vi "Version1z.vi"() -> ()   [LabVIEW 2019]
doc: "This is the interface, the one VI which loads all the others. Run this one first.\n\n(the line below ensures settings are saved)\n[Red Tweezers Save Settings]"
uses:
  plugins/subvis/line_trapping.ctl
  plugins/subvis/spot.ctl
  <vilib>/userDefined/High Color/IMAQdx.ctl
  plugins/subvis/selection_element.ctl
  <vilib>/Analysis/Matrix/Datatypes/RealMatrix.ctl
  plugins/subvis/mouse_info.ctl
  <vilib>/Analysis/baseanly.llb/Real A x B.vi
  plugins/subvis/red_tweezers_globals_INTERNAL_VOLATILE.vi
  plugins/subvis/red_tweezers_globals.vi
  <vilib>/Analysis/Matrix/Numeric/Multiply/Multiply - RM,R.vi
  <vilib>/Analysis/NI_AALBase.lvlib
  <vilib>/vision/driver/NI_Vision_Acquisition_Software.lvlib
  <vilib>/vision/NI_Vision_Development_Module.lvlib
  <vilib>/Analysis/Matrix/NI_Matrix.lvlib
panel:
  out "Objects":T1(array[cluster]) {"Aspect Ratio" format="%.2f"; "Orientation" format="%.2f"; "Area" format="%.2f"; "Object Center"."Y" format="%.2f"; "Object Center"."X" format="%.2f"}
  out "Specific Point 2":cluster{i32, i32}
  out "Specific Point":cluster{i32, i32}
  out "bottomrx 3":dbl
  out "toply 3":dbl
  out "bottomry 3":dbl
  out "toplx 3":dbl
  out "Circles 2":T2(array[cluster]) {"Position"."Y" format="%.2f"; "Position"."X" format="%.2f"}
  out "Spot Storage":T3[](array[typedef]) {"Amplitude Correction" step=0.1; "Line Trapping"."Phase Gradient" step=0.05; "Line Trapping"."Vector"."x" step=1e-06 format="%#_6p"; "Line Trapping"."Vector"."y" step=1e-06 format="%#_6p"; "Line Trapping"."Vector"."z" step=1e-06 format="%#_6p"; "NA Position"."r" step=1e-06; "NA Position"."y" step=1e-06; "NA Position"."x" step=1e-06; "Position"."z" step=1e-06; "Position"."y" step=1e-06; "Position"."x" step=1e-06; "Phase" step=0.7753; "Intensity" step=0.1}
  out "# selected":i16
  out "Last Pattern":T3[](array[typedef]) {"Amplitude Correction" step=0.1; "Line Trapping"."Phase Gradient" step=0.05; "Line Trapping"."Vector"."x" step=1e-06 format="%#_6p"; "Line Trapping"."Vector"."y" step=1e-06 format="%#_6p"; "Line Trapping"."Vector"."z" step=1e-06 format="%#_6p"; "NA Position"."r" step=1e-06; "NA Position"."y" step=1e-06; "NA Position"."x" step=1e-06; "Position"."z" step=1e-06; "Position"."y" step=1e-06; "Position"."x" step=1e-06; "Phase" step=0.7753; "Intensity" step=0.1}
  out "Plugins":T5(array[cluster])=[{"Name"="ASI Stage", "Folder"=path "C:/Users/Richard Bowman/Dropbox/red_tweezers_1_4_rc4/plugins/ASI Stage.llb", "vi reference"=refnum, "Needs to be run"=TRUE, "Error"={"status"=FALSE, "code"=0, "source"=""}}, {"Name"="iTweezers", "Folder"=path "C:/Users/Richard Bowman/Dropbox/red_tweezers_1_4_rc4/plugins/iTweezers.llb", "vi reference"=refnum, "Needs to be run"=TRUE, "Error"={"status"=FALSE, "code"=0, "source"=""}}, {"Name"="MightexLED", "Folder"=path "C:/Users/Richard Bowman/Dropbox/red_tweezers_1_4_rc4/plugins/MightexLED.llb", "vi reference"=refnum, "Needs to be run"=TRUE, "Error"={"status"=FALSE, "code"=0, "source"=""}}]
  in  "Tab":T6(tab)
  out "Object MP Y":dbl
  out "Object MP X":dbl
  out "ROI Point 3":T7
  out "Numeric 3":dbl
  out "Numeric 2":dbl
  in  "ROI points":dbl
  out "ROI Y":dbl
  out "ROI X":dbl
  out "Center Y":dbl
  out "Center X":dbl
  in  "Camera Capture 2":bool
  out "Bubble y 2":dbl
  out "Bubble x 2":dbl
  out "Number of Matches Returned":dbl
  out "bottomry 2":dbl
  out "toply 2":dbl
  out "bottomrx 2":dbl
  out "toplx 2":dbl
  in  "Send Data":bool
  out "Camera 3":T8(plugin-control)
  in  "Circle Descriptor 2":cluster{"Min Radius":dbl, "Max Radius":dbl}={"Min Radius"=3.0, "Max Radius"=500.0}
  out "Radius":dbl
  in  "Settings":T9={"Objects"=0, "Threshold"=128, "Reject Border"=FALSE, "Fill Holes"=FALSE, "Min Object Size"=FALSE, "Min Size"=3, "Max Object Size"=FALSE, "Max Size"=100, "Show Search Area"=FALSE, "Show Center"=TRUE, "Show Bounding Box"=TRUE} {"Objects" items=["Bright Objects", "Dark Objects"]; "Threshold" min=1 max=999999999 step=1; "Max Size" min=1 max=999999999 step=1; "Min Size" min=1 max=999999999 step=1}
  out "Number of Objects":i32
  in  "ROI switch":bool
  out "# of pairs":dbl
  out "1spot X":dbl
  out "1spot Y":dbl
  out "2spot X":dbl
  out "2spot Y":dbl
  out "NewX1":dbl
  out "NewY1":dbl
  out "NewX2":dbl
  out "NewY2":dbl
  out "Step Calculation X1":dbl
  out "Step Calculation Y1":dbl
  out "Step Calculation X2":dbl
  out "Step Calculation Y2":dbl
  out "Possible Collision":bool
  out "Play Pressed":bool
  out "Y":dbl
  out "X":dbl
  in  "O Button":bool
  in  "OK Button":bool
  in  "Bubble Size":dbl=50.0002
  out "Hit Indicator":bool
  in  "On":bool
  out "Induce check":bool
  out "Area+ Buffer":dbl
  in  "Area to check":dbl=0.00025
  out "Prev Current Spot":dbl
  out "spots selected 2":i32=4
  out "Spot # Check":dbl
  out "Orig Y SC":dbl
  out "Orig X SC":dbl
  out "ID num check":dbl
  out "Value Check":dbl
  out "ID":dbl[](array[numeric])
  out "Null array":dbl[](array[numeric])
  out "Potential Collisions":dbl
  out "What to Check":dbl[](array[numeric])
  out "Num":dbl
  out "Old Y":dbl
  out "Old X":dbl
  out "init":dbl
  out "Looper":bool
  in  "Output to SLM":bool
  out "Maximum":dbl
  out "Projected Distance":dbl
  out "Previous Distance":dbl
  out "Group ID #":dbl
  in  "Buffer Zone":dbl=7e-05
  out "# of Spots":dbl
  out "Distance":dbl
  out "Hit":bool
  out "Y Displacement":dbl
  out "X Displacement":dbl
  out "Current Spot #":dbl
  out "spots selected":i32=4
  in  "lock aspect ratio":bool=TRUE
  in  "Size":cluster{"x":dbl, "y":dbl, "z":dbl} {"z" step=1e-06 format="%#_4p"; "y" step=1e-06 format="%#_4p"; "x" step=1e-06 format="%#_4p"}
  in  "Position":cluster{"x":dbl, "y":dbl, "z":dbl}={"x"=1e-06, "y"=-6.3e-06, "z"=0.0} {"z" step=1e-06 format="%#_4p"; "y" step=1e-06 format="%#_4p"; "x" step=1e-06 format="%#_4p"}
  in  "phase":dbl step=0.7753
  in  "Vortex Charge":i8
  in  "Intensity":dbl=1.0 step=0.1
  in  "add to selection":bool
  in  "random position":bool
  in  "new spot":bool
  in  "delete":bool
  in  "New location\n ROI":bool
  out "Radius ROI x6":dbl
  out "Radius ROI y6":dbl
  out "Radius ROI y5":dbl
  out "Radius ROI x5":dbl
  out "Radius ROI y4":dbl
  out "Radius ROI x4":dbl
  out "Radius ROI y3":dbl
  out "Radius ROI x3":dbl
  out "Radius ROI x2":dbl
  out "Radius ROI y2":dbl
  out "Radius ROI y1":dbl
  out "Radius ROI x1":dbl
  out "Caging Radius \nToo Big":bool
  in  "Caging Radius":dbl
  out "ROI Point 1":T7
  out "ROI Point 0":T7
  out "ROI Point 2":T7
  in  "New Center Y":dbl
  in  "New Center X":dbl
  out "Delta x":dbl[](array[numeric])
  out "Delta y":dbl[](array[numeric])
  in  "Input New \nObject Location":bool
  out "Time Elapsed(ms)":i32
  out "Start":i32
  out "Stop":i32
  out "Insert End":bool
  out "NewXYRates":dbl[][](array[numeric])
  out "NewXYArraySize":dbl
  out "NewXYArray":dbl[][](array[numeric])
  in  "Rates":dbl
  out "LCS Y":dbl
  out "LCS X":dbl
  in  "LCS":dbl
  in  "Play":bool
  out "Initiate Creation":dbl
  in  "Max Number \nof Bubbles":dbl
  in  "Number of Planned\nSequence Frames":dbl
  in  "Add Additional Frames":bool
  in  "Frame Location":dbl
  in  "Additional Frames Wanted":dbl
  in  "rotate":bool
  in  "Rotation Axis":u16(ring)=2 items=["Z", "X", "Y", "Custom"]
  in  "Angle (degrees)":dbl=2.0
  in  "Custom Axis":cluster{dbl, dbl, dbl}
  in  "Spot Shape":enum32{"Normal", "Line", "NA", "Mixed"}(tab)=enum."Mixed"
  in  "Line Trapping":T4 {"Phase Gradient" step=0.05; "Vector"."x" step=1e-06 format="%#_4p"; "Vector"."y" step=1e-06 format="%#_4p"; "Vector"."z" step=1e-06 format="%#_4p"}
  in  "Scale back aperture":dbl=1.1 step=0.1
  in  "Scale BA":bool
  in  "Position on back aperture":cluster{"x":dbl, "y":dbl}={"x"=-5.84327907697451e-18, "y"=0.0} {"y" step=0.1 format="%#_4p"; "x" step=0.1 format="%#_4p"}
  in  "Radius on back aperture":dbl=1.1 step=0.1
  in  "Generate":bool
  in  "Pattern":T10(tab)
  in  "Spots across centre":i32=5
  in  "Reference Array?":bool
  in  "Fraction of SLM":dbl=1.0
  in  "Spots across centre":i32=5
  in  "N":cluster{i32, i32}
  in  "spacing/m":dbl=2.0
  in  "Iterations":i32=10
  out "non-uniformity":dbl(slide)=0.031119223416512406 scale=0.0..0.2
  out "efficiency":dbl(slide)=0.8985936267644501 scale=0.0..1.0
  in  "Optimise":bool
  in  "Reset Phase/Amplitude":bool
  in  "Fall-off/m":dbl=0.00025 min=0.0 step=1e-06 format="%#_4p"
  in  "Abort Plugin":bool
  in  "Plugin:":u16(ring)=1
  in  "Save Video":bool
  in  "Global ROI (requires restart)":i32[](array[numeric])=[0, 0, 1280, 512]
  in  "Zoom":bool
  in  "Draw ROI":bool
  in  "Zoom to Fit":bool
  out "Image Information":string="640x480 1.93X 8-bit image 255    (0,0)"
  in  "Camera":T11
  in  "Time per Frame (ms)":dbl
  in  "Edit Sequence Mode":bool
  in  "Manual Edit":bool
  in  "Bubble ID to Empty":dbl
  in  "Clearance Button":bool
  in  "Manual Sequence":bool
  in  "Play Sequence":bool
  in  "Reset":bool
  out "Sequence Instances":dbl
  out "Counter":dbl
  in  "Save State":bool
  out "Sequence On?":bool
  in  "Sequence Order":dbl
  out "Selection/Group":T12[](array[typedef])
  in  "Sequence Storer":T3[][](array[typedef]) {"Amplitude Correction" step=0.1; "Line Trapping"."Phase Gradient" step=0.05; "Line Trapping"."Vector"."x" step=1e-06 format="%#_6p"; "Line Trapping"."Vector"."y" step=1e-06 format="%#_6p"; "Line Trapping"."Vector"."z" step=1e-06 format="%#_6p"; "NA Position"."r" step=1e-06; "NA Position"."y" step=1e-06; "NA Position"."x" step=1e-06; "Position"."z" step=1e-06; "Position"."y" step=1e-06; "Position"."x" step=1e-06; "Phase" step=0.7753; "Intensity" step=0.1}
  in  "Tab Control":enum32{"Line", "Arc"}(tab)
  out "X Rate":dbl
  out "Y Rate":dbl
  out "Degree Rate":dbl
  out "Radians":dbl
  out "Center Y":dbl
  out "Center X":dbl
  in  "Radius X":dbl
  in  "Theta":dbl
  in  "Lock Current Spot":bool
  out "Locked Current Spot":dbl
  out "Numeric":dbl
  out "probe":dbl
  in  "Insert":bool
  in  "Start at Which Frame?":dbl
  out "Original Y":dbl
  out "Original X":dbl
  in  "Mark Original Position":bool
  in  "How Many Frames?":dbl
  out "New Y":dbl
  out "New X":dbl
  out "Spot Storage 2":T3[](array[typedef]) {"Amplitude Correction" step=0.1; "Line Trapping"."Phase Gradient" step=0.05; "Line Trapping"."Vector"."x" step=1e-06 format="%#_6p"; "Line Trapping"."Vector"."y" step=1e-06 format="%#_6p"; "Line Trapping"."Vector"."z" step=1e-06 format="%#_6p"; "NA Position"."r" step=1e-06; "NA Position"."y" step=1e-06; "NA Position"."x" step=1e-06; "Position"."z" step=1e-06; "Position"."y" step=1e-06; "Position"."x" step=1e-06; "Phase" step=0.7753; "Intensity" step=0.1}
  in  "Save":bool
  in  "Load":bool
  out "Video Frame Rate":dbl(knob)=50.00000000000003 scale=0.0..100.0 scale format="%.1f"
  out "Interface Frame Rate":dbl(knob)=97.23240312927678 scale=0.0..100.0 scale format="%.1f"
  in  "stop":bool=TRUE
  in  "Spots":dbl
  out "ROI new MPx":dbl
  out "ROI new Mpy":dbl
  out "3spot Y":dbl
  out "3spot X":dbl
  out "ROI y6":dbl
  out "ROI x6":dbl
  out "ROI y5":dbl
  out "ROI x5":dbl
  out "ROI y4":dbl
  out "ROI x4":dbl
  out "ROI y3":dbl
  out "ROI x3":dbl
  out "ROI y2":dbl
  out "ROI x2":dbl
  out "ROI y1":dbl
  out "ROI x1":dbl
  out "ROI Point 6":T7
  out "ROI point 5":T7
  out "ROI Point 4":T7
  out "MOP pressed":bool
  out "MOP pressed After":bool
  out "X Pos every 10 sec":dbl
  out "Elapsed Time":dbl
  out "Position Indicator":string
  out "Spot Checker":T3[](array[typedef]) {"Amplitude Correction" step=0.1; "Line Trapping"."Phase Gradient" step=0.05; "Line Trapping"."Vector"."x" step=1e-06 format="%#_6p"; "Line Trapping"."Vector"."y" step=1e-06 format="%#_6p"; "Line Trapping"."Vector"."z" step=1e-06 format="%#_6p"; "NA Position"."r" step=1e-06; "NA Position"."y" step=1e-06; "NA Position"."x" step=1e-06; "Position"."z" step=1e-06; "Position"."y" step=1e-06; "Position"."x" step=1e-06; "Phase" step=0.7753; "Intensity" step=0.1}
  out "Image":T8(plugin-control)
  # "Notes:\n\nIf you are doing non-sequence controls,\nthe delete function can be used as intended.\nHowever, do not use the delete function after\nrunning a sequence! Using it will prevent\nthe bubbles from appearing as the\nnumber of spots will change, which is\nessential for the sequence to work (it would\nbe displaying the maximum number of\nbubbles). \n\nIf you happen to delete a bubble, it can be \nrestored by inserting a new spot. Once enough\nspots have been restored, click on manual edit\nto correct the # of spots tracker. It should \nbe restored to where it originally was."
  # "The SLM can be used to shape spots; here you can restrict the NA of a spot (so it comes only from part of the back aperture), or create a line-trap"
  # "The traps do not have any spot-shaping applied (so they should just be diffraction-limited focal spots)."
  # "This shapes the amplitude (and phase) of the beam to create extended line traps.  The \"Phase Gradient\" control allows the Poynting vector to push things along the line.  Unfortunately, some work is needed on the scaling factors so the phase gradient control will need tweaking if the line trap has a nonzero z component."
  # "By default,each spot comes from the whole back aperture.  Here, you can limit a spot to come from a specific part of the back aperture."
  # "The control below allows you to scale the whole back aperture (i.e. the position and size of all the apertures).  It's a one-time operation, i.e. only changes things when you push \"ok\"."
  # "A Combination of line-trapping and NA restriction has been applied to these traps.  You can get at the line trap or NA parameters on the other tabs, switching to the NA tab does not delete the line-trap settings."
  # "This tab generates Shack-Hartmann type holograms, which are often useful when aligning the system, and arrays of spots."
  # "The controls above only work when using the \"IMAQdx with ROI Buttons\" case in the bottom loop.  You can save video regardless of camera code though."
  # "Manual Edit allows a user to\ngo to a specific sequence frame."
  # "To clear the sequence, you must\nclear the array. Right click on sequence\nstorer to do this."
  # "Use this to \"clear\" a \nspecific bubble. If\nworking on a sequence,\nuse this as your delete\nbutton! You can update\nthe view by using manual edit."
  # "Use the reset button\nto clear counter.\nIt becomes necessary\nwhen you clear the array,\nespecially in manual mode."
  # "Use the sequence creator tab to specify the\nnumber of bubbles you want along with\nthe number of frames.\n\nTo save at a specific interval, the sequence\norder can be used to place the state. If used\nto correct something, it will replace the\nentire sequence frame.\n\n\"Sequence On?\" is only used in auto mode."
  # "Multiple bubbles can  be done with the\nline function. One bubble at a time for the arc\nfunction."
  # "Using the Load/Save function:\n\nRed Tweezers itself is unable to save long \nsequences, but a separate program is able to\naccomplish this. To do this, follow these\nsteps:\n\n1. After creating your sequence, press the save\nbutton below.\n\n2. Then, go to the subvi folder and find\nSequenceSaver.vi.\n\n3. At the control \"Sequence Storer,\" right-click\nthe dimensions part of the array and go to\ndata operations.\n\n4. Press \"Make Current Values Default\" and save\nthe sequence.\n\n5. The next time you load the program, simply\npress load to re-acquire the sequence. You\nwill need to insert the bubbles again, but after\nthe first frame can be recovered by using\nSequenceControl.vi."
types:
  T1 = cluster{"Object Center":cluster{"X":sgl, "Y":sgl}, "Bounding Box":cluster{"X Left":i32, "Y Top":i32, "X Right":i32, "Y Bottom":i32}, "Area":sgl, "Orientation":sgl, "Aspect Ratio":sgl, "Nb Holes":i32}[]
  T2 = cluster{"Position":cluster{"X":sgl, "Y":sgl}, "Radius":dbl, "Score":dbl}[]
  T3 = typedef "spot.ctl" = cluster{"Position":cluster{"x":dbl, "y":dbl, "z":dbl}, "Intensity":dbl, "Vortex Charge":i8, "Phase":dbl, "NA Position":cluster{"x":dbl, "y":dbl, "r":dbl}, "Line Trapping":T4, "Amplitude Correction":dbl}
  T4 = typedef "line_trapping.ctl" = cluster{"Vector":cluster{"x":dbl, "y":dbl, "z":dbl}, "Phase Gradient":dbl}
  T5 = cluster{"Name":string, "Folder":path, "vi reference":refnum<vi>, "Needs to be run":bool, "Error":errorcluster}[]
  T6 = enum32{"Image Process", "Current Spot", "Sequence Creator", "Rotate", "Spot Shape", "Patterns", "Plugins", "Video", "Sequence", "Spot Control", "Load/Save"}
  T7 = typedef "NI_Matrix.lvlib/RealMatrix.ctl" = dbl[][]
  T8 = typedef "IMAQ Image.ctl" = refnum<image>
  T9 = cluster{"Objects":u16, "Threshold":i32, "Reject Border":bool, "Fill Holes":bool, "Min Object Size":bool, "Min Size":i32, "Max Object Size":bool, "Max Size":i32, "Show Search Area":bool, "Show Center":bool, "Show Bounding Box":bool}
  T10 = enum32{"HCP Shack-Hartmann", "Square Shack-Hartmann", "Rectangular Grid"}
  T11 = typedef "IMAQdx.ctl" = refnum<k21>
  T12 = typedef "selection_element.ctl" = cluster{"Group ID":i32, "Selected":bool}
  T13 = typedef "mouse_info.ctl" = cluster{"Button Down":bool, "Dragging":bool, "Position (Image Pixels)":cluster{"X":dbl, "Y":dbl}, "Previous Position (Image Pixels)":cluster{"X":dbl, "Y":dbl}, "Button":u16, "Mods":cluster{"Double Click":bool, "Menu Key":bool}, "PlatMods":cluster{"Shift":bool, "Ctrl":bool, "Alt":bool, "Cmd":bool, "Opt":bool}}
  T14 = cluster{"Desired Font (Application)":enum16{"User-specified Font", "Application Font", "System Font", "Dialog Font"}, "[User-specified Font]":cluster{"Font Name":string, "Size":i16, "Strikeout?":bool, "Italic?":bool, "Underline?":bool, "Outline?":bool, "Shadow?":bool, "Bold?":bool, "Rotation Angle":dbl}, "Horizontal Alignment":i16, "Vertical Alignment":i16}
  T15 = cluster{"Position":cluster{"x":dbl, "y":dbl, "z":dbl}, "Intensity":dbl, "Vortex Charge":i8, "Phase":dbl, "NA Position":cluster{"x":dbl, "y":dbl, "r":dbl}, "Line Trapping":T4, "Amplitude Correction":dbl}
  T16 = enum16{"Set guide visibility", "Set grid visibility", "Show front panel", "Render on image"}
  T17 = enum32{"Current Spot", "Rotate", "Spot Shape", "Patterns", "Plugins", "Video"}
  T18 = enum16{"Left Button", "Center Button", "Right Button", "Window Close"}
  T19 = typedef "Image Type" = u32
  T20 = cluster{"number: 0 to 1":dbl, "number: 0 to 1":dbl}
  T21 = typedef "overlay_element.ctl" = cluster{"Tool":enum16{"Lines", "Oval", "Rectangle", "Text"}, "Points":cluster{"X":dbl, "Y":dbl}[], "Drawing Mode":u32, "Color":u32, "String":string}
  T22 = enum32{"Current Spot", "Rotate", "Spot Shape", "Patterns", "Plugins", "Video", "Particle Tracking", "Clamping", "Blank"}[]
  T23 = typedef "LVMenuShortCut.ctl" = cluster{"include Shift key?":bool, "include Ctrl key?":bool, "shortcut key":string}
  T24 = typedef "LVPoint32TypeDef.ctl" = cluster{"Horizontal":i32, "Vertical":i32}
  T25 = cluster{"Shift":bool, "Ctrl":bool, "Alt":bool, "Cmd":bool, "Opt":bool}
  T26 = cluster{"Button Down":bool, "Dragging":bool, "Mouse Coords (image pixels)":cluster{dbl, dbl}, "Mouse Coords (image pixels)":cluster{dbl, dbl}, "Button":u16, "Mods":cluster{"Double Click":bool, "Menu Key":bool}, "PlatMods":cluster{"Shift":bool, "Ctrl":bool, "Alt":bool, "Cmd":bool, "Opt":bool}}
  T27 = cluster{"Global Rectangle":i32[], "Contours":cluster{"Contour Type":u32, "ROI Type":u32, "Points":i32[]}[]}
  T28 = cluster{"Contour Type":u32, "ROI Type":u32, "Points":i32[]}[]
  T29 = cluster{"Position":cluster{"X":sgl, "Y":sgl}, "Radius":dbl, "Score":dbl}
  T30 = cluster{"Contour Type":u32, "ROI Type":u32, "Points":i32[]}
  T31 = cluster{"[0]":dbl, "[1]":dbl, "[2]":dbl, "[3]":dbl}
  T32 = cluster{"Object Center":cluster{"X":sgl, "Y":sgl}, "Bounding Box":cluster{"X Left":i32, "Y Top":i32, "X Right":i32, "Y Bottom":i32}, "Area":sgl, "Orientation":sgl, "Aspect Ratio":sgl, "Nb Holes":i32}
  T33 = cluster{"NewXYArray[0]":dbl, "NewXYArray[1]":dbl, "NewXYArray[2]":dbl, "NewXYArray[3]":dbl, "NewXYArray[4]":dbl, "NewXYArray[5]":dbl, "NewXYArray[6]":dbl, "NewXYArray[7]":dbl, "NewXYArray[8]":dbl}
  T34 = cluster{"Average Frame Time":dbl, "millisecond timer value":u32}
  T35 = cluster{"Position":cluster{"x":dbl, "y":dbl, "z":dbl}, "Intensity":dbl, "Vortex Charge":i8, "Phase":dbl, "NA Position":cluster{"x":dbl, "y":dbl, "r":dbl}, "Line Trapping":T4, "Amplitude Correction":dbl}[]
  T36 = enum32{"Bad", "Idle", "Run top level", "Running"}
  T37 = typedef "AviRefnum.ctl" = refnum<k1>
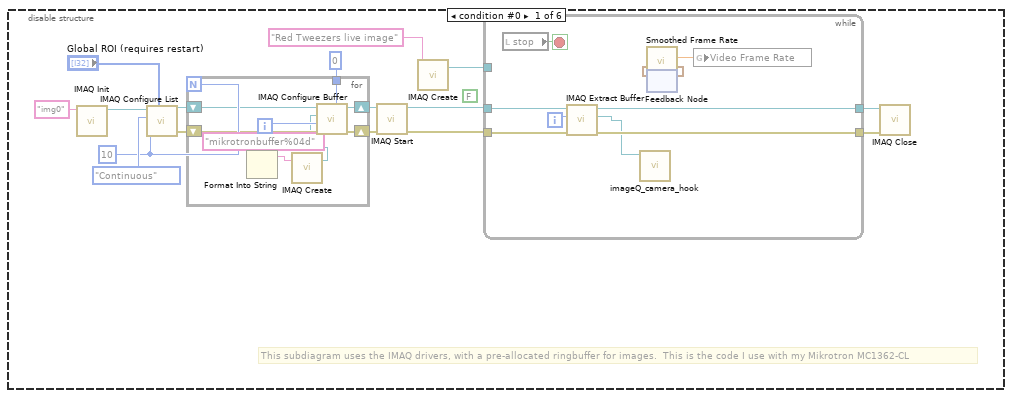
[diagram p3: hidden frame]
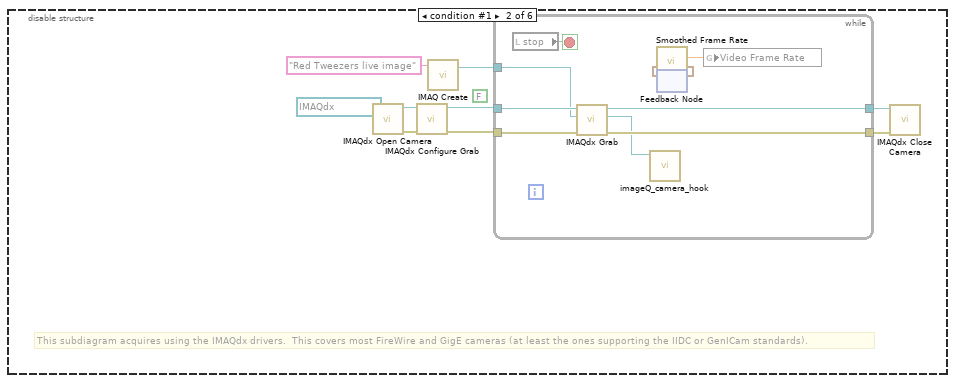
[diagram p4: hidden frame]
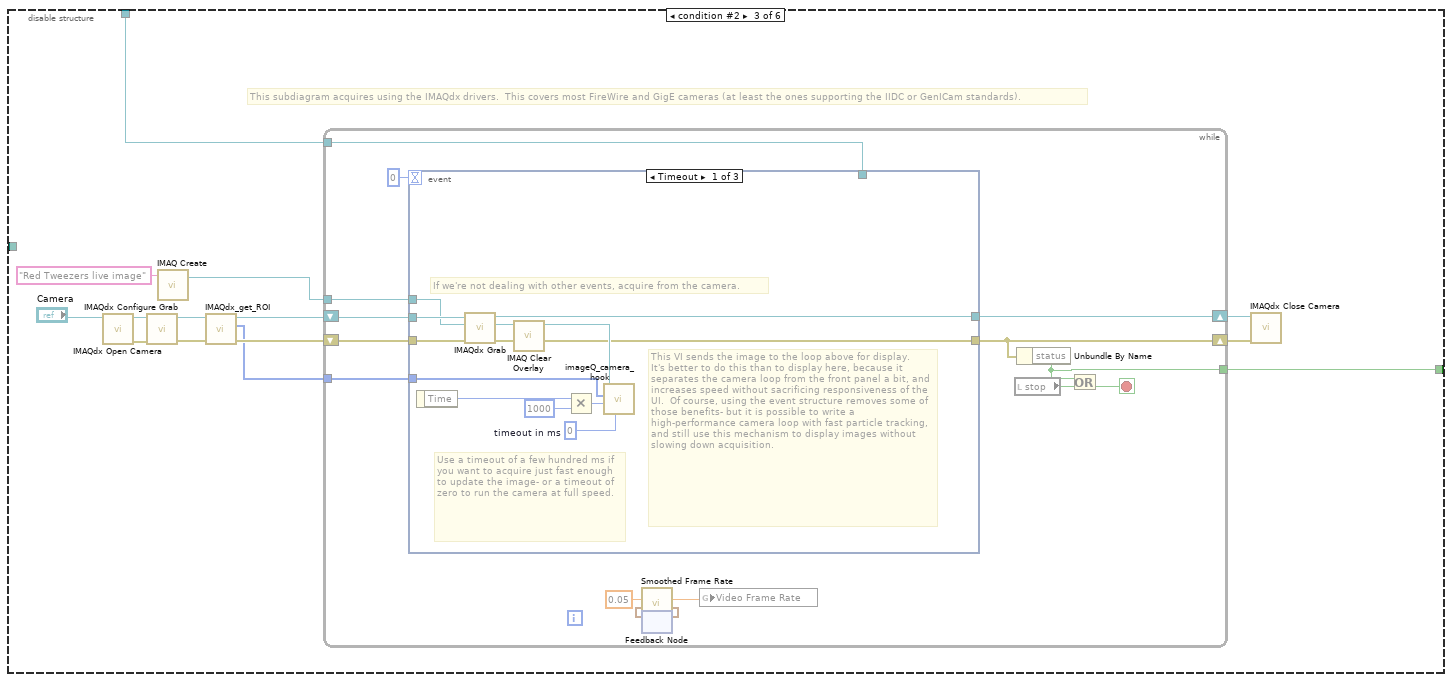
[diagram p5: hidden frame]
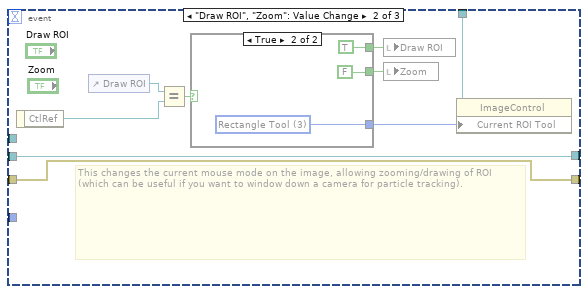
[diagram p6: hidden frame]
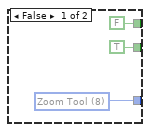
[diagram p7: hidden frame]
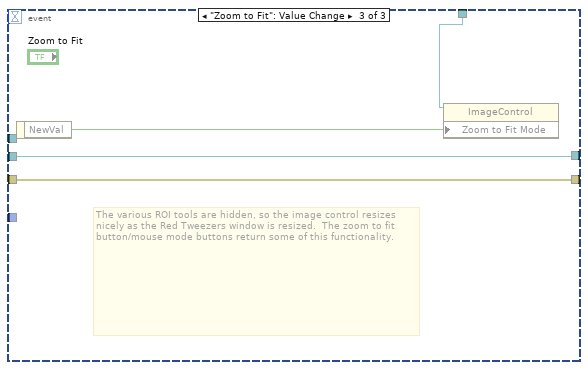
[diagram p8: hidden frame]
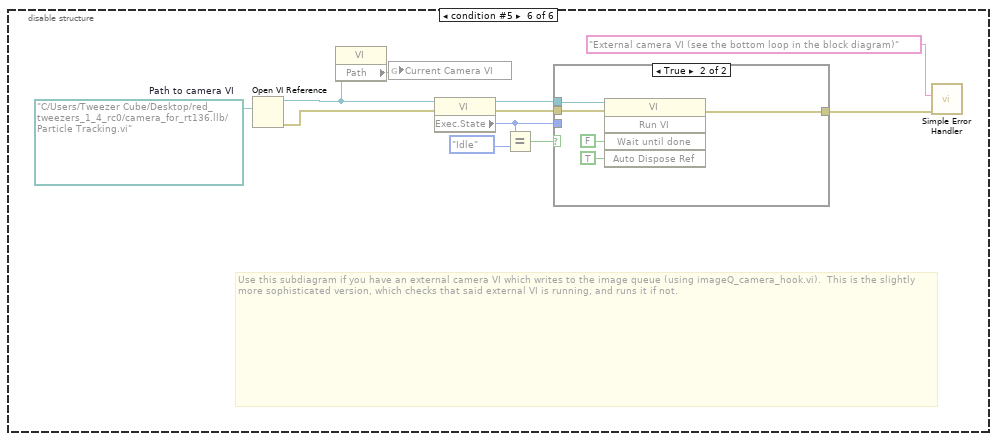
[diagram p10: hidden frame]
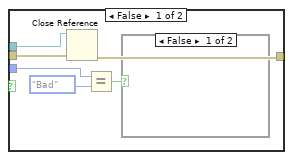
[diagram p11: hidden frame]
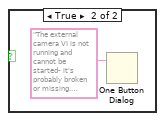
[diagram p12: hidden frame]
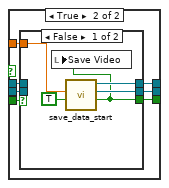
[diagram p14: hidden frame]
diagram:
  w11 = "red_tweezers_display_imageQ" ("Queue Name")
  w23 = T13 {"Button Down"=FALSE, "Dragging"=FALSE, "Position (Image Pixels)"={"X"=0.0, "Y"=0.0}, "Previous Position (Image Pixels)"={"X"=0.0, "Y"=0.0}, "Button"=0, "Mods"={"Double Click"=FALSE, "Menu Key"=FALSE}, "PlatMods"={"Shift"=FALSE, "Ctrl"=FALSE, "Alt"=FALSE, "Cmd"=FALSE, "Opt"=FALSE}}  # Mouse Information
  w24 = refnum<vi> refnum  # Image
  # "The funny looking feedback-node structure is deliberate (if odd).  We want to reload settings from the last used file (stored in the registry) only if this program has not been run since it was last loaded from file/recompiled.  That's why I use an uninitialised shift register: every time the program runs, it increments.  So, if it is zero, this is our first run (or we've been recently recompiled)."
  # "This loop handles the video that is displayed on-screen and saved to file."
  # "Initially, we only register to be told when the user clicks the image"
  # "This is the actual image control"
  # "This is a generic reference.\nIt is just a placeholder, so we can register for events later."
  # "This version of red tweezers uses two coordinate systems: \n1. Real Coordinates - corresponding to physical distances in 3D in microns\n2. Image Coordinates - position on the camera image, relative to the top left of the CURRENT ROI, measured in pixels. If the ROI changes, the relationship between \"real units\" and \"image pixels\" may change, so all values should be stored and presented to the user in REAL units unless there is a good reason to do otherwise."
  n1 = control-ref of="Plugin Pnl"() -> (w20:refnum<vi>)
  n2 = flat-sequence {
    tunnel: [w27] -> w6
    tunnel: w4 -> [_]
    frame #0 {
      n3 = vi-ref "red_tweezers_globals_INTERNAL.vi"() -> (w28:refnum<vi>)
      n4 = property class="VI"(reference=w28) -> ("Path"=w27:path)  [unwired: 1 in, 2 out]
      n5 = global write "red_tweezers_globals_INTERNAL_VOLATILE.vi" "Current Camera VI"(w27) -> ()
    }
  }
  n6 = control-ref of="Plugin:"() -> (w21:refnum<vi>)
  n7 = feedback #1() -> (w14:dbl)  [unwired: 1 in]
  n8 = Equal To 0?(x=w14) -> (x = 0?=w13:bool)
  n9 = Increment(x=w14) -> (x+1=w12:dbl)
  n10 = feedback-in #1(w12) -> ()
  n11 = call "plugins_load.vi"("Sub Panel"=w20, "Plugin Chooser"=w21) -> ("error out"=w15:errorcluster, "Plugins"=w17:T5)  [unwired: 2 in, 2 out]
  "Plugins" <- w17
  n12 = control-ref of="Image"() -> (w5:refnum<vi>)
  n13 = case shown="True" w13 {
    tunnel: w15 -> [_ w29]
    tunnel: [_ w29] -> w4
    frame False {
    }
    frame True {
      n14 = call "settings_load_default_file.vi"("error out"=w29) -> ()
    }
  }
  n15 = flat-sequence {
    tunnel: w4 -> [_]
    tunnel: w2 -> [w31]
    frame #0 {
      # "ensure we don't accidentally start saving video, and run UDP Sender to set up the hologram window."
      n16 = local write "Save Video"(FALSE ("background subtraction")) -> ()
      n17 = call "UDP Sender generic_2.vi"("Spots"=w31) -> ()  [unwired: 2 in, 1 out]
    }
  }
  n18 = global read "red_tweezers_globals.vi" "Selection/Group"() -> (w22:T12[])
  n19 = register-events(w5, w24, w24, w24) -> (reference out=w25:refnum<event-registration>)  [unwired: 2 in, 1 out]
  n20 = global read "red_tweezers_globals.vi" "Spots"() -> (w2:T3[])
  n21 = local write "stop"(FALSE ("STOP")) -> ()
  n22 = call "ensure_selection_matches_spots.vi"("Selection and Groups in"=w22, "Spots"=w2) -> ("Selection and Groups out"=w26:T12[], "Spots (duplicate)"=w1:T3[])  [unwired: 4 in]
  n23 = call "IMAQ Create"("Image Name"=w11) -> ("New Image"=w9:T8)  [unwired: 4 in, 1 out]
  n24 = call "imageQ_create_return_queue.vi"("Queue Name"=w11) -> ("queue out"=w10:refnum<queue>)
  n25 = while {
    shift-right: [w170] -> _
    shift-left: w1 -> [w190]
    shift-right: [w189] -> _
    shift-left: w26 -> [w188]
    shift-right: [w192] -> _
    shift-left: _ -> [w183]
    shift-right: [w191] -> _
    shift-left: _ -> [w182]
    tunnel: w5 -> [w187]
    shift-right: [w181] -> _
    shift-left: w23 -> [w180]
    shift-right: [w184] -> _
    shift-left: w25 -> [w185]
    border: errorcluster {"status"=FALSE, "code"=0, "source"=""} ("error out") -> [_]
    tunnel: [errorcluster {"status"=FALSE, "code"=0, "source"=""} ("error in (no error)")] -> w18
    border: w17 -> [_]
    tunnel: w1 -> [w171]
    stop <- w172 stop-if-true
    (unwired) 1 ("index")
    w88 = 7 items=["Red", "Green", "Blue", "Hue", "Saturation", "Luminance", "Value", "Intensity"] ("Color Plane")
    w90 = T19 0 items=["Grayscale (U8)", "Grayscale (I16)", "Grayscale (SGL)", "Complex (CSG)", "RGB (U32)", "HSL (U32)", "RGB (U64)", "Grayscale (U16)"] ("Image Type")
    # "Collision Avoidance System"
    # "When done obtatining points\nKEEP it at 7!"
    # "Cycle through to obtain points"
    # "This is the calculation for the center of the detected circle, not sure where to put for now"
    # "This Play Function inserts bubbles from a given .mat file into the sequence storer"
    # "The function inserts the newly generated sequence for the automatic sequence generator. It also contains the code\nthe code necessary to check whether the bubbles will intersect with each other in the sequence."
    # "This calculates the size of the area including the buffer zone length.\nThe bubble diameter will also be included in the near future."
    # "The statement to the right controls the area that are being chcecked and checks\nwhich bubbles need to be checked.  There are two instances where this activates\nin this case:\n\nWhen a new bubble is selected\nWhen a bubble is deselected, reverting to the last current spot #\n\nThe other case, when the bubble moves out of the area specified, is located\ninside the while loop controlling the bubble movement with a mouse."
    # "Timer function example"
    # "These functions help with the calculations for the sequence generator."
    # "This loads the sequence from the \"saver\" VI. The save function below \"saves\" the sequence into the saver VI."
    # "The VI above is SequenceSaver.vi which contains the\ncode necessary to create a sequence."
    # "This case structure is the Save State structure. This stores\nthe current state of the bubbles (ie position)."
    # "Reset sets the counter back to zero. This is particularly useful \nwhen using the manual sequence."
    # "This case structure helps to continue the sequence.\nThis takes the true case of the Sequence On? function\nor the true case for the Manual Sequence function\nin order to go to the next sequence frame."
    # "This case structure allows for the playing of the sequence.\nThe amount of time it takes to go through the sequence\ncan be edited on the current spot menu."
    # "We only write to the image overlay when we are in one of the tabs, to prevent it disappearing when we are (for example) using the mouse."
    # "These wires control saving undo info. See the VI below's tip strips for details."
    # "Setting these wires to false means:\n(1) dragging moves the selection\n(2) clicking spots changes selection\nset them to true to stop the default mouse behaviour, don't wire them straight through!"
    n26 = event shown="[0] Timeout" {
      selector: w185 -> [w867 w1538 w1543 w1765 w1793 w1810 w1907 _]
      dyn-events: [w867 w1537 w1543 w1763 w1790 w1811 w1907 _] -> w184
      timeout: 0 -> [_ _ _ _ _ _ _ _]
      tunnel: [w875 _ w1545 w1760 w1795 w1802 w1894 _] -> w192
      tunnel: [w874 _ w1544 w1759 w1794 w1801 w1898 _] -> w191
      tunnel: [w873 _ _ _ _ _ _ _] -> w143
      tunnel: w190 -> [w872 w1533 w1550 w1755 w1788 w1807 w1902 w2225]
      tunnel: [w871 w1533 w1548 w1755 w1788 w1798 w1900 w2225] -> w178
      tunnel: [w870 w1532 w1547 w1744 w1787 w1808 w1890 w2224] -> w177
      tunnel: w188 -> [w869 w1532 w1549 w1744 w1787 w1806 w1901 w2224]
      tunnel: w187 -> [w868 w1534 w1540 w1754 w1791 w1809 w1903 _]
      tunnel: [w866 _ w1542 w1764 T13 {"Button Down"=FALSE, "Dragging"=FALSE, "Position (Image Pixels)"={"X"=0.0, "Y"=0.0}, "Previous Position (Image Pixels)"={"X"=0.0, "Y"=0.0}, "Button"=0, "Mods"={"Double Click"=FALSE, "Menu Key"=FALSE}, "PlatMods"={"Shift"=FALSE, "Ctrl"=FALSE, "Alt"=FALSE, "Cmd"=FALSE, "Opt"=FALSE}} T13 {"Button Down"=FALSE, "Dragging"=FALSE, "Position (Image Pixels)"={"X"=0.0, "Y"=0.0}, "Previous Position (Image Pixels)"={"X"=0.0, "Y"=0.0}, "Button"=0, "Mods"={"Double Click"=FALSE, "Menu Key"=FALSE}, "PlatMods"={"Shift"=FALSE, "Ctrl"=FALSE, "Alt"=FALSE, "Cmd"=FALSE, "Opt"=FALSE}} w1906 _] -> w181
      tunnel: w180 -> [w866 _ w1542 _ _ w1805 w1897 _]
      tunnel: w183 -> [_ _ w1545 w1760 w1795 w1802 w1894 _]
      tunnel: w182 -> [_ _ w1544 w1759 w1794 w1801 w1898 _]
      tunnel: [w865 _ _ _ _ _ _ _] -> w179
      tunnel: [_ _ w1541 _ _ _ TRUE _] -> w176
      tunnel: [_ _ _ TRUE TRUE TRUE FALSE _] -> w175
      tunnel: [TRUE _ _ _ _ _ _ _] -> w173
      tunnel: [_ _ _ _ _ _ _ "stop"] -> w172
      tunnel: w171 -> [_ _ _ _ _ _ w1891 _]
      event Timeout {
        n27 = event-data() -> ()  [unwired: 1 in, 1 out]
        n28 = case shown="\"Current Spot\", Default" "Tab" {
          tunnel: [w890 w1158 w1305 w1407 w1488 w1526] -> w871
          tunnel: w872 -> [w887 w1160 w1306 w1409 w1488 w1526]
          tunnel: w869 -> [w876 w1159 w1303 w1408 w1487 w1525]
          tunnel: [w889 w1157 w1304 w1406 w1487 w1525] -> w870
          tunnel: [w877 _ TRUE _ _ _] -> w875
          tunnel: [w877 _ _ _ _ _] -> w874
          tunnel: [_ _ _ FALSE _ _] -> w873
          tunnel: w868 -> [_ _ _ _ _ w1522]
          tunnel: w866 -> [_ _ w1285 _ _ _]
          tunnel: [_ _ w1287 _ _ _] -> w865
          frame "Current Spot", Default {
            w877 = FALSE
            # "The function below contains the code necessary to use the automatic sequence generator to create specific movements. It also helps translate cases where the point is entered in not dragged.\nThis prevents bubbles from intersecting if the bubble is told not to intersect."
            # "If it's out of date, update front panel"
            n29 = call "find_centroid.vi"("Selection and Groups"=w876, "Spots"=w887) -> ("Mean Values"=w885:T3, "size"=w879:cluster{"x":dbl, "y":dbl, "z":dbl}, "centroid"=w880:cluster{"x":dbl, "y":dbl, "z":dbl}, "# selected"=w878:i16)  [unwired: 2 in, 1 out]
            n30 = stacked-sequence {
              tunnel: w878 -> [_ w892]
              frame #0 {
                n31 = local read "spots selected"() -> (→"spots selected 2":i32)
              }
              frame #1 {
                "spots selected" <- w892
              }
            }
            n32 = feedback-in #2(w885) -> ()
            n33 = feedback #2() -> (w886:T3)  [unwired: 1 in]
            n34 = feedback #3() -> (w884:cluster{"x":dbl, "y":dbl, "z":dbl})  [unwired: 1 in]
            n35 = feedback-in #3(w879) -> ()
            n36 = Not Equal?(x=w886, y=w885) -> (x != y?=w883:bool)
            n37 = Not Equal?(x=w884, y=w879) -> (x != y?=w882:bool)
            n38 = Or(x=w883, y=w882) -> (x .or. y?=w881:bool)
            n39 = case shown="True" w881 {
              tunnel: w885 -> [_ w898]
              tunnel: w879 -> [_ w894]
              frame False {
              }
              frame True {
                n40 = Unbundle By Name(w898) -> ("Position"=w893:cluster{"x":dbl, "y":dbl, "z":dbl}, "Intensity"=w896:dbl, "Vortex Charge"=w895:i8, "Phase"=w897:dbl)
                n41 = local write "Size"(w894) -> ()
                n42 = local write "Vortex Charge"(w895) -> ()
                n43 = local write "Intensity"(w896) -> ()
                n44 = local write "Position"(w893) -> ()
                n45 = local write "phase"(w897) -> ()
                n46 = Unbundle By Name(w893) -> ()  [unwired: 2 out]
              }
            }
            n47 = local write "Selection/Group"(w876) -> ()
            n48 = event shown="[3] \"Position\": Value Change" {
              selector: _ -> [_ _ _ _ _ _ _ _]
              dyn-events: _ -> [_ _ _ _ _ _ _ _]
              timeout: 10 -> [_ _ _ _ _ _ _ _]
              tunnel: w887 -> [w900 w904 w918 w941 w1045 w1090 w1116 w1139]
              tunnel: w876 -> [w899 w903 w921 w948 w1032 w1087 w1113 w1137]
              tunnel: [w900 w902 w919 w940 w1033 w1088 w1114 w1138] -> w890
              tunnel: [w899 w901 w920 w948 w1032 w1087 w1113 w1137] -> w889
              tunnel: w880 -> [_ _ _ _ w1044 _ _ _]
              event Timeout {
                n49 = event-data() -> ()  [unwired: 3 out]
              }
              event "delete": Value Change {
                n50 = event-data() -> ()  [unwired: 7 out]
                n51 = call "delete_selected_spots.vi"("Selection/Group 3"=w903, "Spots 3"=w904) -> ("Selection/Group 2"=w901:T12[], "Spots 2"=w902:T3[])  [unwired: 4 in]
              }
              event "new spot": Value Change {
                # "If we're not adding it to the selection, de-select all the other spots"
                n52 = event-data() -> ()  [unwired: 7 out]
                n53 = call "coords_ROI_currentimage.vi"() -> ("Mono ROI"=w905:i32[])
                n54 = case shown="False" "add to selection" {
                  tunnel: w921 -> [w934 w939]
                  tunnel: [w933 w939] -> w916
                  frame False {
                    n55 = for {
                      tunnel: w934 -> [w937] mode=indexing
                      tunnel: [w938] -> w933 mode=indexing
                      n56 = Unbundle(w937) -> ("Group ID"=w936:i32)  [unwired: 1 out]
                      n57 = Bundle(cluster=w937, "Group ID"=w936, "Selected"=FALSE ("Label.Visible")) -> (w938:T12)
                    }
                  }
                  frame True {
                  }
                }
                n58 = Index Array(array=w905) -> (element #1=w911:i32, element #2=w912:i32, element #3=w910:i32, element #4=w909:i32)  [unwired: 4 in]
                n59 = Bundle("Numeric"=w911, "Numeric"=w912) -> (w906:cluster{"Numeric":i32, "Numeric":i32})  [unwired: 1 in]
                n60 = Bundle("Numeric"=w910, "Numeric"=w909) -> (w908:cluster{"Numeric":i32, "Numeric":i32})  [unwired: 1 in]
                n61 = Subtract(x=w908, y=w906) -> (x-y=w907:cluster{"Numeric":i32, "Numeric":i32})
                n62 = case shown="True" "random position" {
                  tunnel: [w923 w929] -> w914
                  tunnel: w907 -> [_ w925]
                  tunnel: w906 -> [_ w924]
                  frame False {
                    n63 = call "replace_position.vi"("Position"=cluster{"x":dbl, "y":dbl, "z":dbl} {"x"=0.0, "y"=0.0, "z"=0.0}) -> ("Spot"=w923:T3)  [unwired: 1 in, 2 out]
                  }
                  frame True {
                    n64 = Random Number (0-1)() -> (number: 0 to 1=w931:dbl)
                    n65 = Random Number (0-1)() -> (number: 0 to 1=w932:dbl)
                    n66 = Bundle("number: 0 to 1"=w932, "number: 0 to 1"=w931) -> (w930:T20)  [unwired: 1 out]
                    n67 = Multiply(x=w930, y=w925) -> (x*y=w927:cluster{dbl, dbl})
                    n68 = Add(x=w927, y=w924) -> (x+y=w926:cluster{dbl, dbl})
                    n69 = call "coords_image_to_real_currentimage.vi"("Position (pixels on image)"=w926) -> ("Position (real coords)"=w928:cluster{dbl, dbl, "Z":dbl})  [unwired: 9 in]
                    n70 = call "replace_position.vi"("Position"=w928) -> ("Spot"=w929:T3)  [unwired: 1 in, 2 out]
                  }
                }
                n71 = Build Array (concatenate)(w918, w914) -> (w919:T3[])
                n72 = Build Array (concatenate)(w916, cluster{i32, "Label.Visible":bool} {0, "Label.Visible"=TRUE}) -> (w920:T12[])
              }
              event "Position": Value Change {
                # "If the position has changed, translate the spots"
                n73 = event-data() -> ("OldVal"=w946:cluster{"x":dbl, "y":dbl, "z":dbl}, "NewVal"=w947:cluster{"x":dbl, "y":dbl, "z":dbl})  [unwired: 5 out]
                n74 = flat-sequence {
                  tunnel: w948 -> [w952]
                  tunnel: w945 -> [w951]
                  tunnel: w941 -> [w950]
                  tunnel: [w949] -> w942
                  frame #0 {
                    n75 = for {
                      tunnel: w950 -> [w957] mode=indexing
                      tunnel: w952 -> [w954] mode=indexing
                      tunnel: [w956] -> w949 mode=indexing
                      tunnel: w951 -> [w955]
                      n76 = Unbundle(w954) -> ("Selected"=w953:bool)  [unwired: 1 out]
                      n77 = case shown="True" w953 {
                        tunnel: w957 -> [w958 w963]
                        tunnel: [w958 w962] -> w956
                        tunnel: w955 -> [_ w959]
                        frame False {
                        }
                        frame True {
                          n78 = call "extract_position.vi"("Spot"=w963) -> ("Position"=w960:cluster{"x":dbl, "y":dbl, "z":dbl})
                          n79 = Add(x=w960, y=w959) -> (x+y=w961:cluster{"x":dbl, "y":dbl, "z":dbl})
                          n80 = call "replace_position.vi"("Position"=w961, "Spot in"=w963) -> ("Spot"=w962:T3)  [unwired: 2 out]
                        }
                      }
                    }
                  }
                }
                n81 = Subtract(x=w947, y=w946) -> (x-y=w945:cluster{"x":dbl, "y":dbl, "z":dbl})
                n82 = local read "# of Spots"() -> (w944:dbl)
                n83 = stacked-sequence {
                  tunnel: w941 -> [_ w968 _]
                  tunnel: w942 -> [_ w967 _]
                  tunnel: w944 -> [_ w966 _]
                  tunnel: [_ _ w1015] -> w943
                  tunnel: w942 -> [_ _ w1014]
                  tunnel: w941 -> [_ _ w1013]
                  tunnel: [_ _ w1012] -> w940
                  frame #0 {
                    n84 = local write "Looper"(FALSE) -> ()
                    "init" <- 0
                  }
                  frame #1 {
                    n85 = for {
                      N: w966 -> [_]
                      tunnel: w968 -> [w973]
                      tunnel: w967 -> [w978]
                      stop <- w979 stop-if-true
                      n86 = local read "init"() -> (w972:dbl)
                      n87 = Index Array(array=w978, index=w972) -> (element=w977:T3)
                      n88 = Index Array(array=w973, index=w972) -> (element=w971:T3)
                      n89 = Unbundle By Name(w977) -> ("Position.x"=w976:dbl, "Position.y"=w975:dbl)
                      n90 = local read "# of Spots"() -> (w974:dbl)
                      n91 = Unbundle By Name(w971) -> ("Position.x"=→"Old X":dbl, "Position.y"=→"Old Y":dbl)
                      n92 = local write "New X"(w976) -> ()
                      n93 = local write "New Y"(w975) -> ()
                      n94 = stacked-sequence {
                        tunnel: w973 -> [w984 _]
                        tunnel: w976 -> [w983 _]
                        tunnel: w975 -> [w982 _]
                        tunnel: w974 -> [w981 _]
                        tunnel: w972 -> [w980 _]
                        frame #0 {
                          n95 = for {
                            N: w981 -> [_]
                            tunnel: w984 -> [w1006]
                            tunnel: w983 -> [w1005]
                            tunnel: w982 -> [w1003]
                            tunnel: w980 -> [w988]
                            i -> [w990]
                            stop <- w989 stop-if-true
                            n96 = Index Array(array=w1006, index=w990) -> (element=w1007:T3)
                            n97 = Unbundle By Name(w1007) -> ("Position.x"=w1004:dbl, "Position.y"=w1002:dbl)
                            n98 = Subtract(x=w1005, y=w1004) -> (x-y=w1001:dbl)
                            n99 = Subtract(x=w1003, y=w1002) -> (x-y=w1000:dbl)
                            n100 = Square(x=w1001) -> (x^2=w999:dbl)
                            n101 = Square(x=w1000) -> (x^2=w998:dbl)
                            n102 = local read "# of Spots"() -> (w992:dbl)
                            n103 = Add(x=w999, y=w998) -> (x+y=w997:dbl)
                            n104 = local read "Buffer Zone"() -> (w987:dbl)
                            n105 = Square Root(x=w997) -> (sqrt(x)=w996:dbl)
                            n106 = Multiply(x=2, y=w987) -> (x*y=w985:dbl)
                            n107 = Less?(x=w996, y=w985) -> (x < y?=w994:bool)
                            n108 = Not Equal?(x=w988, y=w990) -> (x != y?=w993:bool)
                            n109 = Equal?(x=w992, y=w990) -> (x = y?=w995:bool)
                            n110 = And(x=w993, y=w994) -> (x .and. y?=w991:bool)
                            "Looper" <- w991
                            n111 = Or(x=w991, y=w995) -> (x .or. y?=w989:bool)
                          }
                        }
                        frame #1 {
                          n112 = local read "Looper"() -> (w1008:bool)
                          n113 = case shown="False" w1008 {
                            frame False {
                              n114 = local read "init"() -> (w1009:dbl)
                              n115 = Add(x=w1009, y=1) -> (x+y=w1011:dbl)
                              n116 = local write "init"(w1011) -> ()
                            }
                            frame True {
                            }
                          }
                        }
                      }
                      n117 = local read "Looper"() -> (w979:bool)
                    }
                  }
                  frame #2 {
                    n118 = local read "Looper"() -> (w1016:bool)
                    n119 = case shown="True" w1016 {
                      tunnel: w1014 -> [w1020 _]
                      tunnel: w1013 -> [_ w1028]
                      tunnel: ["This is an acceptable entry." "ERROR: A bubble will intersect the buffer zone."] -> w1015
                      tunnel: [w1020 w1028] -> w1012
                      frame False {
                        n120 = local write "Looper"(FALSE) -> ()
                        n121 = local read "Current Spot #"() -> (w1021:dbl)
                        n122 = Index Array(array=w1020, index=w1021) -> (element=w1019:T3)
                        n123 = Unbundle By Name(w1019) -> ("Position.x"=w1018:dbl, "Position.y"=w1017:dbl)
                        n124 = local write "New Y"(w1017) -> ()
                        n125 = local write "New X"(w1018) -> ()
                      }
                      frame True {
                        # "Restore original position"
                        n126 = local write "Looper"(FALSE) -> ()
                        n127 = local read "Old Y"() -> (w1025:dbl)
                        n128 = local read "Old X"() -> (w1026:dbl)
                        n129 = local read "Position"() -> (w1024:cluster{"x":dbl, "y":dbl, "z":dbl})
                        n130 = Bundle By Name(cluster=w1024, "x"=w1026, "y"=w1025) -> (w1027:cluster{"x":dbl, "y":dbl, "z":dbl})
                        n131 = local write "Position"(w1027) -> ()
                      }
                    }
                  }
                }
                "Position Indicator" <- w943
              }
              event "Size": Value Change {
                # "If we were constraining the aspect ratio, or preventing a divide by zero, the size control on the FP may be incorrect.  We refresh it in here to stop it displaying a wrong value."
                # "If the size has changed, scale the spots"
                n132 = event-data() -> ("OldVal"=w1037:cluster{"x":dbl, "y":dbl, "z":dbl}, "NewVal"=w1043:cluster{"x":dbl, "y":dbl, "z":dbl})  [unwired: 5 out]
                n133 = Not Equal?(x=w1037, y=w1043) -> (x != y?=w1036:cluster{"x":bool, "y":bool, "z":bool})
                n134 = Divide(x=w1043, y=w1037) -> (x/y=w1042:cluster{"x":dbl, "y":dbl, "z":dbl})
                n135 = Not Equal To 0?(x=w1037) -> (x != 0?=w1035:cluster{"x":bool, "y":bool, "z":bool})
                n136 = And(x=w1036, y=w1035) -> (x .and. y?=w1034:cluster{"x":bool, "y":bool, "z":bool})
                n137 = Cluster To Array(cluster=w1034) -> (array=w1041:bool[])
                n138 = Cluster To Array(cluster=w1042) -> (array=w1040:dbl[])
                n139 = case shown="True" "lock aspect ratio" {
                  tunnel: w1041 -> [w1049 w1066]
                  tunnel: w1040 -> [w1048 w1064]
                  tunnel: [w1046 w1056] -> w1039
                  frame False {
                    # "We are not constraining the aspect ratio here, so just check we're not introducing NAs"
                    n140 = for {
                      tunnel: w1049 -> [w1055] mode=indexing
                      tunnel: w1048 -> [w1051] mode=indexing
                      tunnel: [w1053] -> w1047 mode=indexing
                      n141 = Not A Number/Path/Refnum?(number/path/refnum=w1051) -> (NaN/Path/Refnum?=w1052:bool)
                      n142 = Compound Arithmetic op=AND(w1055, invert w1052) -> (w1054:bool)
                      n143 = Select(t=w1051, s=w1054, f=1.0) -> (s? t:f=w1053:dbl)
                    }
                    n144 = Array To Cluster(array=w1047) -> (cluster=w1046:cluster{"[0]":dbl, "[1]":dbl, "[2]":dbl})
                  }
                  frame True {
                    # "Pick the first element that changed and use it.  Also need to make sure (1) an element did change and (2) everything's valid (no divide by zeros)"
                    n145 = Search 1D Array(1D array=w1066, element=TRUE) -> (index of element=w1063:i32)  [unwired: 1 in]
                    n146 = Index Array(array=w1064, index=w1063) -> (element=w1059:dbl)
                    n147 = Not A Number/Path/Refnum?(number/path/refnum=w1059) -> (NaN/Path/Refnum?=w1062:bool)
                    n148 = Less Than 0?(x=w1063) -> (x < 0?=w1061:bool)
                    n149 = Or(x=w1062, y=w1061) -> (x .or. y?=w1060:bool)
                    n150 = Select(t=1.0, s=w1060, f=w1059) -> (s? t:f=w1057:dbl)
                    n151 = Bundle("x"=w1057, "x"=w1057, "x"=w1057) -> (w1056:cluster{"x":dbl, "x":dbl, "x":dbl})  [unwired: 1 in]
                  }
                }
                n152 = for {
                  tunnel: w1045 -> [w1072] mode=indexing
                  tunnel: w1032 -> [w1069] mode=indexing
                  tunnel: [w1071] -> w1033 mode=indexing
                  tunnel: w1039 -> [w1070]
                  tunnel: w1044 -> [w1067]
                  n153 = Unbundle(w1069) -> ("Selected"=w1068:bool)  [unwired: 1 out]
                  n154 = case shown="True" w1068 {
                    tunnel: w1072 -> [w1073 w1081]
                    tunnel: [w1073 w1080] -> w1071
                    tunnel: w1070 -> [_ w1079]
                    tunnel: w1067 -> [_ w1075]
                    frame False {
                    }
                    frame True {
                      n155 = call "extract_position.vi"("Spot"=w1081) -> ("Position"=w1077:cluster{"x":dbl, "y":dbl, "z":dbl})
                      n156 = Subtract(x=w1077, y=w1075) -> (x-y=w1078:cluster{"x":dbl, "y":dbl, "z":dbl})
                      n157 = Multiply(x=w1078, y=w1079) -> (x*y=w1076:cluster{"x":dbl, dbl, dbl})
                      n158 = Add(x=w1075, y=w1076) -> (x+y=w1074:cluster{"x":dbl, dbl, dbl})
                      n159 = call "replace_position.vi"("Position"=w1074, "Spot in"=w1081) -> ("Spot"=w1080:T3)  [unwired: 2 out]
                    }
                  }
                }
                n160 = call "find_centroid.vi"("Selection and Groups"=w1032, "Spots"=w1033) -> ("size"=w1031:cluster{"x":dbl, "y":dbl, "z":dbl})  [unwired: 2 in, 4 out]
                n161 = local write "Size"(w1031) -> ()
              }
              event "Intensity": Value Change {
                # "When  the user changes intensity, scale all the spots selected so the new mean is correct but keep the ratio between the selected spots.\n\nThe exception to this is when the mean intensity is zero, in which case multiplying makes no sense- in that case we just replace with the new value."
                n162 = event-data() -> ("NewVal"=w1082:dbl, "OldVal"=w1089:dbl)  [unwired: 5 out]
                n163 = Equal To 0?(x=w1089) -> (x = 0?=w1085:bool)
                n164 = Not A Number/Path/Refnum?(number/path/refnum=w1089) -> (NaN/Path/Refnum?=w1084:bool)
                n165 = Or(x=w1085, y=w1084) -> (x .or. y?=w1083:bool)
                n166 = Divide(x=w1082, y=w1089) -> (x/y=w1086:dbl)
                n167 = for {
                  tunnel: w1090 -> [w1095] mode=indexing
                  tunnel: w1087 -> [w1097] mode=indexing
                  tunnel: [w1094] -> w1088 mode=indexing
                  tunnel: w1086 -> [w1093]
                  tunnel: w1083 -> [w1092]
                  tunnel: w1082 -> [w1091]
                  n168 = Unbundle(w1097) -> ("Selected"=w1096:bool)  [unwired: 1 out]
                  n169 = case shown="True" w1096 {
                    tunnel: w1095 -> [w1098 w1105]
                    tunnel: [w1098 w1102] -> w1094
                    tunnel: w1093 -> [_ w1101]
                    tunnel: w1092 -> [_ w1100]
                    tunnel: w1091 -> [_ w1099]
                    frame False {
                    }
                    frame True {
                      n170 = Unbundle By Name(w1105) -> ("Intensity"=w1103:dbl)
                      n171 = case shown="True" w1100 {
                        tunnel: [w1108 w1109] -> w1104
                        tunnel: w1103 -> [w1107 _]
                        tunnel: w1101 -> [w1106 _]
                        tunnel: w1099 -> [_ w1109]
                        frame False {
                          n172 = Multiply(x=w1107, y=w1106) -> (x*y=w1108:dbl)
                        }
                        frame True {
                        }
                      }
                      n173 = Bundle By Name(cluster=w1105, "Intensity"=w1104) -> (w1102:T3)
                    }
                  }
                }
              }
              event "phase": Value Change {
                # "When  the user changes phase, translate the phase of all spots selectedd"
                n174 = event-data() -> ("NewVal"=w1111:dbl, "OldVal"=w1115:dbl)  [unwired: 5 out]
                n175 = Not A Number/Path/Refnum?(number/path/refnum=w1115) -> (NaN/Path/Refnum?=w1110:bool)
                n176 = Subtract(x=w1111, y=w1115) -> (x-y=w1112:dbl)
                n177 = for {
                  tunnel: w1116 -> [w1121] mode=indexing
                  tunnel: w1113 -> [w1123] mode=indexing
                  tunnel: [w1120] -> w1114 mode=indexing
                  tunnel: w1112 -> [w1119]
                  tunnel: w1110 -> [w1118]
                  tunnel: w1111 -> [w1117]
                  n178 = Unbundle(w1123) -> ("Selected"=w1122:bool)  [unwired: 1 out]
                  n179 = case shown="False" w1122 {
                    tunnel: w1121 -> [w1124 w1131]
                    tunnel: [w1124 w1128] -> w1120
                    tunnel: w1119 -> [_ w1127]
                    tunnel: w1118 -> [_ w1126]
                    tunnel: w1117 -> [_ w1125]
                    frame False {
                    }
                    frame True {
                      n180 = Unbundle By Name(w1131) -> ("Phase"=w1129:dbl)
                      n181 = case shown="False" w1126 {
                        tunnel: [w1134 w1135] -> w1130
                        tunnel: w1129 -> [w1133 _]
                        tunnel: w1127 -> [w1132 _]
                        tunnel: w1125 -> [_ w1135]
                        frame False {
                          n182 = Add(x=w1133, y=w1132) -> (x+y=w1134:dbl)
                        }
                        frame True {
                        }
                      }
                      n183 = Bundle By Name(cluster=w1131, "Phase"=w1130) -> (w1128:T3)
                    }
                  }
                }
              }
              event "Vortex Charge": Value Change {
                # "When  the user changes l, just set all selected spots to have that value of l."
                n184 = event-data() -> ("NewVal"=w1136:i8)  [unwired: 6 out]
                n185 = for {
                  tunnel: w1139 -> [w1142] mode=indexing
                  tunnel: w1137 -> [w1144] mode=indexing
                  tunnel: [w1141] -> w1138 mode=indexing
                  tunnel: w1136 -> [w1140]
                  n186 = Unbundle(w1144) -> ("Selected"=w1143:bool)  [unwired: 1 out]
                  n187 = case shown="True" w1143 {
                    tunnel: w1142 -> [w1145 w1148]
                    tunnel: [w1145 w1147] -> w1141
                    tunnel: w1140 -> [_ w1146]
                    frame False {
                    }
                    frame True {
                      n188 = Bundle By Name(cluster=w1148, "Vortex Charge"=w1146) -> (w1147:T3)
                    }
                  }
                }
              }
            }
          }
          frame "Spot Shape" {
            # "We update the spot shape tab only when spots have changed OUTSIDE this tab.  This avoids unnecessary jumping about of the tab control."
            n189 = call "find_centroid.vi"("Selection and Groups"=w1159, "Spots"=w1160) -> ("Mean Values"=w1155:T3)  [unwired: 2 in, 4 out]
            n190 = Wait (ms)(milliseconds to wait=u32 10) -> ()  [unwired: 1 out]
            n191 = call "spots_shape.vi"("Selection and Groups"=w1159, "Spots"=w1160) -> ("Spot Shape"=w1162:enum32{"Normal", "Line", "NA", "Mixed"})  [unwired: 7 in]
            n192 = feedback-in #4(w1155) -> ()
            n193 = feedback #4() -> (w1156:T3)  [unwired: 1 in]
            n194 = Not Equal?(x=w1156, y=w1155) -> (x != y?=w1161:bool)
            n195 = feedback #5() -> (w1151:enum32{"Normal", "Line", "NA", "Mixed"})  [unwired: 1 in]
            n196 = feedback #6() -> (w1153:T3)  [unwired: 1 in]
            n197 = Not Equal?(x=w1153, y=w1155) -> (x != y?=w1152:bool)
            n198 = case shown="False" w1152 {
              tunnel: w1162 -> [_ w1281]
              tunnel: ["Spot Shape" w1281] -> w1150
              frame False {
              }
              frame True {
                n199 = local write "Spot Shape"(w1281) -> ()
              }
            }
            n200 = feedback-in #5(w1150) -> ()
            n201 = Not Equal?(x=w1150, y=w1151) -> (x != y?=w1149:bool)
            n202 = case shown="\"Normal\", Default" w1150 {
              tunnel: w1160 -> [w1166 w1183 w1209 w1279]
              tunnel: w1159 -> [w1165 w1182 w1208 w1278]
              tunnel: [w1165 w1181 w1206 w1278] -> w1157
              tunnel: [w1164 w1180 w1207 w1279] -> w1158
              tunnel: w1155 -> [_ w1179 w1205 _]
              tunnel: w1161 -> [_ w1178 w1204 _]
              tunnel: w1149 -> [_ w1176 w1202 _]
              frame "Normal", Default {
                # "If \"normal\" is selected, don't allow any NA or line-trapping stuff"
                n203 = for {
                  tunnel: w1166 -> [w1169] mode=indexing
                  tunnel: w1165 -> [w1168] mode=indexing
                  tunnel: [w1170] -> w1164 mode=indexing
                  n204 = Unbundle(w1168) -> ("Selected"=w1167:bool)  [unwired: 1 out]
                  n205 = case shown="True" w1167 {
                    tunnel: [w1171 w1175] -> w1170
                    tunnel: w1169 -> [w1171 w1174]
                    frame False {
                    }
                    frame True {
                      n206 = Bundle By Name(cluster=w1174, "NA Position"=cluster{"x":dbl, "y":dbl, "r":dbl} {"x"=0.0, "y"=0.0, "r"=1.0} ("x"), "Line Trapping"=T4 {"Vector"={"x"=0.0, "y"=0.0, "z"=0.0}, "Phase Gradient"=0.0}) -> (w1175:T3)
                    }
                  }
                }
              }
              frame "Line" {
                # "If it's out of date, update front panel"
                n207 = Or(x=w1178, y=w1176) -> (x .or. y?=w1177:bool)
                n208 = case shown="True" w1177 {
                  tunnel: w1179 -> [_ w1186]
                  frame False {
                  }
                  frame True {
                    n209 = Unbundle By Name(w1186) -> ("Line Trapping"=w1185:T4)
                    n210 = local write "Line Trapping"(w1185) -> ()
                  }
                }
                n211 = event shown="[1] \"Line Trapping\": Value Change" {
                  selector: _ -> [_ _]
                  dyn-events: _ -> [_ _]
                  timeout: 10 -> [_ _]
                  tunnel: w1183 -> [w1188 w1192]
                  tunnel: w1182 -> [w1187 w1190]
                  tunnel: [w1188 w1191] -> w1180
                  tunnel: [w1187 w1190] -> w1181
                  event Timeout {
                    n212 = event-data() -> ()  [unwired: 3 out]
                  }
                  event Value Change {
                    # "If the line vector has changed, update it"
                    n213 = event-data() -> ("NewVal"=w1189:T4)  [unwired: 6 out]
                    n214 = for {
                      tunnel: w1192 -> [w1197] mode=indexing
                      tunnel: w1190 -> [w1194] mode=indexing
                      tunnel: [w1196] -> w1191 mode=indexing
                      tunnel: w1189 -> [w1195]
                      n215 = Unbundle(w1194) -> ("Selected"=w1193:bool)  [unwired: 1 out]
                      n216 = case shown="True" w1193 {
                        tunnel: w1197 -> [w1198 w1200]
                        tunnel: [w1198 w1201] -> w1196
                        tunnel: w1195 -> [_ w1199]
                        frame False {
                        }
                        frame True {
                          n217 = Bundle By Name(cluster=w1200, "Line Trapping"=w1199) -> (w1201:T3)
                        }
                      }
                    }
                  }
                }
              }
              frame "NA" {
                n218 = Or(x=w1202, y=w1204) -> (x .or. y?=w1203:bool)
                n219 = case shown="True" w1203 {
                  tunnel: w1205 -> [_ w1214]
                  frame False {
                  }
                  frame True {
                    n220 = Unbundle By Name(w1214) -> ("NA Position"=w1213:cluster{"x":dbl, "y":dbl, "r":dbl})
                    n221 = call "xyz_to_xy.vi"("Position"=w1213) -> ("Position (2D)"=w1212:cluster{"x":dbl, "y":dbl}, "z"=w1211:dbl)  [unwired: 6 out]
                    n222 = local write "Position on back aperture"(w1212) -> ()
                    n223 = local write "Radius on back aperture"(w1211) -> ()
                  }
                }
                n224 = event shown="[3] \"Scale BA\": Value Change" {
                  selector: _ -> [_ _ _ _]
                  dyn-events: _ -> [_ _ _ _]
                  timeout: 10 -> [_ _ _ _]
                  tunnel: w1209 -> [w1216 w1222 w1243 w1265]
                  tunnel: w1208 -> [w1215 w1220 w1240 w1266]
                  tunnel: [w1216 w1221 w1241 w1263] -> w1207
                  tunnel: [w1215 w1220 w1240 w1266] -> w1206
                  event Timeout {
                    n225 = event-data() -> ()  [unwired: 3 out]
                  }
                  event "Position on back aperture": Value Change {
                    # "If the position has changed, translate the spots"
                    n226 = event-data() -> ("OldVal"=w1218:cluster{"x":dbl, "y":dbl}, "NewVal"=w1219:cluster{"x":dbl, "y":dbl})  [unwired: 5 out]
                    n227 = Subtract(x=w1219, y=w1218) -> (x-y=w1217:cluster{"x":dbl, "y":dbl})
                    n228 = for {
                      tunnel: w1222 -> [w1227] mode=indexing
                      tunnel: w1220 -> [w1224] mode=indexing
                      tunnel: [w1226] -> w1221 mode=indexing
                      tunnel: w1217 -> [w1225]
                      n229 = Unbundle(w1224) -> ("Selected"=w1223:bool)  [unwired: 1 out]
                      n230 = case shown="True" w1223 {
                        tunnel: w1227 -> [w1228 w1230]
                        tunnel: [w1228 w1231] -> w1226
                        tunnel: w1225 -> [_ w1232]
                        frame False {
                        }
                        frame True {
                          n231 = Unbundle By Name(w1230) -> ("NA Position"=w1234:cluster{"x":dbl, "y":dbl, "r":dbl})
                          n232 = call "xy_to_xyz.vi"("Position (2D)"=w1232) -> ("Position (3D)"=w1233:cluster{dbl, dbl, dbl})  [unwired: 1 in, 2 out]
                          n233 = Add(x=w1234, y=w1233) -> (x+y=w1229:cluster{dbl, dbl, dbl})
                          n234 = Bundle By Name(cluster=w1230, "NA Position"=w1229) -> (w1231:T3)
                        }
                      }
                    }
                  }
                  event "Radius on back aperture": Value Change {
                    # "When  the user changes intensity, scale all the spots selected so the new mean is correct but keep the ratio between the selected spots.\n\nThe exception to this is when the mean intensity is zero, in which case multiplying makes no sense- in that case we just replace with the new value."
                    n235 = event-data() -> ("NewVal"=w1235:dbl, "OldVal"=w1242:dbl)  [unwired: 5 out]
                    n236 = Equal To 0?(x=w1242) -> (x = 0?=w1238:bool)
                    n237 = Not A Number/Path/Refnum?(number/path/refnum=w1242) -> (NaN/Path/Refnum?=w1237:bool)
                    n238 = Or(x=w1238, y=w1237) -> (x .or. y?=w1236:bool)
                    n239 = Divide(x=w1235, y=w1242) -> (x/y=w1239:dbl)
                    n240 = for {
                      tunnel: w1243 -> [w1248] mode=indexing
                      tunnel: w1240 -> [w1250] mode=indexing
                      tunnel: [w1247] -> w1241 mode=indexing
                      tunnel: w1239 -> [w1246]
                      tunnel: w1236 -> [w1245]
                      tunnel: w1235 -> [w1244]
                      n241 = Unbundle(w1250) -> ("Selected"=w1249:bool)  [unwired: 1 out]
                      n242 = case shown="True" w1249 {
                        tunnel: w1248 -> [w1251 w1258]
                        tunnel: [w1251 w1255] -> w1247
                        tunnel: w1246 -> [_ w1254]
                        tunnel: w1245 -> [_ w1253]
                        tunnel: w1244 -> [_ w1252]
                        frame False {
                        }
                        frame True {
                          n243 = Unbundle By Name(w1258) -> ("NA Position.r"=w1256:dbl)
                          n244 = case shown="False" w1253 {
                            tunnel: [w1261 w1262] -> w1257
                            tunnel: w1256 -> [w1260 _]
                            tunnel: w1254 -> [w1259 _]
                            tunnel: w1252 -> [_ w1262]
                            frame False {
                              n245 = Multiply(x=w1260, y=w1259) -> (x*y=w1261:dbl)
                            }
                            frame True {
                            }
                          }
                          n246 = Bundle By Name(cluster=w1258, "NA Position.r"=w1257) -> (w1255:T3)
                        }
                      }
                    }
                  }
                  event "Scale BA": Value Change {
                    n247 = event-data() -> ()  [unwired: 7 out]
                    n248 = for {
                      tunnel: w1266 -> [w1271] mode=indexing
                      tunnel: w1265 -> [w1269] mode=indexing
                      tunnel: "Scale back aperture" -> [w1268]
                      tunnel: [w1267] -> w1263 mode=indexing
                      n249 = Unbundle(w1271) -> ("Selected"=w1270:bool)  [unwired: 1 out]
                      n250 = case shown="True" w1270 {
                        tunnel: w1269 -> [w1272 w1273]
                        tunnel: w1268 -> [_ w1276]
                        tunnel: [w1272 w1274] -> w1267
                        frame False {
                        }
                        frame True {
                          n251 = Unbundle By Name(w1273) -> ("NA Position"=w1277:cluster{"x":dbl, "y":dbl, "r":dbl})
                          n252 = Multiply(x=w1276, y=w1277) -> (x*y=w1275:cluster{"x":dbl, "y":dbl, "r":dbl})
                          n253 = Bundle By Name(cluster=w1273, "NA Position"=w1275) -> (w1274:T3)
                        }
                      }
                    }
                  }
                }
              }
              frame "Mixed" {
              }
            }
            n254 = call "find_centroid.vi"("Selection and Groups"=w1157, "Spots"=w1158) -> ("Mean Values"=w1154:T3)  [unwired: 2 in, 4 out]
            n255 = feedback-in #6(w1154) -> ()
          }
          frame "Rotate" {
            w1292 = u32 0 items=["Frame", "Fill", "Highlight"] ("Drawing Mode")
            w1291 = u32 0 ("Color")
            w1288 = i16 100 ("radius")
            # "It's necessary to check this has changed to stop us unintentionally \"spinning\" the spots..."
            # "Draw the centroid as a spot, then a large circle+cross"
            # "It's important that this loop doesn't go too fast- it hogs the CPU.  However, each tab can have a different loop speed."
            n256 = Unbundle By Name(w1285) -> ("Position (Image Pixels)"=w1301:cluster{"X":dbl, "Y":dbl}, "Previous Position (Image Pixels)"=w1300:cluster{"X":dbl, "Y":dbl}, "Dragging"=w1302:bool)
            n257 = feedback-in #7(w1285) -> ()
            n258 = feedback #7() -> (w1286:T13)  [unwired: 1 in]
            n259 = call "find_centroid.vi"("Selection and Groups"=w1303, "Spots"=w1306) -> ("centroid"=w1299:cluster{"x":dbl, "y":dbl, "z":dbl})  [unwired: 2 in, 4 out]
            n260 = Not Equal?(x=w1285, y=w1286) -> (x != y?=w1283:bool)
            n261 = Wait (ms)(milliseconds to wait=u32 10) -> ()  [unwired: 1 out]
            n262 = And(x=w1283, y=w1302) -> (x .and. y?=w1284:bool)
            n263 = call "coords_real_to_image_currentview.vi"("Position (real coords)"=w1299) -> ("Position (pixels, relative to the top left of the image)"=w1282:cluster{dbl, dbl})  [unwired: 7 in, 1 out]
            n264 = case shown="True" w1284 {
              tunnel: w1306 -> [w1315 w1359]
              tunnel: [w1317 w1358] -> w1305
              tunnel: w1303 -> [w1316 w1360]
              tunnel: [w1316 w1360] -> w1304
              tunnel: w1299 -> [w1314 w1351]
              tunnel: w1301 -> [_ w1350]
              tunnel: w1300 -> [_ w1349]
              tunnel: w1282 -> [_ w1348]
              frame False {
                n265 = event shown="[1] Timeout" {
                  selector: _ -> [_ _]
                  dyn-events: _ -> [_ _]
                  timeout: 10 -> [_ _]
                  tunnel: [w1330 w1347] -> w1317
                  tunnel: w1316 -> [w1329 _]
                  tunnel: w1315 -> [w1328 w1347]
                  tunnel: w1314 -> [w1324 _]
                  event "rotate": Value Change {
                    n266 = event-data() -> ()  [unwired: 6 out]
                    n267 = case shown="3" "Rotation Axis" {
                      tunnel: [cluster{dbl, dbl, dbl} {0.0, 0.0, 1.0} ("Custom Axis") cluster{dbl, dbl, dbl} {1.0, 0.0, 0.0} ("Custom Axis") cluster{dbl, dbl, dbl} {0.0, 1.0, 0.0} ("Custom Axis") "Custom Axis"] -> w1325
                      frame 0, Default {
                        # "Z"
                      }
                      frame 1 {
                        # "X"
                      }
                      frame 2 {
                        # "Y"
                      }
                      frame 3 {
                      }
                    }
                    n268 = call "normalise_3d_vector.vi"("Vector"=w1325) -> ("Unit Vector"=w1327:cluster{dbl, dbl, dbl})  [unwired: 3 out]
                    n269 = Divide(x=6.283185307179586, y=360.0) -> (x/y=w1322:dbl)
                    n270 = Multiply(x="Angle (degrees)", y=w1322) -> (x*y=w1319:dbl)
                    n271 = call "arb_rotation_matrix.vi"("Unit Vector"=w1327, "theta"=w1319) -> ("Real Matrix"=w1331:T7)
                    n272 = for {
                      tunnel: w1329 -> [w1341] mode=indexing
                      tunnel: w1328 -> [w1336] mode=indexing
                      tunnel: [w1337] -> w1330 mode=indexing
                      tunnel: w1324 -> [w1339]
                      tunnel: w1331 -> [w1338]
                      n273 = Unbundle(w1341) -> ("Selected"=w1340:bool)  [unwired: 1 out]
                      n274 = case shown="True" w1340 {
                        tunnel: w1339 -> [_ w1346]
                        tunnel: [w1342 w1345] -> w1337
                        tunnel: w1336 -> [w1342 w1344]
                        tunnel: w1338 -> [_ w1343]
                        frame False {
                        }
                        frame True {
                          n275 = call "apply_matrix_transformation_to_spots.vi"("Transform centre (i.e. transform about this point)"=w1346, "Transformation Matrix (3x3)"=w1343, "Spot In"=w1344) -> ("Spot Out"=w1345:T3)  [unwired: 5 out]
                        }
                      }
                    }
                  }
                  event Timeout {
                    n276 = event-data() -> ()  [unwired: 4 out]
                  }
                }
              }
              frame True {
                # "if the mouse has not moved, stuff will be NaN, so let's make like a leopard and not change our spots"
                # "the magnitude of the change in our direction vector gives the rotation angle in radians"
                # "If it's within 100px of the centroid, pretend the mouse is on the surface of a sphere, and synthesize Z accordingly (z^2=100^2-x^2-y^2).  This allows rotation in 3d :)  The output should always be a unit vector."
                n277 = Build Array(w1350, w1349) -> (w1365:cluster{"X":dbl, "Y":dbl}[])
                n278 = for {
                  tunnel: w1348 -> [w1398]
                  tunnel: w1365 -> [w1394] mode=indexing
                  tunnel: [w1384] -> w1364 mode=indexing
                  n279 = Subtract(x=w1394, y=w1398) -> (x-y=w1389:cluster{dbl, dbl})
                  n280 = Divide(x=w1389, y=100.0 ("x")) -> (x/y=w1390:cluster{dbl, dbl})
                  n281 = Square(x=w1390) -> (x^2=w1397:cluster{dbl, dbl})
                  n282 = Unbundle(w1397) -> (w1395:dbl, w1396:dbl)
                  n283 = Add(x=w1395, y=w1396) -> (x+y=w1386:dbl)
                  n284 = Subtract(x=1.0, y=w1386) -> (x-y=w1392:dbl)
                  n285 = Square Root(x=w1386) -> (sqrt(x)=w1387:dbl)
                  n286 = Greater Than 0?(x=w1392) -> (x > 0?=w1393:bool)
                  n287 = case shown="False" w1393 {
                    tunnel: w1392 -> [_ w1405]
                    tunnel: [0.0 w1404] -> w1383
                    tunnel: w1390 -> [w1402 w1403]
                    tunnel: w1387 -> [w1401 _]
                    tunnel: [w1400 w1403] -> w1385
                    frame False {
                      n288 = Divide(x=w1402, y=w1401) -> (x/y=w1400:cluster{dbl, dbl})
                    }
                    frame True {
                      n289 = Square Root(x=w1405) -> (sqrt(x)=w1404:dbl)
                    }
                  }
                  n290 = call "xy_to_xyz.vi"("z"=w1383, "Position (2D)"=w1385) -> ("Position (3D)"=w1384:cluster{dbl, dbl, dbl})  [unwired: 2 out]
                }
                n291 = Index Array(array=w1364) -> (element #1=w1363:cluster{dbl, dbl, dbl}, element #2=w1354:cluster{dbl, dbl, dbl})  [unwired: 2 in]
                n292 = Add(x=w1363, y=w1354) -> (x+y=w1353:cluster{dbl, dbl, dbl})
                n293 = Subtract(x=w1363, y=w1354) -> (x-y=w1352:cluster{dbl, dbl, dbl})
                n294 = call "cross_product.vi"("b"=w1353, "a"=w1352) -> ("a cross b"=w1362:cluster{dbl, dbl, dbl})
                n295 = call "normalise_3d_vector.vi"("Vector"=w1362) -> ("Unit Vector"=w1361:cluster{dbl, dbl, dbl})  [unwired: 3 out]
                n296 = call "normalise_3d_vector.vi"("Vector"=w1352) -> ("magnitude"=w1356:dbl)  [unwired: 3 out]
                n297 = Not Equal To 0?(x=w1356) -> (x != 0?=w1355:bool)
                n298 = call "arb_rotation_matrix.vi"("Unit Vector"=w1361, "theta"=w1356) -> ("Real Matrix"=w1357:T7)
                n299 = case shown="True" w1355 {
                  tunnel: w1360 -> [_ w1371]
                  tunnel: w1359 -> [w1366 w1370]
                  tunnel: [w1366 w1369] -> w1358
                  tunnel: w1357 -> [_ w1368]
                  tunnel: w1351 -> [_ w1367]
                  frame False {
                  }
                  frame True {
                    n300 = for {
                      tunnel: w1371 -> [w1377] mode=indexing
                      tunnel: w1370 -> [w1374] mode=indexing
                      tunnel: [w1373] -> w1369 mode=indexing
                      tunnel: w1368 -> [w1375]
                      tunnel: w1367 -> [w1372]
                      n301 = Unbundle(w1377) -> ("Selected"=w1376:bool)  [unwired: 1 out]
                      n302 = case shown="True" w1376 {
                        tunnel: [w1378 w1381] -> w1373
                        tunnel: w1374 -> [w1378 w1382]
                        tunnel: w1375 -> [_ w1379]
                        tunnel: w1372 -> [_ w1380]
                        frame False {
                        }
                        frame True {
                          n303 = call "apply_matrix_transformation_to_spots.vi"("Transform centre (i.e. transform about this point)"=w1380, "Transformation Matrix (3x3)"=w1379, "Spot In"=w1382) -> ("Spot Out"=w1381:T3)  [unwired: 5 out]
                        }
                      }
                    }
                  }
                }
              }
            }
            n304 = call "coords_real_to_image_currentview.vi"("Position (real coords)"=w1299) -> ("Position (pixels, relative to the top left of the image)"=w1294:cluster{dbl, dbl}, "z (real coords)"=w1298:dbl)  [unwired: 7 in]
            n305 = expression code="z*1e7+20"(w1298) -> (w1310:dbl)
            n306 = In Range and Coerce(upper limit=100.0, x=w1310, lower limit=2.0) -> (coerced(x)=w1297:dbl)  [unwired: 1 out]
            n307 = Bundle("upper limit"=w1297, "upper limit"=w1297) -> (w1290:cluster{"upper limit":dbl, "upper limit":dbl})  [unwired: 1 in]
            n308 = call "myoverlay_oval.vi"("Color"=w1291, "Drawing Mode"=w1292, "Size"=w1290, "Centre Position (pixels on image)"=w1294) -> ("Overlay Elements Out"=w1296:T21[])  [unwired: 5 in]
            n309 = Bundle("radius"=w1288, "radius"=w1288) -> (w1289:cluster{"radius":i16, "radius":i16})  [unwired: 1 in]
            n310 = call "myoverlay_oval.vi"("Color"=w1291, "Drawing Mode"=w1292, "Size"=w1289, "Centre Position (pixels on image)"=w1294, "Overlay Elements In"=w1296) -> ("Overlay Elements Out"=w1295:T21[])  [unwired: 4 in]
            n311 = Multiply(x=w1288, y=cluster{dbl, dbl}[] [{0.0, 0.0}, {1.0, 0.0}, {0.0, 0.0}, {0.0, 1.0}, {0.0, 0.0}, {-1.0, 0.0}, {0.0, 0.0}, {0.0, -1.0}, {0.0, 0.0}]) -> (x*y=w1307:cluster{dbl, dbl}[])
            n312 = Add(x=w1294, y=w1307) -> (x+y=w1293:cluster{dbl, dbl}[])
            n313 = call "myoverlay_lines.vi"("Color"=w1291, "Drawing Mode"=w1292, "Line Endpoints"=w1293, "Overlay Elements In"=w1295) -> ("Overlay Elements Out"=w1287:T21[])  [unwired: 5 in]
          }
          frame "Patterns" {
            n314 = event shown="[3] \"Optimise\": Value Change" {
              selector: _ -> [_ _ _ _ _]
              dyn-events: _ -> [_ _ _ _ _]
              timeout: u32 10 ("milliseconds to wait") -> [_ _ _ _ _]
              tunnel: [w1424 w1454 w1458 w1461 w1472] -> w1407
              tunnel: [w1423 w1455 w1457 w1464 w1473] -> w1406
              tunnel: w1409 -> [w1422 w1454 w1458 w1462 w1471]
              tunnel: w1408 -> [w1421 w1455 w1457 w1464 w1473]
              event "Generate": Value Change {
                # "If there were previous spots, centre the pattern on the spots"
                n315 = event-data() -> ()  [unwired: 1 in, 1 out]
                n316 = call "find_centroid.vi"("Selection and Groups"=w1421, "Spots"=w1422) -> ("size"=w1417:cluster{"x":dbl, "y":dbl, "z":dbl}, "centroid"=w1413:cluster{"x":dbl, "y":dbl, "z":dbl}, "# selected"=w1419:i16)  [unwired: 2 in, 2 out]
                n317 = Greater?(x=w1419, y=i16 1) -> (0:w1414:bool)
                n318 = case shown="False" w1414 {
                  tunnel: w1417 -> [_ w1440]
                  tunnel: [cluster{"x":dbl, "y":dbl, "z":dbl} {"x"=2e-05, "y"=2e-05, "z"=2e-05} ("size") w1440] -> w1416
                  frame False {
                  }
                  frame True {
                  }
                }
                n319 = case shown="\"HCP Shack-Hartmann\"" "Pattern" {
                  tunnel: [w1442 w1445 w1451] -> w1415
                  tunnel: w1416 -> [_ w1444 _]
                  frame "Square Shack-Hartmann" {
                    n320 = call "patterns_square_shack_hartmann.vi"("N"="Spots across centre") -> ("Spots"=w1442:T3[])
                  }
                  frame "HCP Shack-Hartmann" {
                    n321 = Unbundle By Name(w1444) -> ("x"=w1443:dbl)
                    n322 = call "pattern_hcp_shack_hartmann.vi"("Width"=w1443, "Reference Array?"="Reference Array?", "Fraction of SLM"="Fraction of SLM", "N"="Spots across centre") -> ("Shack-Hartmann Spots"=w1445:T3[])  [unwired: 7 in]
                  }
                  frame "Rectangular Grid" {
                    n323 = call "patterns_rectangular_grid.vi"("spacing/m"="spacing/m", "N"="N") -> ("Spots"=w1451:T3[])
                  }
                }
                n324 = local write "Generate"(FALSE ("Generate")) -> ()
                n325 = case shown="True" w1414 {
                  tunnel: w1415 -> [w1427 w1431]
                  tunnel: w1413 -> [_ w1433]
                  tunnel: [w1427 w1429] -> w1425
                  frame False {
                  }
                  frame True {
                    n326 = call "find_centroid.vi"("Spots"=w1431) -> ("centroid"=w1432:cluster{"x":dbl, "y":dbl, "z":dbl}, "# selected"=→"# selected":i16)  [unwired: 3 in, 3 out]
                    n327 = Subtract(x=w1433, y=w1432) -> (x-y=w1430:cluster{"x":dbl, "y":dbl, "z":dbl})
                    n328 = for {
                      tunnel: w1431 -> [w1436] mode=indexing
                      tunnel: w1430 -> [w1435]
                      tunnel: [w1434] -> w1429 mode=indexing
                      n329 = call "extract_position.vi"("Spot"=w1436) -> ("Position"=w1437:cluster{"x":dbl, "y":dbl, "z":dbl})
                      n330 = Add(x=w1437, y=w1435) -> (x+y=w1438:cluster{"x":dbl, "y":dbl, "z":dbl})
                      n331 = call "replace_position.vi"("Position"=w1438, "Spot in"=w1436) -> ("Spot"=w1434:T3)  [unwired: 2 out]
                    }
                  }
                }
                "Last Pattern" <- w1425
                n332 = call "ensure_selection_matches_spots.vi"("Select All (default: no)"=TRUE ("Select All (default: true)"), "Spots"=w1425) -> ("Selection and Groups out"=w1423:T12[], "Spots (duplicate)"=w1424:T3[])  [unwired: 4 in]
              }
              event "Spots across centre", "Fraction of SLM", "Reference Array?", "N", "spacing/m", "Spots across centre": Value Change {
                n333 = event-data() -> ()  [unwired: 1 in, 1 out]
                n334 = local read "Last Pattern"() -> (w1453:T3[])
                n335 = Equal?(x=w1454, y=w1453) -> (x = y?=w1452:bool)
                n336 = case shown="True" w1452 {
                  selector: w1452 -> [_ w1456]
                  frame False {
                  }
                  frame True {
                    n337 = property on="Generate" class="Bool (strict)"("Val(Sgnl)"=w1456) -> ()  [unwired: 2 in, 2 out]
                  }
                }
              }
              event Timeout {
                n338 = event-data() -> ()  [unwired: 1 in, 1 out]
              }
              event "Optimise": Value Change {
                n339 = event-data() -> ()  [unwired: 1 in, 1 out]
                n340 = for {
                  N: "Iterations" -> [_]
                  tunnel: 203 ("Optimisation Resolution") -> [w1468]
                  shift-right: [w1469] -> w1461
                  shift-left: w1462 -> [w1470]
                  tunnel: "Fall-off/m" -> [w1465]
                  n341 = call "do_gsw_step.vi"("Optimisation Resolution"=w1468, "Sinc Zero"=w1465, "Spots In"=w1470) -> ("non-uniformity"=→"non-uniformity":dbl, "efficiency"=→"efficiency":dbl, "Spots Out"=w1469:T3[])  [unwired: 6 in]
                }
              }
              event "Reset Phase/Amplitude": Value Change {
                n342 = event-data() -> ()  [unwired: 1 in, 1 out]
                n343 = for {
                  tunnel: [w1476] -> w1472 mode=indexing
                  tunnel: w1471 -> [w1477] mode=indexing
                  n344 = Bundle By Name(cluster=w1477, "Phase"=0.0, "Amplitude Correction"=0.0) -> (w1476:T3)
                }
              }
            }
          }
          frame "Plugins" {
            # "The local variable ensures the references are  correct when they make it through to the \"close plugins\" block."
            # "This is the error from loading/unloading VIs on the front panel"
            n345 = control-ref of="Plugin Pnl"() -> (w1481:refnum<vi>)
            n346 = Wait (ms)(milliseconds to wait=u32 10) -> ()  [unwired: 1 out]
            n347 = feedback #8() -> (w1480:T5)
            n348 = feedback #9() -> (w1482:errorcluster)
            n349 = event shown="[1] \"Plugin:\": Value Change" {
              selector: _ -> [_ _ _]
              dyn-events: _ -> [_ _ _]
              timeout: 10 -> [_ _ _]
              tunnel: "Abort Plugin" -> [w1489 _ _]
              tunnel: "Plugin:" -> [w1494 _ w1510]
              tunnel: w1482 -> [w1493 w1508 w1512]
              tunnel: [w1492 w1503 w1511] -> w1483
              tunnel: [w1491 w1504 w1514] -> w1479
              tunnel: w1480 -> [w1495 w1505 w1513]
              tunnel: w1481 -> [_ w1506 _]
              event Timeout {
                n350 = event-data() -> ()  [unwired: 1 in, 2 out]
                n351 = Not(x=w1489) -> (.not. x?=w1490:bool)
                n352 = case shown="True" w1490 {
                  tunnel: w1495 -> [w1497 w1502]
                  tunnel: w1494 -> [_ w1501]
                  tunnel: w1493 -> [w1496 w1500]
                  tunnel: [w1496 w1499] -> w1492
                  tunnel: [w1497 w1498] -> w1491
                  frame False {
                  }
                  frame True {
                    n353 = call "plugins_run.vi"("Error In"=w1500, "Plugin Index"=w1501, "Plugins In"=w1502) -> ("Error Out"=w1499:errorcluster, "Plugins"=w1498:T5)  [unwired: 7 in]
                  }
                }
              }
              event "Plugin:": Value Change {
                n354 = event-data() -> ("NewVal"=w1507:u16)  [unwired: 1 in]
                n355 = call "plugins_switch.vi"("error in"=w1508, "Plugin Pnl"=w1506, "Plugin Index"=w1507, "Plugins In"=w1505) -> ("error out"=w1503:errorcluster, "Plugins Out"=w1504:T5)  [unwired: 4 in]
              }
              event "Abort Plugin": Value Change {
                n356 = event-data() -> ("NewVal"=w1509:bool)  [unwired: 1 in]
                n357 = case shown="True" w1509 {
                  tunnel: [w1516 w1521] -> w1514
                  tunnel: w1513 -> [w1516 w1520]
                  tunnel: w1512 -> [w1515 w1519]
                  tunnel: [w1515 w1518] -> w1511
                  tunnel: w1510 -> [_ w1517]
                  frame False {
                  }
                  frame True {
                    n358 = call "plugins_abort.vi"("Error In"=w1519, "Plugin Index"=w1517, "Plugins In"=w1520) -> ("Error Out"=w1518:errorcluster, "Plugins Out"=w1521:T5)  [unwired: 7 in]
                  }
                }
              }
            }
            n359 = feedback-in #8(w1479) -> ()
            n360 = feedback-in #9(w1483) -> ()
            n361 = local write "Plugins"(w1479) -> ()
          }
          frame "Video" {
            # "All the controls on this tab are in the bottom (camera) loop."
            n362 = Wait (ms)(milliseconds to wait=u32 10) -> ()  [unwired: 1 out]
            n363 = property on="Property Node" class="ImageControl"(reference=w1522) -> ("Image Information String"=→"Image Information":string)  [unwired: 1 in, 2 out]
          }
        }
      }
      event "Tab": Value Change {
        w1530 = T22 [enum."Video", enum."Particle Tracking"] items=["Current Spot", "Rotate", "Spot Shape", "Patterns", "Plugins", "Video", "Particle Tracking", "Clamping", "Blank"]
        w1535 = refnum<vi> refnum  # Image
        # "This allows us to disable custom mouse-handling for certain tabs.  It can also be done from within the \"mouse down\" event case."
        n364 = event-data() -> ("NewVal"=w1531:T6)  [unwired: 1 in, 3 out]
        n365 = Equal?(x=w1530, y=w1531) -> (x = y?=w1529:bool[])
        n366 = Or Array Elements(Boolean array=w1529) -> (logical OR=w1528:bool)
        n367 = Not(x=w1528) -> (.not. x?=w1527:bool)
        n368 = Select(t=w1534, s=w1527, f=w1535) -> (s? t:f=w1536:refnum<vi>)
        n369 = register-events(reference=w1538, w1536, w1535, w1535, w1535) -> (reference out=w1537:refnum<event-registration>)  [unwired: 1 in, 1 out]
      }
      event Menu Selection (User) {
        n370 = event-data() -> ("ItemTag"=w1546:string, "MenuRef"=w1539:refnum<k9>)  [unwired: 1 in]
        n371 = case shown="\"ToggleSavingData\"" w1546 {
          tunnel: w1550 -> [w1554 w1564 w1573 w1587 w1606 w1610 w1613 w1620 w1627 w1629 w1632 w1661 w1687 w1708 w1719 w1730 w1733 w1735 w1740 w1743]
          tunnel: w1549 -> [w1553 w1563 w1572 w1596 w1605 w1609 w1611 w1618 w1626 w1628 w1631 w1660 w1686 w1707 w1718 w1729 w1732 w1736 w1741 w1742]
          tunnel: [w1554 w1564 w1573 w1587 w1604 w1607 w1613 w1620 w1627 w1629 w1632 w1661 w1687 w1708 w1719 w1730 w1733 w1735 w1740 w1743] -> w1548
          tunnel: [w1553 w1563 w1572 w1596 w1603 w1608 w1612 w1619 w1625 w1630 w1633 w1660 w1686 w1707 w1718 w1729 w1732 w1736 w1741 w1742] -> w1547
          tunnel: [_ _ _ _ TRUE _ _ _ _ _ _ _ _ _ _ _ _ _ _ _] -> w1541
          tunnel: w1540 -> [_ _ _ _ _ _ _ _ _ _ _ w1659 w1685 w1699 _ _ _ _ _ _]
          tunnel: w1539 -> [_ _ _ _ _ _ _ _ _ _ _ w1650 w1679 w1702 w1713 w1724 _ _ _ _]
          frame "ToggleSavingData" {
            # "Data is saved from the middle loop: look there for an explanation."
            n372 = local read "Save Video"() -> (w1552:bool)
            n373 = Not(x=w1552) -> (.not. x?=w1551:bool)
            n374 = local write "Save Video"(w1551) -> ()
          }
          frame "SaveStateToFile" {
            # "Save the current settings (i.e. the values of all the controls in VIs that have [Red Tweezers Save Settings] in their documentation string) to a file."
            n375 = call "File Dialog"("prompt"="Please select a location to save the settings", "button label"="Save", "default name"="red_tweezers_settings.xml", "pattern (all files)"="*.xml" ("pattern label"), "pattern label"="XML Settings Files") -> ("selected path"=w1562:path, "cancelled"=w1555:bool)  [unwired: 7 in, 2 out]
            n376 = Not(x=w1555) -> (.not. x?=w1556:bool)
            n377 = case shown="True" w1556 {
              tunnel: w1562 -> [_ w1566]
              frame False {
              }
              frame True {
                n378 = Path To String(path=w1566) -> (string=w1565:string)
                n379 = call "settings_save_to_file.vi"("XML File Path"=w1566) -> ()  [unwired: 11 in]
                n380 = call "settings_filename_to_registry.vi"("Last Used Settings File"=w1565) -> ()  [unwired: 11 in]
              }
            }
          }
          frame "SaveStateToCurrentFile" {
            # "As SaveStateToFile, but using the current file (i.e. Save not Save As...)."
            n381 = global read "red_tweezers_globals_INTERNAL_VOLATILE.vi" "Current Settings File"() -> (w1571:path)
            n382 = call <vilib>:"Check if File or Folder Exists.vi"("path"=w1571) -> ("file or folder exists?"=w1570:bool, "dup path"=w1569:path)  [unwired: 8 in, 1 out]
            n383 = case shown="True" w1570 {
              selector: w1570 -> [_ w1584]
              tunnel: w1569 -> [_ w1585]
              tunnel: [w1576 w1585] -> w1568
              tunnel: [w1577 w1584] -> w1567
              frame False {
                n384 = call "File Dialog3"("prompt"="Please select a location to save the settings", "button label"="Save", "default name"="red_tweezers_settings.xml", "pattern (all files)"="*.xml" ("pattern label"), "pattern label"="XML Settings Files") -> ("selected path"=w1576:path, "cancelled"=w1583:bool)  [unwired: 7 in, 2 out]
                n385 = Not(x=w1583) -> (.not. x?=w1577:bool)
              }
              frame True {
              }
            }
            n386 = case shown="True" w1567 {
              tunnel: w1568 -> [_ w1575]
              frame False {
              }
              frame True {
                n387 = Path To String(path=w1575) -> (string=w1574:string)
                n388 = call "settings_save_to_file.vi"("XML File Path"=w1575) -> ()  [unwired: 11 in]
                n389 = call "settings_filename_to_registry.vi"("Last Used Settings File"=w1574) -> ()  [unwired: 11 in]
              }
            }
          }
          frame "LoadStateFromFile" {
            # "Load a file, and use it to reset the values of all the front panel controls."
            # "We need to re-run the initialisation stuff in UDP sender after changing settings\n(for example, this synchronises the settings like camera pixel size with the\nrelevant global variable)"
            n390 = call "File Dialog2"("prompt"="Please select a settings file", "button label"="Open", "default name"="red_tweezers_settings.xml", "pattern (all files)"="*.xml" ("pattern label"), "pattern label"="XML Settings Files") -> ("selected path"=w1588:path, "cancelled"=w1595:bool)  [unwired: 7 in, 2 out]
            n391 = Not(x=w1595) -> (.not. x?=w1594:bool)
            n392 = case shown="False" w1594 {
              selector: w1594 -> [w1597 w1598]
              tunnel: w1588 -> [_ w1599]
              tunnel: [w1597 w1598] -> w1586
              frame False {
              }
              frame True {
                n393 = call "settings_load_from_file.vi"("XML File Path"=w1599) -> ()  [unwired: 9 in, 2 out]
                n394 = Path To String(path=w1599) -> (string=w1600:string)
                n395 = call "settings_filename_to_registry.vi"("Last Used Settings File"=w1600) -> ()  [unwired: 11 in]
              }
            }
            n396 = call "UDP Sender generic_2.vi"("re-initialise"=w1586, "Spots"=w1587) -> ()  [unwired: 1 in, 1 out]
          }
          frame "Undo" {
            # "This should get the last undo vector and replace the spots with it :)"
            n397 = call "red_tweezers_UNDO.vi"("Selection/Group"=w1605, "Undo/Store (store, False)"=TRUE, "Spots"=w1606) -> ("Selection/Group Out (Undo only)"=w1603:T12[], "Spots Out (Undo only)"=w1604:T3[])  [unwired: 7 in]
          }
          frame "Delete" {
            n398 = call "delete_selected_spots.vi"("Selection/Group 3"=w1609, "Spots 3"=w1610) -> ("Selection/Group 2"=w1608:T12[], "Spots 2"=w1607:T3[])  [unwired: 4 in]
          }
          frame "SelectAllSpots" {
            n399 = for {
              tunnel: w1611 -> [w1616] mode=indexing
              tunnel: [w1617] -> w1612 mode=indexing
              n400 = Unbundle(w1616) -> ("Group ID"=w1615:i32)  [unwired: 1 out]
              n401 = Bundle(cluster=w1616, "Group ID"=w1615, "Selected"=TRUE ("Label.Visible")) -> (w1617:T12)
            }
          }
          frame "SelectNoSpots" {
            n402 = for {
              tunnel: w1618 -> [w1623] mode=indexing
              tunnel: [w1624] -> w1619 mode=indexing
              n403 = Unbundle(w1623) -> ("Group ID"=w1622:i32)  [unwired: 1 out]
              n404 = Bundle(cluster=w1623, "Group ID"=w1622, "Selected"=FALSE ("Label.Visible")) -> (w1624:T12)
            }
          }
          frame "SelectSpecificSpots" {
            n405 = call "select_by_id.vi"("Selection/Group"=w1626, "Spots"=w1627) -> ("Selection/Group Out"=w1625:T12[])  [unwired: 9 in]
          }
          frame "Group" {
            # "Group the currently selected spots"
            n406 = call "group_selected_spots.vi"("Selection/Group 2"=w1628) -> ("Array"=w1630:T12[])
          }
          frame "Ungroup" {
            # "Ungroup the currently selected spots"
            n407 = for {
              tunnel: [w1637] -> w1633 mode=indexing
              tunnel: w1631 -> [w1636] mode=indexing
              tunnel: 0 -> [w1635]
              n408 = Unbundle(w1636) -> ("Selected"=w1638:bool)  [unwired: 1 out]
              n409 = case shown="False" w1638 {
                tunnel: [w1639 w1642] -> w1637
                tunnel: w1636 -> [w1639 w1641]
                tunnel: w1635 -> [_ w1640]
                frame False {
                }
                frame True {
                  n410 = Unbundle(w1641) -> ("Selected"=w1643:bool)  [unwired: 1 out]
                  n411 = Bundle(cluster=w1641, "Group ID"=w1640, "Selected"=w1643) -> (w1642:T12)
                }
              }
            }
          }
          frame "ZoomIn" {
            w1644 = "ZoomToFit" ("item tag")
            # "turn off \"zoom to fit\""
            n412 = property class="ImageControl"(reference=w1659) -> (reference out=w1653:refnum<vi>, "ZoomSingle"=w1658:cluster{"X":sgl, "Y":sgl}, "Image Center Position"=w1651:cluster{"X":u32, "Y":u32})  [unwired: 1 in, 1 out]
            n413 = Unbundle(w1658) -> ("X"=w1656:sgl)  [unwired: 1 out]
            n414 = Round To Nearest(number=w1656) -> (nearest integer value=w1652:sgl)
            n415 = Greater Than 0?(x=w1652) -> (x > 0?=w1657:bool)
            n416 = case shown="True" w1657 {
              tunnel: w1656 -> [w1666 w1669]
              tunnel: [w1665 w1667] -> w1655
              frame False {
                n417 = Reciprocal(x=w1666) -> (1/x=w1663:sgl)
                n418 = Round Toward +Infinity(x=w1663) -> (ceil(x): smallest int >= x=w1664:sgl)
                n419 = Decrement(x=w1664) -> (x-1=w1662:sgl)
                n420 = Reciprocal(x=w1662) -> (1/x=w1665:sgl)
              }
              frame True {
                n421 = Round Toward -Infinity(1:w1669) -> (0:w1668:sgl)
                n422 = Increment(x=w1668) -> (x+1=w1667:sgl)
              }
            }
            n423 = Bundle(w1655, w1655) -> (w1654:cluster{sgl, sgl})  [unwired: 1 in]
            n424 = property class="ImageControl"(reference=w1653, "ZoomSingle"=w1654, "Image Center Position"=w1651) -> ()  [unwired: 1 in, 2 out]
            n425 = Get Menu Item Info(7:w1644, 11:w1650) -> (1:w1647:bool, 2:w1648:string, 3:w1649:refnum<k9>, 6:w1646:T23)  [unwired: 1 in, 3 out]
            n426 = Set Menu Item Info(4:w1646, 6:FALSE ("checked"), 7:w1644, 9:w1647, 10:w1648, 11:w1649) -> ()  [unwired: 1 in, 2 out]
          }
          frame "ZoomOut" {
            w1673 = "ZoomToFit" ("item tag")
            # "turn off \"zoom to fit\""
            n427 = property class="ImageControl"(reference=w1685) -> (reference out=w1681:refnum<vi>, "ZoomSingle"=w1684:cluster{"X":sgl, "Y":sgl}, "Image Center Position"=w1680:cluster{"X":u32, "Y":u32})  [unwired: 1 in, 1 out]
            n428 = Unbundle(w1684) -> ("X"=w1670:sgl)  [unwired: 1 out]
            n429 = Greater?(x=w1670, y=1.0) -> (0:w1672:bool)
            n430 = case shown="False" w1672 {
              tunnel: w1670 -> [w1694 w1697]
              tunnel: [w1693 w1695] -> w1683
              frame False {
                n431 = Reciprocal(x=w1694) -> (1/x=w1691:sgl)
                n432 = Add(x=w1691, y=sgl 0.01 ("x")) -> (x+y=w1689:sgl)
                n433 = Round Toward -Infinity(1:w1689) -> (0:w1692:sgl)
                n434 = Increment(x=w1692) -> (x+1=w1690:sgl)
                n435 = Reciprocal(x=w1690) -> (1/x=w1693:sgl)
              }
              frame True {
                n436 = Round Toward +Infinity(x=w1697) -> (ceil(x): smallest int >= x=w1696:sgl)
                n437 = Decrement(x=w1696) -> (x-1=w1695:sgl)
              }
            }
            n438 = Bundle(w1683, w1683) -> (w1682:cluster{sgl, sgl})  [unwired: 1 in]
            n439 = property class="ImageControl"(reference=w1681, "ZoomSingle"=w1682, "Image Center Position"=w1680) -> ()  [unwired: 1 in, 2 out]
            n440 = Get Menu Item Info(7:w1673, 11:w1679) -> (1:w1676:bool, 2:w1677:string, 3:w1678:refnum<k9>, 6:w1675:T23)  [unwired: 1 in, 3 out]
            n441 = Set Menu Item Info(4:w1675, 6:FALSE ("checked"), 7:w1673, 9:w1676, 10:w1677, 11:w1678) -> ()  [unwired: 1 in, 2 out]
          }
          frame "ZoomToFit" {
            w1703 = "ZoomToFit" ("item tag")
            # "and make sure the image obeys the result"
            # "Toggle menu checkmark"
            n442 = Get Menu Item Info(7:w1703, 11:w1702) -> (1:w1701:bool, 2:w1705:string, 3:w1706:refnum<k9>, 4:w1700:bool, 6:w1704:T23)  [unwired: 1 in, 2 out]
            n443 = Not(x=w1700) -> (.not. x?=w1698:bool)
            n444 = Set Menu Item Info(4:w1704, 6:w1698, 7:w1703, 9:w1701, 10:w1705, 11:w1706) -> ()  [unwired: 1 in, 2 out]
            n445 = property class="ImageControl"(reference=w1699, "Zoom to Fit Mode"=w1698) -> ()  [unwired: 1 in, 2 out]
          }
          frame "ShowGrid" {
            w1714 = "ShowGrid" ("item tag")
            # "Toggle menu checkmark"
            n446 = Get Menu Item Info(7:w1714, 11:w1713) -> (1:w1712:bool, 2:w1716:string, 3:w1717:refnum<k9>, 4:w1711:bool, 6:w1715:T23)  [unwired: 1 in, 2 out]
            n447 = Not(x=w1711) -> (.not. x?=w1710:bool)
            n448 = Set Menu Item Info(4:w1715, 6:w1710, 7:w1714, 9:w1712, 10:w1716, 11:w1717) -> ()  [unwired: 1 in, 2 out]
            n449 = call "grid_and_guides.vi"("Boolean"=w1710, "Operation"=T16."Set grid visibility") -> ()  [unwired: 9 in, 1 out]
          }
          frame "ShowGuides" {
            w1725 = "ShowGuides" ("item tag")
            # "Toggle menu checkmark"
            n450 = Get Menu Item Info(7:w1725, 11:w1724) -> (1:w1723:bool, 2:w1727:string, 3:w1728:refnum<k9>, 4:w1722:bool, 6:w1726:T23)  [unwired: 1 in, 2 out]
            n451 = Not(x=w1722) -> (.not. x?=w1721:bool)
            n452 = Set Menu Item Info(4:w1726, 6:w1721, 7:w1725, 9:w1723, 10:w1727, 11:w1728) -> ()  [unwired: 1 in, 2 out]
            n453 = call "grid_and_guides.vi"("Boolean"=w1721, "Operation"=T16."Set guide visibility") -> ()  [unwired: 9 in, 1 out]
          }
          frame "ConfigureGridAndGuides" {
            n454 = call "grid_and_guides.vi"("Operation"=T16."Show front panel") -> ()  [unwired: 10 in, 1 out]
          }
          frame "ShowSettings" {
            n455 = call "UDP Sender generic_2.vi"("Show panel"=TRUE, "Spots"=w1735) -> ()  [unwired: 1 in, 1 out]
          }
          frame "CameraSettings" {
            n456 = global read "red_tweezers_globals_INTERNAL_VOLATILE.vi" "Current Camera VI"() -> (w1738:path)
            n457 = Open VI Reference(vi path=w1738) -> (vi reference=w1737:refnum<vi>)  [unwired: 5 in, 1 out]
            n458 = property class="VI"(reference=w1737, "Front Panel.Open"=TRUE ("Front Panel Window:Open")) -> ()  [unwired: 1 in, 2 out]
          }
          frame Default {
          }
        }
      }
      event Mouse Down? {
        # "We don't process clicks when the user is on the video tab, so that we can set ROIs."
        # "When the mouse button goes down over the image, we save where it went down, etc. and wait to see what happens next.  We also register to be told when the mouse leaves the control, goes up, or moves.  \"click\" or \"drag\" are only detected once the mouse moves or goes up."
        n459 = event-data() -> ("Coords"=w1758:T24, "Button"=w1753:u16, "Mods"=w1762:cluster{"Double Click":bool, "Menu Key":bool}, "PlatMods"=w1761:T25)  [unwired: 1 in]
        n460 = call "mouse_to_image_coords.vi"("Mouse Coords (screen/pane units)"=w1758, "Image Control"=w1754) -> ("Cursor is on Display Area"=w1752:bool, "Mouse Coords (image pixels)"=w1757:cluster{dbl, dbl})  [unwired: 4 in]
        n461 = disable-structure shown="Enabled" {
          disable-tunnel: w1753 -> [w1770 _]
          disable-tunnel: w1752 -> [w1768 w1771]
          disable-tunnel: [w1767 w1771] -> w1748
          frame Enabled {
            n462 = Equal?(x=u16 1, y=w1770) -> (x = y?=w1769:bool)
            n463 = And(x=w1768, y=w1769) -> (x .and. y?=w1767:bool)
          }
          frame Disabled {
            # "use other pane to allow right-clicking on image"
          }
        }
        n464 = local read "Tab"() -> (w1749:T6)
        n465 = Not Equal?(x=w1749, y=T17."Video" ("Tab")) -> (x != y?=w1747:bool)
        n466 = And(x=w1748, y=w1747) -> (x .and. y?=w1746:bool)
        n467 = case shown="False" w1746 {
          tunnel: w1765 -> [w1774 w1785]
          tunnel: [T13 {"Button Down"=FALSE, "Dragging"=FALSE, "Position (Image Pixels)"={"X"=0.0, "Y"=0.0}, "Previous Position (Image Pixels)"={"X"=0.0, "Y"=0.0}, "Button"=0, "Mods"={"Double Click"=FALSE, "Menu Key"=FALSE}, "PlatMods"={"Shift"=FALSE, "Ctrl"=FALSE, "Alt"=FALSE, "Cmd"=FALSE, "Opt"=FALSE}} w1784] -> w1764
          tunnel: [w1774 w1781] -> w1763
          tunnel: w1753 -> [_ w1780]
          tunnel: w1762 -> [_ w1779]
          tunnel: w1761 -> [_ w1778]
          tunnel: w1757 -> [_ w1777]
          tunnel: [FALSE TRUE] -> w1756
          tunnel: w1754 -> [_ w1775]
          frame False {
            # "If the user clicked on a scrollbar, ignore it and let LabVIEW handle it. (this keeps the scrollbars working)"
          }
          frame True {
            w1783 = FALSE  # Dragging
            w1782 = TRUE  # Button Down
            n468 = register-events(reference=w1785, w1775, w1775, w1775, w1775) -> (reference out=w1781:refnum<event-registration>)  [unwired: 1 in, 1 out]
            n469 = Bundle("Button Down"=w1782, "Dragging"=w1783, "Mouse Coords (image pixels)"=w1777, "Mouse Coords (image pixels)"=w1777, "Button"=w1780, "Mods"=w1779, "PlatMods"=w1778) -> (w1784:T26)  [unwired: 1 in]
          }
        }
        n470 = Array Size(array=w1744) -> (size(s)=w1745:i32)
        n471 = local write "# of Spots"(w1745) -> ()
        n472 = local write "Selection/Group"(w1744) -> ()
        n473 = event-data("Discard?"=w1756) -> ()  [unwired: 4 in, 1 out]
      }
      event Mouse Leave {
        w1792 = refnum<vi> refnum  # Dummy
        # "When the mouse leaves, we reset things."
        n474 = event-data() -> ()  [unwired: 1 in, 2 out]
        n475 = register-events(reference=w1793, w1791, w1792, w1792, w1792) -> (reference out=w1790:refnum<event-registration>)  [unwired: 1 in, 1 out]
      }
      event Mouse Up {
        w1812 = refnum<vi> refnum  # Dummy
        # "Double clicking adds a spot at the mouse position."
        # "deregister"
        # "If we get here the mouse has gone down and up again.  If we've not moved in between, we have a Click.\nEither way we're no longer interested in mouse leave/move/up events."
        n476 = event-data() -> ("Mods"=w1799:cluster{"Double Click":bool, "Menu Key":bool})  [unwired: 1 in, 5 out]
        n477 = Unbundle By Name(w1805) -> ("Dragging"=w1814:bool)
        n478 = Unbundle By Name(w1799) -> ("Double Click"=w1796:bool)
        n479 = Not(x=w1814) -> (.not. x?=w1813:bool)
        n480 = Not(x=w1801) -> (.not. x?=w1803:bool)
        n481 = And(x=w1813, y=w1803) -> (x .and. y?=w1797:bool)
        n482 = case shown="True" w1797 {
          tunnel: w1805 -> [_ w1820]
          tunnel: w1807 -> [w1815 w1819]
          tunnel: w1806 -> [w1816 w1822]
          tunnel: [w1816 w1821] -> w1808
          tunnel: w1796 -> [_ w1817]
          tunnel: [w1815 w1818] -> w1798
          frame False {
          }
          frame True {
            n483 = case shown="True" w1817 {
              tunnel: w1822 -> [w1829 w1879]
              tunnel: [w1827 w1885] -> w1821
              tunnel: w1819 -> [w1823 w1886]
              tunnel: w1820 -> [w1826 w1881]
              tunnel: [w1823 w1877] -> w1818
              frame False {
                w1833 = 400.0  # 20^2 px
                # "If the user clicked, determine which spots should be selected: if we've clicked a spot/group then select it.  Shift-clicking toggles selection for that spot, and leaves the rest of the selection unchanged."
                # "check we're close enough"
                # "find closest"
                n484 = Unbundle By Name(w1826) -> ("Position (Image Pixels)"=w1825:cluster{"X":dbl, "Y":dbl}, "PlatMods.Shift"=w1824:bool)
                n485 = for {
                  tunnel: [w1869] -> w1831 mode=indexing
                  tunnel: w1825 -> [w1868]
                  tunnel: w1823 -> [w1867] mode=indexing
                  # "calculate distances between mouse position and spot positions"
                  n486 = call "extract_position.vi"("Spot"=w1867) -> ("Position"=w1866:cluster{"x":dbl, "y":dbl, "z":dbl})
                  n487 = call "coords_real_to_image_currentview.vi"("Position (real coords)"=w1866) -> ("Position (pixels, relative to the top left of the image)"=w1865:cluster{dbl, dbl})  [unwired: 7 in, 1 out]
                  n488 = Subtract(x=w1865, y=w1868) -> (x-y=w1872:cluster{dbl, dbl})
                  n489 = Multiply(x=w1872, y=w1872) -> (x*y=w1871:cluster{dbl, dbl})
                  n490 = Cluster To Array(cluster=w1871) -> (array=w1870:dbl[])
                  n491 = Add Array Elements(numeric array=w1870) -> (sum=w1869:dbl)
                }
                n492 = Array Max & Min(array=w1831) -> (min value=w1832:dbl, min index (indices)=w1828:i32)  [unwired: 2 out]
                n493 = Less Or Equal?(x=w1832, y=w1833) -> (x <= y?=w1830:bool)
                n494 = case shown="True" w1830 {
                  tunnel: w1829 -> [w1834 w1841]
                  tunnel: w1828 -> [_ w1835]
                  tunnel: w1824 -> [_ w1837]
                  tunnel: [w1834 w1836] -> w1827
                  frame False {
                    # "If we didn't click a spot, do nothing."
                  }
                  frame True {
                    # "If the spot is in a group, act on all spots in that group, not just the spot we clicked."
                    # "This case statement toggles the selection of the spot/group we clicked, and leaves other spots unchanged if we're holding shift.  Otherwise, we select the spot/group that was clicked and deselect everything else."
                    n495 = stacked-sequence {
                      tunnel: w1835 -> [_ w1843]
                      frame #0 {
                        n496 = local read "Current Spot #"() -> (→"Prev Current Spot":dbl)
                      }
                      frame #1 {
                        "Current Spot #" <- w1843
                      }
                    }
                    n497 = Index Array(array=w1841, index=w1835) -> (element=w1840:T12)
                    n498 = Unbundle(w1840) -> ("Group ID"=w1838:i32)  [unwired: 1 out]
                    n499 = Greater Than 0?(x=w1838) -> (x > 0?=w1839:bool)
                    n500 = for {
                      tunnel: w1841 -> [w1854] mode=indexing
                      tunnel: w1839 -> [w1851]
                      tunnel: w1838 -> [w1850]
                      tunnel: w1835 -> [w1849]
                      tunnel: w1837 -> [w1847]
                      tunnel: [w1845] -> w1836 mode=indexing
                      i -> [w1848]
                      n501 = Unbundle(w1854) -> ("Group ID"=w1844:i32, "Selected"=w1852:bool)
                      n502 = case shown="True" w1851 {
                        tunnel: w1844 -> [_ w1858]
                        tunnel: [w1856 w1860] -> w1846
                        tunnel: w1850 -> [_ w1859]
                        tunnel: w1849 -> [w1857 _]
                        tunnel: w1848 -> [w1855 _]
                        frame False {
                          n503 = Equal?(x=w1855, y=w1857) -> (x = y?=w1856:bool)
                        }
                        frame True {
                          n504 = Equal?(x=w1858, y=w1859) -> (x = y?=w1860:bool)
                        }
                      }
                      n505 = case shown="True" w1847 {
                        tunnel: [w1861 w1862] -> w1853
                        tunnel: w1852 -> [_ w1863]
                        tunnel: w1846 -> [w1861 w1864]
                        frame False {
                        }
                        frame True {
                          n506 = Exclusive Or(1:w1864, 2:w1863) -> (0:w1862:bool)
                        }
                      }
                      n507 = Bundle("Group ID"=w1844, w1853) -> (w1845:cluster{"Group ID":i32, bool})  [unwired: 1 out]
                    }
                  }
                }
              }
              frame True {
                # "convert mouse position to real coords, and add a spot there."
                # "Double-click detected"
                n508 = Unbundle By Name(w1881) -> ("Position (Image Pixels)"=w1880:cluster{"X":dbl, "Y":dbl})
                n509 = for {
                  tunnel: w1879 -> [w1889] mode=indexing
                  tunnel: [w1888] -> w1878 mode=indexing
                  n510 = Bundle(cluster=w1889, "Selected"=FALSE) -> (w1888:T12)  [unwired: 1 in]
                }
                n511 = call "coords_image_to_real_currentimage.vi"("Position (pixels on image)"=w1880) -> ("Position (real coords)"=w1882:cluster{dbl, dbl, "Z":dbl})  [unwired: 9 in]
                n512 = call "replace_position.vi"("Position"=w1882) -> ("Spot"=w1884:T3)  [unwired: 3 in]
                n513 = Build Array (concatenate)(w1886, w1884) -> (w1877:T3[])
                n514 = Build Array (concatenate)(w1878, T12 {"Group ID"=0, "Selected"=TRUE} ("selection_element")) -> (w1885:T12[])
                n515 = Array Size(array=w1877) -> (size(s)=w1876:i32)
                n516 = local write "Induce check"(TRUE) -> ()
                n517 = Subtract(x=w1876, y=1) -> (x-y=w1875:i32)
                n518 = local write "Current Spot #"(w1875) -> ()
              }
            }
          }
        }
        n519 = register-events(reference=w1810, w1809, w1812, w1812, w1812) -> (reference out=w1811:refnum<event-registration>)  [unwired: 1 in, 1 out]
      }
      event Mouse Move {
        n520 = event-data() -> ("Coords"=w1904:T24)  [unwired: 1 in, 2 out]
        n521 = call "mouse_to_image_coords.vi"("Mouse Coords (screen/pane units)"=w1904, "Image Control"=w1903) -> ("Mouse Coords (image pixels)"=w1895:cluster{dbl, dbl})  [unwired: 4 in, 1 out]
        n522 = Not(x=w1894) -> (.not. x?=w1899:bool)
        n523 = case shown="True" w1899 {
          tunnel: w1897 -> [_ w1917]
          tunnel: w1902 -> [w1909 w1919]
          tunnel: w1901 -> [w1908 w1918]
          tunnel: [w1908 w1918] -> w1890
          tunnel: [w1909 w1920] -> w1900
          tunnel: w1895 -> [_ w1911]
          tunnel: w1891 -> [_ w1910]
          frame False {
          }
          frame True {
            # "this is the displacement of the mouse, since the last iteration, in \"real\" coordinates (NB the conversions go before subtracting, as it may involve adding a constant as well as multiplying, which would confuse things as we're only interested in displacements here."
            # "The \"position\" local variable is there just in case we're on the \"current spot\" tab, so that the position updates nicely"
            # "If the user is dragging, translate the spots.\nHolding down shift causes the mouse's motion to be transformed into scaling about the centroid of the spots and rotation about the same point"
            n524 = Unbundle By Name(w1917) -> ("Position (Image Pixels)"=w1912:cluster{"X":dbl, "Y":dbl})
            n525 = call "find_centroid.vi"("Selection and Groups"=w1918, "Spots"=w1919) -> ("centroid"=w1913:cluster{"x":dbl, "y":dbl, "z":dbl})  [unwired: 2 in, 4 out]
            n526 = Unbundle By Name(w1917) -> ("PlatMods.Shift"=w1916:bool)
            n527 = disable-structure shown="Disabled" {
              disable-tunnel: w1913 -> [w1921 _]
              frame Disabled {
                n528 = local write "Position"(w1921) -> ()
              }
              frame Enabled {
              }
            }
            n529 = call "coords_image_to_real_currentimage.vi"("Position (pixels on image)"=w1911) -> ("Position (real coords)"=w1914:cluster{dbl, dbl, "Z":dbl})  [unwired: 9 in]
            n530 = call "coords_image_to_real_currentimage.vi"("Position (pixels on image)"=w1912) -> ("Position (real coords)"=w1915:cluster{dbl, dbl, "Z":dbl})  [unwired: 9 in]
            n531 = case shown="False" w1916 {
              tunnel: [w1926 w2200] -> w1920
              tunnel: w1919 -> [w1932 w2201]
              tunnel: w1918 -> [w1931 w2199]
              tunnel: w1915 -> [w1930 w2186]
              tunnel: w1913 -> [_ w2196]
              tunnel: w1914 -> [w1927 w2187]
              tunnel: w1910 -> [_ _]
              frame False {
                # "Spot Checker passes on information for the bubble collision,system so proper calculations can be made."
                n532 = while {
                  tunnel: w1930 -> [w1971]
                  tunnel: [w1961] -> w1928
                  tunnel: w1927 -> [w1960]
                  i -> [w1954]
                  stop <- w1956 stop-if-true
                  w1946 = 0
                  # "This while loop statement makes sure\nthat every spot gets checked before \nallowing any spot to move."
                  # "Buffer zone controls the amount of space between the\ncenter of a spot compared to the center of another spot.\nThis is used to prevent bubbles from colliding with each other."
                  # "Projected distance calculates the distance between two spots- this is used for when a \"hit\" occurs. If the projected distance becomes larger than the previous distance, the program will assume that the spot is being pulled from the buffer zone and as a result will allow the bubble to exit."
                  # "This subVI leads to the distance function, which outputs the distance between a spot being checked compared to the current spot number."
                  n533 = control-ref of="Value Check"() -> (w1951:refnum<vi>)
                  n534 = control-ref of="ID num check"() -> (w1950:refnum<vi>)
                  n535 = control-ref of="Spot Checker"() -> (w1967:refnum<vi>)
                  n536 = Subtract(x=w1960, y=w1971) -> (x-y=w1961:cluster{dbl, dbl, "Z":dbl})
                  n537 = call "DistanceFunction.vi"("Condition Driver"=FALSE, "Position (real coords)"=w1971, "Current Spot Number"=w1950, "Spot Checker"=w1967, "Spot Number Being Checked"=w1951) -> ("Distance"=w1933:dbl)  [unwired: 6 in]
                  n538 = stacked-sequence {
                    tunnel: w1933 -> [_ w1976]
                    frame #0 {
                      n539 = local read "Distance"() -> (→"Previous Distance":dbl)
                    }
                    frame #1 {
                      "Distance" <- w1976
                    }
                  }
                  n540 = Unbundle(w1961) -> (→"X Displacement":dbl, →"Y Displacement":dbl)  [unwired: 1 out]
                  n541 = control-ref of="ID num check"() -> (w1952:refnum<vi>)
                  n542 = control-ref of="Spot Checker"() -> (w1965:refnum<vi>)
                  n543 = control-ref of="Y Displacement"() -> (w1963:refnum<vi>)
                  n544 = control-ref of="Value Check"() -> (w1953:refnum<vi>)
                  n545 = control-ref of="X Displacement"() -> (w1964:refnum<vi>)
                  n546 = call "ProjectedDistance.vi"("X Displacement"=w1964, "Spot Number Check"=w1953, "Current Spot #"=w1952, "Spot Checker"=w1965, "Y Displacement"=w1963) -> ("Numeric"=→"Projected Distance":dbl)  [unwired: 6 in]
                  n547 = local read "Projected Distance"() -> (w1939:dbl)
                  n548 = Multiply(x="Buffer Zone", y=2) -> (x*y=w1970:dbl)
                  n549 = Less Or Equal?(x=w1933, y=w1970) -> (x <= y?=w1940:bool)
                  n550 = Not Equal?(x=w1939, y=0) -> (x != y?=w1937:bool)
                  n551 = And(x=w1940, y=w1937) -> (x .and. y?=w1934:bool)
                  "Hit" <- w1934
                  n552 = local read "ID num check"() -> (w1947:dbl)
                  n553 = local read "Value Check"() -> (w1948:dbl)
                  n554 = Equal?(x=w1933, y=0) -> (x = y?=w1936:bool)
                  n555 = case shown="False" w1936 {
                    frame False {
                      n556 = local read "Hit"() -> (w1973:bool)
                      n557 = local write "Hit Indicator"(w1973) -> ()
                    }
                    frame True {
                      "Hit Indicator" <- FALSE
                    }
                  }
                  n558 = Equal?(x=w1947, y=w1946) -> (x = y?=w1945:bool)
                  n559 = Equal?(x=w1946, y=w1948) -> (x = y?=w1944:bool)
                  n560 = Not(x=w1934) -> ()  [unwired: 1 out]
                  n561 = And(x=w1945, y=w1944) -> (x .and. y?=w1943:bool)
                  n562 = Or(x=w1934, y=w1943) -> (x .or. y?=w1949:bool)
                  n563 = case shown="True" w1949 {
                    frame False {
                      n564 = stacked-sequence {
                        frame #0 {
                          n565 = local read "Potential Collisions"() -> (w1979:dbl)
                          n566 = local read "Spot # Check"() -> (w1981:dbl)
                          n567 = Subtract(x=w1979, y=1) -> (x-y=w1977:dbl)
                          n568 = Less Or Equal?(x=w1981, y=w1977) -> (x <= y?=w1980:bool)
                          n569 = case shown="True" w1980 {
                            frame False {
                              # "Spot # Check resets if the the number of potential collisons is more than Spot # Check."
                              n570 = local write "Spot # Check"(0) -> ()
                            }
                            frame True {
                              n571 = stacked-sequence {
                                frame #0 {
                                # "Spot # Check increments by 1 every time it is greater than the # of potential collisions."
                                n572 = local read "Spot # Check"() -> (w1985:dbl)
                                n573 = Add(x=w1985, y=1) -> (x+y=→"Spot # Check":dbl)
                                }
                                frame #1 {
                                # "Spot # Check resets if the Spot # Check is eqaul to the # of potential collisions."
                                n574 = local read "Potential Collisions"() -> (w1986:dbl)
                                n575 = local read "Spot # Check"() -> (w1987:dbl)
                                n576 = Equal?(x=w1987, y=w1986) -> (x = y?=w1988:bool)
                                n577 = case shown="True" w1988 {
                                frame False {
                                }
                                frame True {
                                n578 = local write "Spot # Check"(0) -> ()
                                }
                                }
                                }
                                frame #2 {
                                n579 = local read "Spot Checker"() -> (w2003:T3[])
                                n580 = local read "Current Spot #"() -> (w2004:dbl)
                                n581 = local read "Area to check"() -> (w1990:dbl)
                                n582 = Index Array(array=w2003, index=w2004) -> (element=w2002:T3)
                                n583 = local read "Orig Y SC"() -> (w1999:dbl)
                                n584 = Unbundle By Name(w2002) -> ("Position.x"=w2000:dbl, "Position.y"=w1998:dbl)
                                n585 = local read "Orig X SC"() -> (w2001:dbl)
                                n586 = Subtract(x=w1998, y=w1999) -> (x-y=w1991:dbl)
                                n587 = Absolute Value(x=w1991) -> (abs(x)=w1992:dbl)
                                n588 = Subtract(x=w2000, y=w2001) -> (x-y=w1994:dbl)
                                n589 = Greater?(x=w1992, y=w1990) -> (0:w1996:bool)
                                n590 = Absolute Value(x=w1994) -> (abs(x)=w1993:dbl)
                                n591 = Greater?(x=w1993, y=w1990) -> (0:w1995:bool)
                                n592 = Or(x=w1995, y=w1996) -> (x .or. y?=w1997:bool)
                                n593 = case shown="True" w1997 {
                                frame False {
                                }
                                frame True {
                                n594 = stacked-sequence {
                                frame #0 {
                                n595 = local read "Null array"() -> (w2009:dbl[])
                                n596 = local write "What to Check"(w2009) -> ()
                                n597 = local write "ID"(w2009) -> ()
                                n598 = local read "Current Spot #"() -> (w2011:dbl)
                                n599 = local write "Potential Collisions"(0) -> ()
                                n600 = local read "Spot Checker"() -> (w2010:T3[])
                                n601 = Index Array(array=w2010, index=w2011) -> (element=w2012:T3)
                                n602 = Wait (ms)(milliseconds to wait=100) -> ()  [unwired: 1 out]
                                n603 = Unbundle By Name(w2012) -> ("Position.x"=w2006:dbl, "Position.y"=w2007:dbl)
                                n604 = local write "Orig Y SC"(w2007) -> ()
                                n605 = local write "Orig X SC"(w2006) -> ()
                                }
                                frame #1 {
                                # "All this is a  statement checking whether the microrobot is within the area being checked using absolute value statements. The number of potential collisions gets added by 1 every time a bubble is detected within the area."
                                n606 = local read "# of Spots"() -> (w2013:dbl)
                                n607 = for {
                                N: w2013 -> [_]
                                tunnel: w2013 -> [w2018]
                                i -> [w2014]
                                n608 = local read "Selection/Group"() -> (w2017:T12[])
                                n609 = Index Array(array=w2017, index=w2014) -> (element=w2016:T12)
                                n610 = Unbundle By Name(w2016) -> ("Selected"=w2015:bool)
                                n611 = case shown="True" w2015 {
                                tunnel: w2018 -> [_ w2020]
                                tunnel: w2014 -> [_ w2019]
                                frame False {
                                }
                                frame True {
                                n612 = for {
                                N: w2020 -> [_]
                                tunnel: w2019 -> [w2021]
                                i -> [w2022]
                                n613 = local read "Selection/Group"() -> (w2026:T12[])
                                n614 = Index Array(array=w2026, index=w2022) -> (element=w2025:T12)
                                n615 = Unbundle By Name(w2025) -> ("Selected"=w2023:bool)
                                n616 = Not(x=w2023) -> (.not. x?=w2024:bool)
                                n617 = case shown="True" w2024 {
                                tunnel: w2022 -> [_ w2030]
                                tunnel: w2021 -> [_ w2029]
                                tunnel: w2021 -> [_ w2028]
                                frame False {
                                }
                                frame True {
                                n618 = local read "Spot Checker"() -> (w2047:T3[])
                                n619 = Index Array(array=w2047, index=w2030) -> (element=w2048:T3)
                                n620 = Index Array(array=w2047, index=w2029) -> (element=w2046:T3)
                                n621 = Unbundle By Name(w2046) -> ("Position.x"=w2043:dbl, "Position.y"=w2039:dbl)
                                n622 = Unbundle By Name(w2048) -> ("Position.x"=w2040:dbl, "Position.y"=w2036:dbl)
                                n623 = local read "Area+ Buffer"() -> (w2027:dbl)
                                n624 = Subtract(x=w2043, y=w2027) -> (x-y=w2044:dbl)
                                n625 = Greater Or Equal?(x=w2040, y=w2044) -> (x >= y?=w2045:bool)
                                n626 = Add(x=w2039, y=w2027) -> (x+y=w2038:dbl)
                                n627 = Subtract(x=w2039, y=w2027) -> (x-y=w2037:dbl)
                                n628 = Add(x=w2043, y=w2027) -> (x+y=w2041:dbl)
                                n629 = Less Or Equal?(x=w2036, y=w2038) -> (x <= y?=w2035:bool)
                                n630 = Greater Or Equal?(x=w2036, y=w2037) -> (x >= y?=w2034:bool)
                                n631 = Less Or Equal?(x=w2040, y=w2041) -> (x <= y?=w2042:bool)
                                n632 = And(x=w2045, y=w2042) -> (x .and. y?=w2032:bool)
                                n633 = And(x=w2035, y=w2034) -> (x .and. y?=w2033:bool)
                                n634 = And(x=w2032, y=w2033) -> (x .and. y?=w2031:bool)
                                n635 = case shown="True" w2031 {
                                tunnel: w2030 -> [_ _]
                                tunnel: w2030 -> [_ w2050]
                                tunnel: w2028 -> [_ w2049]
                                frame False {
                                }
                                frame True {
                                n636 = stacked-sequence {
                                tunnel: w2050 -> [w2051 _]
                                tunnel: w2049 -> [w2052 _]
                                frame #0 {
                                n637 = local read "Potential Collisions"() -> (w2055:dbl)
                                n638 = local read "What to Check"() -> (w2056:dbl[])
                                n639 = Insert Into Array(array=w2056, index=w2055, new element=w2051) -> (w2057:dbl[])
                                n640 = local read "ID"() -> (w2054:dbl[])
                                n641 = local write "What to Check"(w2057) -> ()
                                n642 = Insert Into Array(array=w2054, index=w2055, new element=w2052) -> (w2053:dbl[])
                                n643 = local write "ID"(w2053) -> ()
                                }
                                frame #1 {
                                n644 = local read "Potential Collisions"() -> (w2060:dbl)
                                n645 = Add(x=w2060, y=1) -> (x+y=w2058:dbl)
                                n646 = local write "Potential Collisions"(w2058) -> ()
                                }
                                }
                                }
                                }
                                }
                                }
                                }
                                }
                                }
                                }
                                }
                                frame #2 {
                                n647 = local read "Current Spot #"() -> (w2061:dbl)
                                n648 = local write "Prev Current Spot"(w2061) -> ()
                                }
                                }
                                }
                                }
                                }
                              }
                            }
                          }
                        }
                        frame #1 {
                          # "This updates the ID and Value being checked at the beginning of IDs and values being checked."
                          n649 = local read "Spot # Check"() -> (w2064:dbl)
                          n650 = local read "What to Check"() -> (w2065:dbl[])
                          n651 = local read "ID"() -> (w2066:dbl[])
                          n652 = Index Array(array=w2066, index=w2064) -> (element=w2063:dbl)
                          n653 = Index Array(array=w2065, index=w2064) -> (element=w2062:dbl)
                          n654 = local write "Value Check"(w2062) -> ()
                          n655 = local write "ID num check"(w2063) -> ()
                        }
                      }
                    }
                    frame True {
                      n656 = stacked-sequence {
                        frame #0 {
                          # "This section activate a case statement which allows us to change the area being checked. Orig X/Y SC holds the position of the area to check and changes after the bubble exits the area beig checked."
                          # "This statement controls the areas selected and finds which bubbles needs to be checked. This activates when the bubble\nmoves out of the area specified."
                          n657 = local read "# of Spots"() -> (w2086:dbl)
                          n658 = local read "Current Spot #"() -> (w2085:dbl)
                          n659 = Subtract(x=w2086, y=1) -> (x-y=w2087:dbl)
                          n660 = Equal?(x=w2085, y=w2087) -> (x = y?=w2083:bool)
                          n661 = case shown="True" w2083 {
                            tunnel: [w2146 w2149] -> w2084
                            frame True {
                              n662 = local read "# of Spots"() -> (w2147:dbl)
                              n663 = Subtract(x=w2147, y=2) -> (x-y=w2146:dbl)
                            }
                            frame False {
                              n664 = local read "# of Spots"() -> (w2148:dbl)
                              n665 = Subtract(x=w2148, y=1) -> (x-y=w2149:dbl)
                            }
                          }
                          "Maximum" <- w2084
                          n666 = local read "Spot Checker"() -> (w2082:T3[])
                          n667 = local read "Current Spot #"() -> (w2081:dbl)
                          n668 = Index Array(array=w2082, index=w2081) -> (element=w2080:T3)
                          n669 = Unbundle By Name(w2080) -> ("Position.x"=w2079:dbl, "Position.y"=w2078:dbl)
                          n670 = local read "Orig Y SC"() -> (w2076:dbl)
                          n671 = local read "Orig X SC"() -> (w2077:dbl)
                          n672 = Subtract(x=w2078, y=w2076) -> (x-y=w2073:dbl)
                          n673 = Subtract(x=w2079, y=w2077) -> (x-y=w2075:dbl)
                          n674 = Absolute Value(x=w2073) -> (abs(x)=w2072:dbl)
                          n675 = Absolute Value(x=w2075) -> (abs(x)=w2074:dbl)
                          n676 = local read "Area to check"() -> (w2068:dbl)
                          n677 = local read "Area to check"() -> (w2067:dbl)
                          n678 = Greater?(x=w2074, y=w2068) -> (0:w2071:bool)
                          n679 = Greater?(x=w2072, y=w2067) -> (0:w2070:bool)
                          n680 = Or(x=w2071, y=w2070) -> (x .or. y?=w2069:bool)
                          n681 = case shown="True" w2069 {
                            frame False {
                            }
                            frame True {
                              n682 = stacked-sequence {
                                frame #0 {
                                # "A small time delay of 100 ms is provided to allow the data to pass throguh properly."
                                n683 = Wait (ms)(milliseconds to wait=100) -> ()  [unwired: 1 out]
                                n684 = local read "Null array"() -> (→"What to Check" →"ID":dbl[])
                                n685 = local read "Spot Checker"() -> (w2094:T3[])
                                n686 = local read "Current Spot #"() -> (w2093:dbl)
                                n687 = Index Array(array=w2094, index=w2093) -> (element=w2092:T3)
                                n688 = Unbundle By Name(w2092) -> ("Position.x"=→"Orig X SC":dbl, "Position.y"=→"Orig Y SC":dbl)
                                "Potential Collisions" <- 0
                                }
                                frame #1 {
                                n689 = local read "# of Spots"() -> (w2097:dbl)
                                n690 = for {
                                N: w2097 -> [_]
                                tunnel: w2097 -> [w2102]
                                i -> [w2098]
                                n691 = local read "Selection/Group"() -> (w2101:T12[])
                                n692 = Index Array(array=w2101, index=w2098) -> (element=w2100:T12)
                                n693 = Unbundle By Name(w2100) -> ("Selected"=w2099:bool)
                                n694 = case shown="True" w2099 {
                                tunnel: w2102 -> [_ w2104]
                                tunnel: w2098 -> [_ w2103]
                                frame False {
                                }
                                frame True {
                                n695 = for {
                                N: w2104 -> [_]
                                tunnel: w2103 -> [w2105]
                                i -> [w2106]
                                n696 = local read "Selection/Group"() -> (w2110:T12[])
                                n697 = Index Array(array=w2110, index=w2106) -> (element=w2109:T12)
                                n698 = Unbundle By Name(w2109) -> ("Selected"=w2107:bool)
                                n699 = Not(x=w2107) -> (.not. x?=w2108:bool)
                                n700 = case shown="True" w2108 {
                                tunnel: w2106 -> [_ w2114]
                                tunnel: w2105 -> [_ w2113]
                                tunnel: w2105 -> [_ w2112]
                                frame False {
                                }
                                frame True {
                                n701 = local read "Spot Checker"() -> (w2131:T3[])
                                n702 = Index Array(array=w2131, index=w2114) -> (element=w2132:T3)
                                n703 = Index Array(array=w2131, index=w2113) -> (element=w2130:T3)
                                n704 = Unbundle By Name(w2130) -> ("Position.x"=w2127:dbl, "Position.y"=w2123:dbl)
                                n705 = Unbundle By Name(w2132) -> ("Position.x"=w2124:dbl, "Position.y"=w2120:dbl)
                                n706 = local read "Area+ Buffer"() -> (w2111:dbl)
                                n707 = Subtract(x=w2127, y=w2111) -> (x-y=w2128:dbl)
                                n708 = Greater Or Equal?(x=w2124, y=w2128) -> (x >= y?=w2129:bool)
                                n709 = Add(x=w2123, y=w2111) -> (x+y=w2122:dbl)
                                n710 = Subtract(x=w2123, y=w2111) -> (x-y=w2121:dbl)
                                n711 = Add(x=w2127, y=w2111) -> (x+y=w2125:dbl)
                                n712 = Less Or Equal?(x=w2120, y=w2122) -> (x <= y?=w2119:bool)
                                n713 = Greater Or Equal?(x=w2120, y=w2121) -> (x >= y?=w2118:bool)
                                n714 = Less Or Equal?(x=w2124, y=w2125) -> (x <= y?=w2126:bool)
                                n715 = And(x=w2129, y=w2126) -> (x .and. y?=w2116:bool)
                                n716 = And(x=w2119, y=w2118) -> (x .and. y?=w2117:bool)
                                n717 = And(x=w2116, y=w2117) -> (x .and. y?=w2115:bool)
                                n718 = case shown="True" w2115 {
                                tunnel: w2114 -> [_ _]
                                tunnel: w2114 -> [_ w2134]
                                tunnel: w2112 -> [_ w2133]
                                frame False {
                                }
                                frame True {
                                n719 = stacked-sequence {
                                tunnel: w2134 -> [w2135 _]
                                tunnel: w2133 -> [w2136 _]
                                frame #0 {
                                n720 = local read "Potential Collisions"() -> (w2139:dbl)
                                n721 = local read "What to Check"() -> (w2140:dbl[])
                                n722 = Insert Into Array(array=w2140, index=w2139, new element=w2135) -> (w2141:dbl[])
                                n723 = local read "ID"() -> (w2138:dbl[])
                                n724 = Insert Into Array(array=w2138, index=w2139, new element=w2136) -> (w2137:dbl[])
                                n725 = local write "What to Check"(w2141) -> ()
                                n726 = local write "ID"(w2137) -> ()
                                }
                                frame #1 {
                                n727 = local read "Potential Collisions"() -> (w2144:dbl)
                                n728 = Add(x=w2144, y=1) -> (x+y=w2142:dbl)
                                n729 = local write "Potential Collisions"(w2142) -> ()
                                }
                                }
                                }
                                }
                                }
                                }
                                }
                                }
                                }
                                }
                                }
                              }
                            }
                          }
                        }
                        frame #1 {
                          n730 = local read "# of Spots"() -> (w2153:dbl)
                          n731 = Not Equal?(x=w2153, y=1) -> (x != y?=w2151:bool)
                          n732 = case shown="True" w2151 {
                            frame False {
                            }
                            frame True {
                              n733 = stacked-sequence {
                                frame #0 {
                                n734 = local read "Potential Collisions"() -> (w2156:dbl)
                                n735 = local read "Spot # Check"() -> (w2158:dbl)
                                n736 = Subtract(x=w2156, y=1) -> (x-y=w2154:dbl)
                                n737 = Less Or Equal?(x=w2158, y=w2154) -> (x <= y?=w2157:bool)
                                n738 = case shown="False" w2157 {
                                frame False {
                                n739 = local write "Spot # Check"(0) -> ()
                                }
                                frame True {
                                }
                                }
                                }
                                frame #1 {
                                n740 = local read "What to Check"() -> (w2164:dbl[])
                                n741 = local read "ID"() -> (w2162:dbl[])
                                n742 = local read "Spot # Check"() -> (w2160:dbl)
                                n743 = Index Array(array=w2164, index=w2160) -> (element=→"Value Check":dbl)
                                n744 = Index Array(array=w2162, index=w2160) -> (element=→"ID num check":dbl)
                                }
                              }
                            }
                          }
                        }
                      }
                    }
                  }
                  n745 = local read "Potential Collisions"() -> (w1941:dbl)
                  n746 = Subtract(x=w1941, y=1) -> (x-y=w1942:dbl)
                  n747 = local read "Hit"() -> (w1959:bool)
                  n748 = Equal?(x=w1954, y=w1942) -> (x = y?=w1958:bool)
                  n749 = Or(x=w1959, y=w1958) -> (x .or. y?=w1956:bool)
                }
                n750 = for {
                  tunnel: w1931 -> [w2178] mode=indexing
                  tunnel: w1932 -> [w2175] mode=indexing
                  tunnel: [w2177] -> w1926 mode=indexing
                  tunnel: w1928 -> [w2176]
                  # "If the projected distance is greater than the\nprevious distance, then the selected spots will move. \nThis situation only occurs if the bubble is about to/crossing \nthe buffer zone of another bubble. \n\nThe selected spots will also move if none of the bubbles\nare near/crossing the buffer zone of another bubble."
                  n751 = local read "Hit"() -> (w2168:bool)
                  n752 = Unbundle By Name(w2175) -> ()  [unwired: 1 out]
                  n753 = local read "Projected Distance"() -> (w2167:dbl)
                  n754 = Unbundle(w2178) -> ("Group ID"=→"Group ID #":i32, "Selected"=w2172:bool)
                  n755 = local read "Previous Distance"() -> (w2170:dbl)
                  n756 = Not(x=w2168) -> (.not. x?=w2166:bool)
                  n757 = Greater?(x=w2167, y=w2170) -> (0:w2169:bool)
                  n758 = And(x=w2168, y=w2169) -> (x .and. y?=w2165:bool)
                  n759 = Or(x=w2166, y=w2165) -> (x .or. y?=w2171:bool)
                  n760 = And(x=w2172, y=w2171) -> (x .and. y?=w2173:bool)
                  n761 = case shown="True" w2173 {
                    tunnel: w2175 -> [w2179 w2183]
                    tunnel: [w2179 w2182] -> w2177
                    tunnel: w2176 -> [_ w2184]
                    frame False {
                      # "otherwise, leave it alone!"
                    }
                    frame True {
                      # "If the spot is selected, move it by the same amount as the mouse"
                      n762 = call "extract_position.vi"("Spot"=w2183) -> ("Position"=w2181:cluster{"x":dbl, "y":dbl, "z":dbl})
                      n763 = Add(x=w2181, y=w2184) -> (x+y=w2180:cluster{dbl, dbl, dbl})
                      n764 = call "replace_position.vi"("Position"=w2180, "Spot in"=w2183) -> ("Spot"=w2182:T3)  [unwired: 2 out]
                    }
                  }
                }
                "Spot Checker" <- w1926
                n765 = local read "Locked Current Spot"() -> (w1922:dbl)
                n766 = Index Array(array=w1926, index=w1922) -> (element=w1925:T3)
                n767 = Unbundle By Name(w1925) -> ("Position.x"=→"New X":dbl, "Position.y"=→"New Y":dbl)  [unwired: 1 out]
                n768 = Array Size(array=w1926) -> (size(s)=→"# of Spots":i32)
              }
              frame True {
                # "coordinate conversion to find the rotation and scaling done by the mouse, about the centroid of the spots"
                n769 = Subtract(x=w2186, y=w2196) -> (x-y=w2205:cluster{dbl, dbl, dbl})
                n770 = Subtract(x=w2187, y=w2196) -> (x-y=w2204:cluster{dbl, dbl, dbl})
                n771 = Unbundle(w2204) -> (w2190:dbl, w2191:dbl)  [unwired: 1 out]
                n772 = Unbundle(w2205) -> (w2195:dbl, w2194:dbl)  [unwired: 1 out]
                n773 = Re/Im To Polar(2:w2191, 3:w2190) -> (0:w2188:dbl, 1:w2189:dbl)
                n774 = Re/Im To Polar(2:w2194, 3:w2195) -> (0:w2192:dbl, 1:w2193:dbl)
                n775 = Divide(x=w2189, y=w2193) -> (x/y=w2185:dbl)
                n776 = Subtract(x=w2188, y=w2192) -> (x-y=w2197:dbl)
                n777 = Bundle(w2185, w2185, w2185) -> (w2207:cluster{dbl, dbl, dbl})  [unwired: 1 out]
                n778 = call "scale_matrix.vi"("Scale Factors"=w2207) -> ("Scale Matrix"=w2203:T7)
                n779 = call "arb_rotation_matrix.vi"("Unit Vector"=cluster{dbl, dbl, dbl} {0.0, 0.0, 1.0}, "theta"=w2197) -> ("Real Matrix"=w2202:T7)
                n780 = call-poly <vilib>:"A x B.vi"("B"=w2202, "A"=w2203) -> ("A x B"=w2198:T7)  [unwired: 1 out]
                n781 = for {
                  tunnel: w2201 -> [w2213] mode=indexing
                  tunnel: [w2212] -> w2200 mode=indexing
                  tunnel: w2199 -> [w2211] mode=indexing
                  tunnel: w2196 -> [w2209]
                  tunnel: w2198 -> [w2208]
                  n782 = Unbundle(w2211) -> ("Selected"=w2210:bool)  [unwired: 1 out]
                  n783 = case shown="True" w2210 {
                    tunnel: w2213 -> [w2214 w2218]
                    tunnel: [w2214 w2217] -> w2212
                    tunnel: w2209 -> [_ w2216]
                    tunnel: w2208 -> [_ w2215]
                    frame False {
                    }
                    frame True {
                      n784 = call "apply_matrix_transformation_to_spots.vi"("Transform centre (i.e. transform about this point)"=w2216, "Transformation Matrix (3x3)"=w2215, "Spot In"=w2218) -> ("Spot Out"=w2217:T3)  [unwired: 5 out]
                    }
                  }
                }
              }
            }
          }
        }
        "Selection/Group" <- w1890
        n785 = Unbundle By Name(w1897) -> ("Position (Image Pixels)"=w1896:cluster{"X":dbl, "Y":dbl})
        n786 = Bundle By Name(cluster=w1897, "Dragging"=TRUE, "Previous Position (Image Pixels)"=w1896, "Position (Image Pixels)"=w1895) -> (w1906:T13)
      }
      event "stop": Value Change {
        n787 = event-data() -> ()  [unwired: 1 in, 4 out]
        n788 = global read "red_tweezers_globals_INTERNAL_VOLATILE.vi" "Current Settings File"() -> (w2222:path)
        n789 = call <vilib>:"Check if File or Folder Exists.vi"("path"=w2222) -> ("file or folder exists?"=w2221:bool)  [unwired: 8 in, 2 out]
        n790 = case shown="False" w2221 {
          tunnel: [w2229 w2233] -> w2223
          frame False {
            n791 = Two Button Dialog(message="Save current settings?", 1:"Don't Save" ("F button name (\"Cancel\")"), 2:"Save As..." ("T button name (\"OK\")")) -> (T button?=w2226:bool)
            n792 = Select(t=T18."Center Button" ("Which Button?"), s=w2226, f=T18."Right Button" ("Which Button?")) -> (s? t:f=w2229:T18)
          }
          frame True {
            n793 = call <vilib>:"Three Button Dialog.vi"("Allow user to close window? (TRUE)"=TRUE, "Window Title (\"\")"="Save Settings?" ("Window Title (\"\")"), "Right Button Text (\"Cancel\")"="No" ("Right Button Text (\"Cancel\")"), "Center Button Text (\"No\")"="Save As..." ("Center Button Text (\"No\")"), "Left Button Text (\"Yes\")"="Save" ("Left Button Text (\"Yes\")"), "message"="Would you like to save the current settings? You can choose to use the current settings file or save to a new location.") -> ("Which Button?"=w2233:T18)  [unwired: 5 in]
          }
        }
        n794 = case shown="\"Center Button\"" w2223 {
          tunnel: [TRUE TRUE FALSE FALSE] -> w2220
          frame "Left Button", Default {
          }
          frame "Center Button" {
            n795 = call "File Dialog5"("prompt"="Please select a location to save the settings", "button label"="Save", "default name"="red_tweezers_settings.xml", "pattern (all files)"="*.xml" ("pattern label"), "pattern label"="XML Settings Files") -> ("selected path"=w2241:path)  [unwired: 7 in, 3 out]
            n796 = global write "red_tweezers_globals_INTERNAL_VOLATILE.vi" "Current Settings File"(w2241) -> ()
          }
          frame "Right Button" {
          }
          frame "Window Close" {
          }
        }
        n797 = global write "red_tweezers_globals_INTERNAL_VOLATILE.vi" "Save Settings On Exit"(w2220) -> ()
      }
    }
    n798 = case shown="1" "ROI points" {
      frame 0, Default {
        # "ROI point 0 is not used"
        n799 = local read "ROI Y"() -> (w279:dbl)
        "ROI new Mpy" <- w279
        n800 = local read "ROI X"() -> (w280:dbl)
        "ROI new MPx" <- w280
        n801 = Build Array(w280, w279) -> (→"ROI Point 0":T7)
      }
      frame 1 {
        n802 = local read "Object MP Y"() -> (w286:dbl)
        n803 = local read "Object MP X"() -> (w287:dbl)
        n804 = local read "ROI Y"() -> (w283:dbl)
        "ROI y1" <- w283
        "NewY1" <- w283
        n805 = local read "ROI X"() -> (w282:dbl)
        "ROI x1" <- w282
        "NewX1" <- w282
        n806 = Subtract(x=w283, y=w286) -> (x-y=→"Radius ROI y1":dbl)
        n807 = Subtract(x=w282, y=w287) -> (x-y=→"Radius ROI x1":dbl)
        n808 = Build Array(w282, w283) -> (→"ROI Point 1":T7)
      }
      frame 2 {
        n809 = local read "Object MP Y"() -> (w293:dbl)
        n810 = local read "Object MP X"() -> (w294:dbl)
        n811 = local read "ROI Y"() -> (w290:dbl)
        "ROI y2" <- w290
        "NewY2" <- w290
        n812 = local read "ROI X"() -> (w289:dbl)
        "ROI x2" <- w289
        "NewX2" <- w289
        n813 = Subtract(x=w290, y=w293) -> (x-y=→"Radius ROI y2":dbl)
        n814 = Subtract(x=w289, y=w294) -> (x-y=→"Radius ROI x2":dbl)
        n815 = Build Array(w289, w290) -> (→"ROI Point 2":T7)
      }
      frame 3 {
        n816 = local read "Object MP Y"() -> (w300:dbl)
        n817 = local read "Object MP X"() -> (w301:dbl)
        n818 = local read "ROI Y"() -> (w296:dbl)
        "ROI y3" <- w296
        n819 = local read "ROI X"() -> (w297:dbl)
        "ROI x3" <- w297
        n820 = Subtract(x=w296, y=w300) -> (x-y=→"Radius ROI y3":dbl)
        n821 = Subtract(x=w297, y=w301) -> (x-y=→"Radius ROI x3":dbl)
        n822 = Build Array(w297, w296) -> (→"ROI Point 3":T7)
      }
      frame 4 {
        n823 = local read "Object MP Y"() -> (w308:dbl)
        n824 = local read "Object MP X"() -> (w307:dbl)
        n825 = local read "ROI Y"() -> (w303:dbl)
        "ROI y4" <- w303
        n826 = local read "ROI X"() -> (w304:dbl)
        "ROI x4" <- w304
        n827 = Subtract(x=w303, y=w308) -> (x-y=→"Radius ROI y4":dbl)
        n828 = Subtract(x=w304, y=w307) -> (x-y=→"Radius ROI x4":dbl)
        n829 = Build Array(w304, w303) -> (→"ROI Point 4":T7)
      }
      frame 5 {
        n830 = local read "Object MP Y"() -> (w315:dbl)
        n831 = local read "Object MP X"() -> (w314:dbl)
        n832 = local read "ROI Y"() -> (w311:dbl)
        "ROI y5" <- w311
        n833 = local read "ROI X"() -> (w310:dbl)
        "ROI x5" <- w310
        n834 = Subtract(x=w311, y=w315) -> (x-y=→"Radius ROI y5":dbl)
        n835 = Subtract(x=w310, y=w314) -> (x-y=→"Radius ROI x5":dbl)
        n836 = Build Array(w310, w311) -> (→"ROI point 5":T7)
      }
      frame 6 {
        n837 = local read "Object MP Y"() -> (w322:dbl)
        n838 = local read "Object MP X"() -> (w321:dbl)
        n839 = local read "ROI Y"() -> (w317:dbl)
        "ROI y6" <- w317
        n840 = local read "ROI X"() -> (w318:dbl)
        "ROI x6" <- w318
        n841 = Subtract(x=w317, y=w322) -> (x-y=→"Radius ROI y6":dbl)
        n842 = Subtract(x=w318, y=w321) -> (x-y=→"Radius ROI x6":dbl)
        n843 = Build Array(w318, w317) -> (→"ROI Point 6":T7)
      }
      frame 7 {
      }
    }
    n844 = call "IMAQ Create"("Image Name"="untitled", "Image Type"=w90) -> ("New Image"=w89:T8)  [unwired: 3 in, 1 out]
    n845 = call "Vision Acquisition"() -> ("Image Out"=w33:T8)  [unwired: 24 in, 3 out]
    n846 = call "IMAQ ExtractSingleColorPlane"("Color Plane"=w88, "Image Dst"=w89, "Image Src"=w33) -> ("Image Dst Out"=w32:T8)  [unwired: 7 in, 1 out]
    n847 = case shown="True" "ROI switch" {
      tunnel: w33 -> [w325 w365]
      frame False {
        n848 = local read "Number of Matches Returned"() -> (w324:dbl)
        n849 = Add(x=w324, y=1.0 ("x+y")) -> (x+y=w326:dbl)
        n850 = for {
          N: w326 -> [_]
          tunnel: w325 -> [w334]
          i -> [w360]
          w332 = 1e-07  # y
          w333 = 1e-07  # y
          n851 = property on="Camera 3" class="ImageControl"() -> ("ROI"=w335:T27)  [unwired: 2 in, 2 out]
          n852 = Unbundle By Name(w335) -> ("Contours"=w344:T28)
          n853 = local read "Circles 2"() -> (w347:T2)
          n854 = Number To Decimal String(number=w360) -> (decimal integer string=w359:string)  [unwired: 1 in]
          n855 = Index Array(array=w347) -> (element=w364:T29)  [unwired: 1 in]
          n856 = Index Array(array=w344) -> (element=w343:T30)  [unwired: 1 in]
          n857 = Unbundle(w364) -> ("Position"=w358:cluster{"X":sgl, "Y":sgl}, "Radius"=w346:dbl)  [unwired: 1 out]
          "Radius" <- w346
          n858 = Unbundle By Name(w343) -> ("Points"=w342:i32[])
          n859 = Unbundle(w358) -> ("X"=w362:sgl, "Y"=w361:sgl)
          n860 = Subtract(x=w362, y=w346) -> (x-y=→"toplx 2":dbl)
          n861 = Add(x=w362, y=w346) -> (x+y=→"bottomrx 2":dbl)
          n862 = Add(x=w361, y=w346) -> (x+y=→"bottomry 2":dbl)
          n863 = Subtract(x=w361, y=w346) -> (x-y=→"toply 2":dbl)
          n864 = Index Array(array=w342, index #1=0 ("index"), index #2=1 ("index")) -> (element #1=w331:i32, element #2=w329:i32)
          n865 = Bundle(w331, w329) -> (w339:cluster{i32, i32})  [unwired: 1 in]
          "Specific Point 2" <- w339
          n866 = call "IMAQ Overlay Text"("Text Color (black)"=u32 1703680, "Font, Size & Style"=T14 {"Desired Font (Application)"=enum."Application Font", "[User-specified Font]"={"Font Name"="", "Size"=40, "Strikeout?"=FALSE, "Italic?"=FALSE, "Underline?"=FALSE, "Outline?"=FALSE, "Shadow?"=FALSE, "Bold?"=FALSE, "Rotation Angle"=0.0}, "Horizontal Alignment"=0, "Vertical Alignment"=0}, "String"="ROI", "Origin"=w339, "Image"=w334) -> ()  [unwired: 5 in, 2 out]
          n867 = Multiply(x=w331, y=w332) -> (x*y=w330:dbl)
          n868 = Multiply(x=w329, y=w333) -> (x*y=w328:dbl)
          n869 = local read "toply 2"() -> (w350:dbl)
          n870 = local read "bottomrx 2"() -> (w349:dbl)
          n871 = local read "toplx 2"() -> (w351:dbl)
          n872 = local read "bottomry 2"() -> (w348:dbl)
          n873 = local write "ROI X"(w330) -> ()
          n874 = local write "ROI Y"(w328) -> ()
          n875 = Build Array(w351, w350, w349, w348) -> (w356:dbl[])
          n876 = Array To Cluster(array=w356) -> (cluster=w363:T31)
          n877 = call "IMAQ Overlay Oval"("Bounding Rectangle"=w363, "Image"=w334) -> ("Image Out"=w357:T8)  [unwired: 8 in, 1 out]
          n878 = call "IMAQ Overlay Text"("String"=w359, "Origin"=w358, "Image"=w357) -> ("Image Out"=→"Camera 3":T8)  [unwired: 7 in, 1 out]
        }
      }
      frame True {
        # "This is the code for ROI and Object detection"
        n879 = local read "Number of Objects"() -> (w367:i32)
        n880 = Add(x=w367, y=1.0 ("x+y")) -> (x+y=w366:dbl)
        n881 = for {
          N: w366 -> [_]
          tunnel: w365 -> [w382]
          w373 = 1e-07  # y
          w374 = 1e-07  # y
          # "This part of the\ncode detects \nobeject"
          # "This is the ROI, a specific point selected"
          # "This part of the code will obtain the Midpoint"
          n882 = property on="Camera 3" class="ImageControl"() -> ("ROI"=w381:T27)  [unwired: 2 in, 2 out]
          n883 = local read "Objects"() -> (w378:T1)
          n884 = Unbundle By Name(w381) -> ("Contours"=w391:T28)
          n885 = Index Array(array=w378) -> (element=w379:T32)  [unwired: 1 in]
          n886 = call "IMAQ Count Objects 2"("Settings"="Settings", "Image"=w382) -> ("Number of Objects"=→"Number of Objects":i32, "Image Out"=w394:T8, "Objects"=→"Objects":T1)  [unwired: 5 in, 2 out]
          n887 = local write "Camera 3"(w394) -> ()
          n888 = Index Array(array=w391) -> (element=w390:T30)  [unwired: 1 in]
          n889 = Unbundle(w379) -> ("Object Center"=w377:cluster{"X":sgl, "Y":sgl})  [unwired: 5 out]
          n890 = Unbundle By Name(w390) -> ("Points"=w389:i32[])
          n891 = Unbundle(w377) -> ("X"=→"Object MP X":sgl, "Y"=→"Object MP Y":sgl)
          n892 = Index Array(array=w389, index #1=0 ("index"), index #2=1 ("index")) -> (element #1=w370:i32, element #2=w372:i32)
          n893 = Multiply(x=w370, y=w374) -> (x*y=→"ROI X":dbl)
          n894 = Multiply(x=w372, y=w373) -> (x*y=→"ROI Y":dbl)
          n895 = Bundle(w370, w372) -> (w386:cluster{i32, i32})  [unwired: 1 in]
          "Specific Point" <- w386
          n896 = call "IMAQ Overlay Text"("Text Color (black)"=u32 1703680, "Font, Size & Style"=T14 {"Desired Font (Application)"=enum."Application Font", "[User-specified Font]"={"Font Name"="", "Size"=40, "Strikeout?"=FALSE, "Italic?"=FALSE, "Underline?"=FALSE, "Outline?"=FALSE, "Shadow?"=FALSE, "Bold?"=FALSE, "Rotation Angle"=0.0}, "Horizontal Alignment"=0, "Vertical Alignment"=0}, "String"="ROI", "Origin"=w386, "Image"=w382) -> ()  [unwired: 5 in, 2 out]
        }
      }
    }
    n897 = call-poly "IMAQ Detect Shapes"("Circle Descriptor"="Circle Descriptor 2", "Image"=w32) -> ("Number of Matches Returned"=→"Number of Matches Returned":i32, "Circles"=→"Circles 2":T2)  [unwired: 7 in, 1 out]
    n898 = property on="Image" class="ImageControl"() -> ("ROI"=w61:T27)  [unwired: 2 in, 2 out]
    n899 = Unbundle By Name(w61) -> ("Contours"=w57:T28)
    n900 = Index Array(array=w57) -> (element=w58:T30)  [unwired: 1 in]
    n901 = Unbundle By Name(w58) -> ("Points"=w59:i32[])
    n902 = Index Array(array=w59, index #1=0 ("index")) -> (element #1=→"Numeric 3":i32, element #2=→"Numeric 2":i32)  [unwired: 1 in]
    n903 = case shown="True" "Camera Capture 2" {
      frame False {
      }
      frame True {
        n904 = local read "Circles 2"() -> (w397:T2)
        n905 = Index Array(array=w397) -> (element=w398:T29)  [unwired: 1 in]
        n906 = Index Array(array=w397) -> (element=w408:T29)  [unwired: 1 in]
        n907 = Unbundle(w398) -> ("Position"=w406:cluster{"X":sgl, "Y":sgl}, "Radius"=w399:dbl)  [unwired: 1 out]
        n908 = Unbundle(w408) -> ("Position"=w407:cluster{"X":sgl, "Y":sgl})  [unwired: 2 out]
        n909 = Unbundle(w406) -> ("X"=w404:sgl, "Y"=w405:sgl)
        n910 = Unbundle(w407) -> ("X"=→"Bubble x 2":sgl, "Y"=→"Bubble y 2":sgl)
        n911 = Subtract(x=w404, y=w399) -> (x-y=→"toplx 3":dbl)
        n912 = Add(x=w404, y=w399) -> (x+y=→"bottomrx 3":dbl)
        n913 = Add(x=w405, y=w399) -> (x+y=→"bottomry 3":dbl)
        n914 = Subtract(x=w405, y=w399) -> (x-y=→"toply 3":dbl)
      }
    }
    n915 = local read "Stop"() -> (w93:i32)
    n916 = local read "Start"() -> (w92:i32)
    n917 = Subtract(x=w93, y=w92) -> (x-y=→"Time Elapsed(ms)":i32)
    n918 = case shown="True" "Play" {
      frame False {
      }
      frame True {
        n919 = stacked-sequence {
          frame #0 {
            n920 = Tick Count (ms)() -> (millisecond timer value=→"Start":u32)
          }
          frame #1 {
            n921 = local read "ROI switch"() -> (w542:bool)
            n922 = case shown="True" w542 {
              frame True {
                # "When this is on select a new Midpoint using the ROI tool"
                n923 = case shown="False" "New location\n ROI" {
                  frame False {
                    n924 = local read "ROI Point 2"() -> (w553:T7)
                    n925 = local read "ROI Point 1"() -> (w554:T7)
                    n926 = local read "ROI Point 3"() -> (w552:T7)
                    n927 = local read "ROI Point 4"() -> (w551:T7)
                    n928 = local read "ROI point 5"() -> (w550:T7)
                    n929 = local read "ROI Point 6"() -> (w549:T7)
                    n930 = Build Array (concatenate) ("Build Matrix")(w554, w553, w552, w551, w550, w549) -> (w555:T7)
                    n931 = local write "NewXYArray"(w555) -> ()
                  }
                  frame True {
                    w592 = 1e-07
                    n932 = local read "Radius ROI x1"() -> (w594:dbl)
                    n933 = local read "Radius ROI x3"() -> (w575:dbl)
                    n934 = local read "Radius ROI x4"() -> (w573:dbl)
                    n935 = local read "Radius ROI y1"() -> (w593:dbl)
                    n936 = local read "Radius ROI y2"() -> (w576:dbl)
                    n937 = local read "Radius ROI y3"() -> (w574:dbl)
                    n938 = local read "Radius ROI y4"() -> (w572:dbl)
                    n939 = local read "Radius ROI y5"() -> (w570:dbl)
                    n940 = local read "Radius ROI y6"() -> (w568:dbl)
                    n941 = local read "Radius ROI x2"() -> (w577:dbl)
                    n942 = local read "Radius ROI x5"() -> (w571:dbl)
                    n943 = local read "Radius ROI x6"() -> (w569:dbl)
                    n944 = local read "ROI new MPx"() -> (w579:dbl)
                    n945 = local read "ROI new Mpy"() -> (w578:dbl)
                    n946 = Add(x=w594, y=w579) -> (x+y=w567:dbl)
                    n947 = Add(x=w593, y=w578) -> (x+y=w566:dbl)
                    n948 = Add(x=w579, y=w577) -> (x+y=w565:dbl)
                    n949 = Add(x=w578, y=w576) -> (x+y=w564:dbl)
                    n950 = Add(x=w579, y=w575) -> (x+y=w563:dbl)
                    n951 = Add(x=w578, y=w574) -> (x+y=w562:dbl)
                    n952 = Add(x=w579, y=w573) -> (x+y=w561:dbl)
                    n953 = Add(x=w578, y=w572) -> (x+y=w560:dbl)
                    n954 = Add(x=w579, y=w571) -> (x+y=w559:dbl)
                    n955 = Add(x=w570, y=w578) -> (x+y=w558:dbl)
                    n956 = Add(x=w579, y=w569) -> (x+y=w557:dbl)
                    n957 = Add(x=w568, y=w578) -> (x+y=w556:dbl)
                    n958 = Build Array(w567, w566) -> (w591:T7)
                    n959 = Build Array(w565, w564) -> (w588:T7)
                    n960 = Build Array(w563, w562) -> (w587:T7)
                    n961 = Build Array(w561, w560) -> (w586:T7)
                    n962 = Build Array(w559, w558) -> (w585:T7)
                    n963 = Build Array(w557, w556) -> (w584:T7)
                    n964 = call-poly <vilib>:"Multiply.vi"("Real Scalar c"=w592, "Real Matrix A"=w591) -> ("A * c"=w590:T7)
                    n965 = call-poly <vilib>:"Multiply.vi"("Real Scalar c"=w592, "Real Matrix A"=w588) -> ("A * c"=w589:T7)
                    n966 = call-poly <vilib>:"Multiply.vi"("Real Scalar c"=w592, "Real Matrix A"=w587) -> ("A * c"=w583:T7)
                    n967 = call-poly <vilib>:"Multiply.vi"("Real Scalar c"=w592, "Real Matrix A"=w586) -> ("A * c"=w582:T7)
                    n968 = call-poly <vilib>:"Multiply.vi"("Real Scalar c"=w592, "Real Matrix A"=w585) -> ("A * c"=w581:T7)
                    n969 = call-poly <vilib>:"Multiply.vi"("Real Scalar c"=w592, "Real Matrix A"=w584) -> ("A * c"=w580:T7)
                    n970 = Build Array (concatenate) ("Build Matrix")(w590, w589, w583, w582, w581, w580) -> (w595:T7)
                    n971 = local write "NewXYArray"(w595) -> ()
                  }
                }
              }
              frame False {
                n972 = case shown="True" "Input New \nObject Location" {
                  frame True {
                    n973 = local read "Caging Radius"() -> (w599:dbl)
                    n974 = Multiply(x=w599, y=1e-07) -> (x*y=w597:dbl)
                    n975 = local read "Radius"() -> (w601:dbl)
                    n976 = local read "New Center X"() -> (w613:dbl)
                    n977 = Add(x=w601, y=w597) -> (x+y=w600:dbl)
                    n978 = Add(x=w613, y=w600) -> (x+y=w619:dbl)
                    n979 = local read "New Center Y"() -> (w617:dbl)
                    n980 = local read "# of pairs"() -> (w616:dbl)
                    n981 = Multiply(x=w619, y=1e-07) -> (x*y=w612:dbl)
                    n982 = Multiply(x=w616, y=2.0) -> (x*y=w614:dbl)
                    n983 = Multiply(x=w617, y=1e-07) -> (x*y=w611:dbl)
                    n984 = Initialize Array(w612, w614) -> (w610:dbl[])
                    n985 = local read "Delta y"() -> (w608:dbl[])
                    n986 = local read "Delta x"() -> (w609:dbl[])
                    n987 = Initialize Array(w611, w614) -> (w607:dbl[])
                    n988 = for {
                      tunnel: w608 -> [w628] mode=indexing
                      tunnel: w607 -> [w627] mode=indexing
                      tunnel: [w626] -> w604 mode=indexing
                      n989 = Add(x=w627, y=w628) -> (x+y=w626:dbl)
                    }
                    n990 = for {
                      tunnel: w610 -> [w625] mode=indexing
                      tunnel: w609 -> [w624] mode=indexing
                      tunnel: [w623] -> w606 mode=indexing
                      n991 = Subtract(x=w625, y=w624) -> (x-y=w623:dbl)
                    }
                    n992 = for {
                      tunnel: w607 -> [w631] mode=indexing
                      tunnel: w608 -> [w630] mode=indexing
                      tunnel: [w629] -> w605 mode=indexing
                      n993 = Subtract(x=w631, y=w630) -> (x-y=w629:dbl)
                    }
                    n994 = Build Array(w606, w604) -> (w603:T7)
                    n995 = Build Array(w606, w605) -> (w602:T7)
                    n996 = Build Array(w612, w611) -> (w622:T7)
                    n997 = Build Array (concatenate)(w622, w603, w602) -> (w621:T7)
                    n998 = local write "NewXYArray"(w621) -> ()
                  }
                  frame False {
                    # "array of bubbles"
                    n999 = local read "Max Number \nof Bubbles"() -> (w638:dbl)
                    n1000 = local read "bottomry 2"() -> (w663:dbl)
                    n1001 = local read "toply 2"() -> (w664:dbl)
                    n1002 = Subtract(x=w664, y=w663) -> (x-y=w666:dbl)
                    n1003 = local read "Caging Radius"() -> (w639:dbl)
                    n1004 = local read "bottomrx 2"() -> (w656:dbl)
                    n1005 = local read "bottomry 2"() -> (w655:dbl)
                    n1006 = case shown="Default" w638 {
                      tunnel: [1 2 3 4 5 6 0] -> w644
                      frame 3 {
                      }
                      frame 4, 5 {
                      }
                      frame 6, 7 {
                      }
                      frame 8, 9 {
                      }
                      frame 10, 11 {
                      }
                      frame 12 {
                      }
                      frame Default {
                      }
                    }
                    "# of pairs" <- w644
                    n1007 = local read "Radius"() -> (w647:dbl)
                    n1008 = Divide(x=w666, y=2.0) -> (x/y=w654:dbl)
                    n1009 = Add(x=w655, y=w654) -> (x+y=w657:dbl)
                    n1010 = Multiply(x=w656, y=1e-07) -> (x*y=w642:dbl)
                    n1011 = Multiply(x=w647, y=1e-07) -> (x*y=w633:dbl)
                    n1012 = Multiply(x=w639, y=1e-07) -> (x*y=w637:dbl)
                    n1013 = Multiply(x=w657, y=1e-07) -> (x*y=w653:dbl)
                    n1014 = Add(x=w633, y=w637) -> (x+y=w643:dbl)
                    n1015 = Add(x=w637, y=w642) -> (x+y=w641:dbl)
                    n1016 = for {
                      N: w644 -> [_]
                      tunnel: w638 -> [w684]
                      tunnel: w643 -> [w683]
                      tunnel: w653 -> [w682]
                      tunnel: [w681] -> w652 mode=indexing
                      tunnel: [w680] -> w651 mode=indexing
                      tunnel: [w679] -> w650 mode=indexing
                      tunnel: [w677] -> w646 mode=indexing
                      tunnel: [w676] -> w645 mode=indexing
                      tunnel: w641 -> [w675]
                      tunnel: [w674] -> w636 mode=indexing
                      i -> [w678]
                      w693 = 2.0
                      n1017 = Divide(x=360, y=w684) -> (x/y=w699:dbl)
                      n1018 = Add(x=1, y=w678) -> (x+y=w697:i32)
                      n1019 = Multiply(x=w699, y=w697) -> (x*y=w692:dbl)
                      n1020 = expression code="(x/180.0)*pi" ("degrees to radians")(w692) -> (w691:dbl)
                      n1021 = Subtract(x=180, y=w692) -> (x-y=w700:dbl)
                      n1022 = Square(x=w683) -> (x^2=w695:dbl)
                      n1023 = Cosine(x=w691) -> (cos(x)=w690:dbl)
                      n1024 = Divide(x=w700, y=w693) -> (x/y=w688:dbl)
                      n1025 = Multiply(x=w693, y=w695) -> (x*y=w696:dbl)
                      n1026 = Compound Arithmetic op=MULTIPLY(w693, w690, w695) -> (w694:dbl)
                      n1027 = expression code="(x/180.0)*pi" ("degrees to radians")(w688) -> (w689:dbl)
                      n1028 = Subtract(x=w696, y=w694) -> (x-y=w686:dbl)
                      n1029 = Sine(x=w689) -> (sin(x)=w685:dbl)
                      n1030 = Cosine(x=w689) -> (cos(x)=w687:dbl)
                      n1031 = Square Root(x=w686) -> (sqrt(x)=w674:dbl)
                      n1032 = Multiply(x=w685, y=w674) -> (x*y=w677:dbl)
                      n1033 = Multiply(x=w687, y=w674) -> (x*y=w676:dbl)
                      n1034 = Add(x=w682, y=w677) -> (x+y=w680:dbl)
                      n1035 = Subtract(x=w682, y=w677) -> (x-y=w681:dbl)
                      n1036 = Subtract(x=w675, y=w676) -> (x-y=w679:dbl)
                    }
                    "Delta y" <- w646
                    "Delta x" <- w645
                    n1037 = Index Array(array=w636, index=0) -> (element=w634:dbl)
                    n1038 = Build Array(w650, w651) -> (w660:T7)
                    n1039 = Greater Or Equal?(x=w634, y=w633) -> (x >= y?=→"Caging Radius \nToo Big":bool)
                    n1040 = Build Array(w641, w653) -> (w661:T7)
                    n1041 = Build Array(w650, w652) -> (w659:T7)
                    n1042 = Build Array (concatenate) ("Build Matrix")(w661, w660, w659) -> (→"NewXYArray":T7)
                  }
                }
              }
            }
            n1043 = local write "Max Number \nof Bubbles"("Max Number \nof Bubbles") -> ()
            n1044 = local write "LCS"("LCS") -> ()
            n1045 = local write "Rates"("Rates") -> ()
            n1046 = local write "How Many Frames?"("Number of Planned\nSequence Frames") -> ()
            "Initiate Creation" <- 1.0
          }
          frame #2 {
            n1047 = local read "NewXYArray"() -> (w706:dbl[][])
            n1048 = Array Size(array=w706) -> (size(s)=w705:i32[])
            n1049 = Index Array(array=w705, index=0) -> (element=w703:i32)
            "NewXYArraySize" <- w703
            n1050 = for {
              N: w703 -> [w708]
              i -> [w709]
              stop <- w707 stop-if-true
              n1051 = stacked-sequence {
                tunnel: w709 -> [w711 _]
                tunnel: w708 -> [w710 _]
                tunnel: [_ w714] -> w707
                frame #0 {
                  n1052 = local write "Locked Current Spot"(w711) -> ()
                  n1053 = local write "# of Spots"(w710) -> ()
                  n1054 = local write "Rates"(1) -> ()
                  n1055 = local write "LCS"(0) -> ()
                }
                frame #1 {
                  n1056 = local read "Insert"() -> (w714:bool)
                  n1057 = local write "Insert"(TRUE) -> ()
                }
              }
            }
          }
        }
      }
    }
    n1058 = local read "toplx 2"() -> (w77:dbl)
    n1059 = local read "bottomrx 2"() -> (w78:dbl)
    n1060 = local write "Caging Radius"("Caging Radius") -> ()
    n1061 = Subtract(x=w77, y=w78) -> (x-y=w80:dbl)
    n1062 = local read "toplx 2"() -> (w82:dbl)
    n1063 = Absolute Value(x=w80) -> (abs(x)=w81:dbl)
    n1064 = Divide(x=w81, y=2.0) -> (x/y=w69:dbl)
    n1065 = Add(x=w69, y=w82) -> (x+y=→"Center X":dbl)
    n1066 = local write "New Center X"("New Center X") -> ()
    n1067 = local read "bottomry 2"() -> (w76:dbl)
    n1068 = local read "toply 2"() -> (w75:dbl)
    n1069 = Subtract(x=w76, y=w75) -> (x-y=w74:dbl)
    n1070 = local write "New Center Y"("New Center Y") -> ()
    n1071 = Absolute Value(x=w74) -> (abs(x)=w73:dbl)
    n1072 = local read "toply 2"() -> (w71:dbl)
    n1073 = Divide(x=w73, y=2.0) -> (x/y=w68:dbl)
    n1074 = Add(x=w68, y=w71) -> (x+y=→"Center Y":dbl)
    n1075 = case shown="True" "Lock Current Spot" {
      frame False {
      }
      frame True {
        n1076 = global read "red_tweezers_globals.vi" "Spots"() -> (w793:T3[])
        n1077 = local read "Current Spot #"() -> (w794:dbl)
        "Locked Current Spot" <- w794
        n1078 = Index Array(array=w793, index=w794) -> (element=w795:T3)
        n1079 = Unbundle By Name(w795) -> ("Position.x"=→"LCS X":dbl, "Position.y"=→"LCS Y":dbl)
        n1080 = local write "LCS"(0) -> ()
      }
    }
    n1081 = local read "Rates"() -> (w98:dbl)
    n1082 = Equal?(x=w98, y=1.0) -> (x = y?=w96:bool)
    n1083 = case shown="True" w96 {
      frame False {
      }
      frame True {
        n1084 = stacked-sequence {
          frame #0 {
            n1085 = local read "Number of Planned\nSequence Frames"() -> (w490:dbl)
            n1086 = local read "Tab Control"() -> (w491:enum32{"Line", "Arc"})
            n1087 = case shown="\"Line\"" w491 {
              tunnel: w490 -> [w492 w511]
              frame "Arc" {
                n1088 = stacked-sequence {
                  tunnel: w492 -> [_ w505 _]
                  frame #0 {
                    n1089 = expression code="(x/180.0)*pi" "degrees to radians"("Theta") -> (→"Radians":dbl)
                    n1090 = local read "Radians"() -> (w504:dbl)
                    n1091 = local read "Original Y"() -> (w498:dbl)
                    n1092 = local read "Original X"() -> (w496:dbl)
                    n1093 = Cosine(x=w504) -> (cos(x)=w493:dbl)
                    n1094 = Sine(x=w504) -> (sin(x)=w495:dbl)
                    n1095 = Multiply(x=w493, y="Radius X") -> (x*y=w497:dbl)
                    n1096 = Multiply(x="Radius X", y=w495) -> (x*y=w499:dbl)
                    n1097 = Subtract(x=w496, y=w497) -> (x-y=→"Center X":dbl)
                    n1098 = Subtract(x=w498, y=w499) -> (x-y=→"Center Y":dbl)
                  }
                  frame #1 {
                    n1099 = local read "Radians"() -> (w509:dbl)
                    n1100 = Subtract(x=w505, y=1) -> (x-y=w507:dbl)
                    n1101 = Divide(x=w509, y=w507) -> (x/y=→"Degree Rate":dbl)
                  }
                  frame #2 {
                  }
                }
              }
              frame "Line" {
                n1102 = local read "Max Number \nof Bubbles"() -> (w510:dbl)
                n1103 = for {
                  N: w510 -> [_]
                  tunnel: w511 -> [w513]
                  i -> [w512]
                  n1104 = stacked-sequence {
                    tunnel: w513 -> [_ w531]
                    tunnel: w512 -> [w517 w528]
                    frame #0 {
                      n1105 = local read "NewXYArray"() -> (w523:dbl[][])
                      n1106 = Index Array(array=w523, index (row)=w517) -> (element=w522:dbl[])  [unwired: 1 in]
                      n1107 = Array To Cluster(array=w522) -> (cluster=w521:T33)
                      n1108 = global read "red_tweezers_globals.vi" "Spots"() -> (w518:T3[])
                      n1109 = Unbundle By Name(w521) -> ("NewXYArray[0]"=w520:dbl, "NewXYArray[1]"=w519:dbl)
                      n1110 = Index Array(array=w518, index=w517) -> (element=w516:T3)
                      n1111 = local write "New Y"(w519) -> ()
                      n1112 = local write "New X"(w520) -> ()
                      n1113 = Unbundle By Name(w516) -> ("Position.x"=w515:dbl, "Position.y"=w514:dbl)
                      n1114 = local write "Original X"(w515) -> ()
                      n1115 = local write "Original Y"(w514) -> ()
                    }
                    frame #1 {
                      n1116 = local read "Original X"() -> (w532:dbl)
                      n1117 = local read "Original Y"() -> (w534:dbl)
                      n1118 = Subtract(x=w531, y=1) -> (x-y=w538:dbl)
                      n1119 = local read "New Y"() -> (w535:dbl)
                      n1120 = local read "New X"() -> (w533:dbl)
                      n1121 = Subtract(x=w534, y=w535) -> (x-y=w537:dbl)
                      n1122 = Subtract(x=w532, y=w533) -> (x-y=w536:dbl)
                      n1123 = Divide(x=w537, y=w538) -> (x/y=w526:dbl)
                      "Y Rate" <- w526
                      n1124 = Divide(x=w536, y=w538) -> (x/y=w527:dbl)
                      "X Rate" <- w527
                      n1125 = Bundle(w527, w526) -> (w525:cluster{dbl, dbl})  [unwired: 1 in]
                      n1126 = local read "NewXYRates"() -> (w529:dbl[][])
                      n1127 = Cluster To Array(cluster=w525) -> (array=w524:dbl[])
                      n1128 = Insert Into Array(array=w529, index (row)=w528, new element=w524) -> (w530:dbl[][])  [unwired: 1 in]
                      n1129 = local write "NewXYRates"(w530) -> ()
                    }
                  }
                }
              }
            }
          }
          frame #1 {
            n1130 = local write "Rates"(0) -> ()
          }
        }
      }
    }
    n1131 = case shown="True" "Mark Original Position" {
      frame False {
      }
      frame True {
        w796 = TRUE
        n1132 = local write "Mark Original Position"(FALSE) -> ()
        n1133 = local read "New X"() -> (→"Original X":dbl)
        n1134 = local read "New Y"() -> (→"Original Y":dbl)
        "MOP pressed After" <- w796
        "MOP pressed" <- w796
      }
    }
    n1135 = local read "Sequence Instances"() -> (w154:dbl)
    n1136 = case shown="True" w173 {
      tunnel: w179 -> [_ w862]
      frame False {
      }
      frame True {
        n1137 = global write "red_tweezers_globals_INTERNAL.vi" "Image Overlay (extras from control loop)"(w862) -> ()
      }
    }
    n1138 = local read "Counter"() -> (w153:dbl)
    n1139 = call "red_tweezers_UNDO.vi"("Force Save"=w175, "This change is inconsequential (don't save it)"=w176, "Selection/Group"=w177, "Spots"=w178) -> ()  [unwired: 6 in, 2 out]
    n1140 = call "sync_with_globals.vi"("Selection/Group"=w177, "Spots"=w178) -> ("Selection/Group 2"=w189:T12[], "Spots 2"=w140:T3[])  [unwired: 4 in]
    n1141 = local read "Sequence Storer"() -> (w149:T3[][])
    n1142 = local read "Sequence On?"() -> (w152:bool)
    n1143 = local read "Sequence On?"() -> (w167:bool)
    n1144 = call "SequenceControl.vi"("Sequence On? 2"=w152, "Counter 2"=w153, "Sequence Instances 2"=w154, "Sequence Storer"=w149) -> ("Time per Frame (ms) 2"=w147:dbl, "Sequence Order 2"=w150:dbl, "Reset 2"=w151:bool, "Sequence Storer 2"=w162:T3[][], "Clearance Button 2"=w161:bool, "Manual Edit 2"=w160:bool, "Save State 2"=w159:bool, "Play Sequence 2"=w156:bool, "Bubble ID to Empty 2"=w155:dbl, "Manual Sequence 2"=w157:bool, "Edit Sequence Mode 2"=w158:bool)  [unwired: 1 in]
    n1145 = local write "Play Sequence"(w156) -> ()
    n1146 = local write "Bubble ID to Empty"(w155) -> ()
    n1147 = local write "Manual Sequence"(w157) -> ()
    n1148 = local write "Reset"(w151) -> ()
    n1149 = local write "Edit Sequence Mode"(w158) -> ()
    n1150 = local write "Clearance Button"(w161) -> ()
    n1151 = local write "Sequence Storer"(w162) -> ()
    n1152 = local write "Save State"(w159) -> ()
    n1153 = local write "Manual Edit"(w160) -> ()
    n1154 = Or(x=w167, y="Manual Sequence") -> (x .or. y?=w166:bool)
    n1155 = local write "Time per Frame (ms)"(w147) -> ()
    n1156 = feedback #10() -> (w194:T34)  [unwired: 1 out]
    n1157 = call "Smoothed Frame Rate.vi"("Feedback In"=w194) -> ("Feedback Out"=w193:T34, "Frame Rate"=→"Interface Frame Rate":dbl)  [unwired: 1 in, 4 out]
    n1158 = feedback-in #10(w193) -> ()
    n1159 = local write "Sequence Order"(w150) -> ()
    n1160 = Not(x=w143) -> (.not. x?=w144:bool)
    n1161 = Not(x="Output to SLM") -> (.not. x?=w145:bool)
    n1162 = case shown="True" w166 {
      tunnel: [w832 w837] -> w170
      tunnel: w140 -> [w831 _]
      frame False {
        n1163 = Or(x="Manual Edit", y="Edit Sequence Mode") -> (x .or. y?=w830:bool)
        n1164 = case shown="False" w830 {
          tunnel: w831 -> [w833 _]
          tunnel: [w833 w834] -> w832
          frame False {
          }
          frame True {
            n1165 = local read "Sequence Order"() -> (w835:dbl)
            n1166 = local read "Sequence Storer"() -> (w836:T3[][])
            n1167 = Index Array(array=w836, index (row)=w835) -> (element=w834:T3[])  [unwired: 1 in]
          }
        }
      }
      frame True {
        n1168 = stacked-sequence {
          tunnel: [w839 _] -> w837
          frame #0 {
            n1169 = local read "Counter"() -> (w840:dbl)
            n1170 = local read "Sequence Storer"() -> (w841:T3[][])
            n1171 = Index Array(array=w841, index (row)=w840) -> (element=w839:T3[])  [unwired: 1 in]
            n1172 = Wait (ms)(milliseconds to wait="Time per Frame (ms)") -> ()  [unwired: 1 out]
          }
          frame #1 {
            n1173 = local read "Sequence Instances"() -> (w843:dbl)
            n1174 = local read "Counter"() -> (w846:dbl)
            n1175 = Subtract(x=w843, y=1) -> (x-y=w844:dbl)
            n1176 = Equal?(x=w846, y=w844) -> (x = y?=w845:bool)
            n1177 = case shown="True" w845 {
              frame False {
                n1178 = local read "Counter"() -> (w849:dbl)
                n1179 = Add(x=w849, y=1) -> (x+y=→"Counter":dbl)
              }
              frame True {
                w850 = FALSE
                n1180 = local write "Counter"(0) -> ()
                n1181 = local write "Play Sequence"(w850) -> ()
                n1182 = local write "Sequence On?"(w850) -> ()
              }
            }
          }
        }
      }
    }
    n1183 = case shown="True" "Save State" {
      tunnel: w140 -> [_ w853]
      frame False {
      }
      frame True {
        n1184 = local write "Save State"(FALSE) -> ()
        n1185 = stacked-sequence {
          tunnel: w853 -> [w854 _]
          frame #0 {
            "Spot Storage" <- w854
          }
          frame #1 {
            n1186 = local read "Spot Storage"() -> (w860:T3[])
            n1187 = Replace Array Subset(array="Sequence Storer", new element=w860, index (row)="Sequence Order") -> (w858:T3[][])  [unwired: 1 in]
            n1188 = Array Size(array=w858) -> (size(s)=w857:i32[])
            n1189 = local write "Sequence Storer"(w858) -> ()
            n1190 = Index Array(array=w857, index=0) -> (element=→"Sequence Instances":i32)
          }
        }
      }
    }
    n1191 = case shown="True" "Clearance Button" {
      frame False {
      }
      frame True {
        # "This is the Bubble ID to Empty tool- this \"deletes\" the bubble in a sequence."
        n1192 = local read "Sequence Order"() -> (w823:dbl)
        n1193 = local read "Sequence Storer"() -> (w824:T3[][])
        n1194 = Replace Array Subset(array=w824, new element=T15 {"Position"={"x"=nan, "y"=nan, "z"=nan}, "Intensity"=1.0, "Vortex Charge"=1, "Phase"=1.0, "NA Position"={"x"=0.0, "y"=0.0, "r"=1.0}, "Line Trapping"={"Vector"={"x"=0.0, "y"=0.0, "z"=0.0}, "Phase Gradient"=0.0}, "Amplitude Correction"=0.0} ("Cluster"), index (row)=w823, index (col)="Bubble ID to Empty") -> (w820:T3[][])
        n1195 = local write "Sequence Storer"(w820) -> ()
      }
    }
    n1196 = case shown="True" "Save" {
      frame False {
      }
      frame True {
        n1197 = local read "Sequence Storer"() -> (w789:T3[][])
        n1198 = call "SequenceSaver.vi"("Sequence Storer"=w789) -> ()  [unwired: 10 in, 1 out]
      }
    }
    n1199 = And(x=w145, y=w144) -> (x .and. y?=w148:bool)
    n1200 = case shown="True" "Load" {
      frame False {
      }
      frame True {
        n1201 = call "SequenceSaver.vi"() -> ("Sequence Storer 2"=w788:T3[][])  [unwired: 11 in]
        n1202 = local write "Sequence Storer"(w788) -> ()
      }
    }
    n1203 = local read "Initiate Creation"() -> (w101:dbl)
    n1204 = case shown="True" w148 {
      tunnel: w140 -> [w2250 _]
      frame False {
        n1205 = call "UDP Sender generic_2.vi"("Spots"=w2250) -> ()  [unwired: 2 in, 1 out]
      }
      frame True {
      }
    }
    n1206 = case shown="True" "Reset" {
      frame False {
      }
      frame True {
        n1207 = local write "Counter"(0) -> ()
      }
    }
    n1208 = case shown="True" "Add Additional Frames" {
      frame False {
      }
      frame True {
        # "This adds additional frames to the sequence."
        n1209 = for {
          N: "Additional Frames Wanted" -> [_]
          i -> [w802]
          n1210 = local read "Max Number \nof Bubbles"() -> (w806:dbl)
          n1211 = Add(x=1, y=w802) -> (x+y=w803:i32)
          n1212 = Add(x="Frame Location", y=w803) -> (x+y=w804:dbl)
          n1213 = Initialize Array(T15 {"Position"={"x"=nan, "y"=nan, "z"=nan}, "Intensity"=1.0, "Vortex Charge"=1, "Phase"=1.0, "NA Position"={"x"=0.0, "y"=0.0, "r"=1.0}, "Line Trapping"={"Vector"={"x"=0.0, "y"=0.0, "z"=0.0}, "Phase Gradient"=0.0}, "Amplitude Correction"=0.0} ("Cluster"), w806) -> (w807:T35)
          n1214 = local read "Sequence Storer"() -> (w808:T3[][])
          n1215 = Insert Into Array(array=w808, index (row)=w804, new element=w807) -> (w809:T3[][])  [unwired: 1 in]
          n1216 = local write "Sequence Storer"(w809) -> ()
        }
      }
    }
    n1217 = case shown="1" w101 {
      frame 0, Default {
      }
      frame 1 {
        # "This create the array needed for a sequential\narray."
        n1218 = local read "Number of Planned\nSequence Frames"() -> (w813:dbl)
        n1219 = local read "Max Number \nof Bubbles"() -> (w812:dbl)
        n1220 = for {
          N: w813 -> [_]
          tunnel: w812 -> [w814]
          i -> [w817]
          n1221 = Initialize Array(T15 {"Position"={"x"=nan, "y"=nan, "z"=nan}, "Intensity"=1.0, "Vortex Charge"=1, "Phase"=1.0, "NA Position"={"x"=0.0, "y"=0.0, "r"=1.0}, "Line Trapping"={"Vector"={"x"=0.0, "y"=0.0, "z"=0.0}, "Phase Gradient"=0.0}, "Amplitude Correction"=0.0} ("Cluster"), w814) -> (w815:T35)
          n1222 = local read "Sequence Storer"() -> (w818:T3[][])
          n1223 = Insert Into Array(array=w818, index (row)=w817, new element=w815) -> (w819:T3[][])  [unwired: 1 in]
          n1224 = local write "Sequence Storer"(w819) -> ()
        }
        n1225 = local write "Initiate Creation"(0) -> ()
      }
    }
    n1226 = case shown="False" "Play Sequence" {
      frame False {
        n1227 = local write "Sequence On?"(FALSE) -> ()
      }
      frame True {
        "Sequence On?" <- TRUE
      }
    }
    n1228 = local read "Current Spot #"() -> (w123:dbl)
    n1229 = local read "Selection/Group"() -> (w124:T12[])
    n1230 = local read "# of Spots"() -> (w139:dbl)
    n1231 = Not Equal?(x=w123, y=-1) -> (x != y?=w125:bool)
    n1232 = local read "spots selected 2"() -> (w113:i32)
    n1233 = Index Array(array=w124, index=w123) -> (element=w122:T12)
    n1234 = Unbundle By Name(w122) -> ("Selected"=w121:bool)
    n1235 = local read "spots selected"() -> (w114:i32)
    n1236 = Not(x=w121) -> (.not. x?=w120:bool)
    n1237 = And(x=w120, y=w125) -> (x .and. y?=w115:bool)
    n1238 = Less?(x=w114, y=w113) -> (x < y?=w111:bool)
    n1239 = case shown="True" "Insert" {
      tunnel: w140 -> [_ w410]
      tunnel: w139 -> [_ w409]
      frame False {
      }
      frame True {
        n1240 = for {
          N: w409 -> [_]
          tunnel: w410 -> [w412]
          i -> [w411]
          n1241 = stacked-sequence {
            tunnel: w412 -> [w414 w419 _]
            tunnel: w411 -> [_ w415 _]
            frame #0 {
              n1242 = local read "Start at Which Frame?"() -> (→"Num":dbl)
              "Spot Storage 2" <- w414
            }
            frame #1 {
              n1243 = local read "Selection/Group"() -> (w418:T12[])
              n1244 = Index Array(array=w418, index=w415) -> (element=w417:T12)
              n1245 = Unbundle By Name(w417) -> ("Selected"=w416:bool)
              n1246 = case shown="True" w416 {
                tunnel: w419 -> [_ _]
                frame False {
                }
                frame True {
                  n1247 = stacked-sequence {
                    frame #0 {
                      n1248 = case shown="\"Arc\"" "Tab Control" {
                        frame "Arc" {
                          n1249 = local read "How Many Frames?"() -> (w423:dbl)
                          n1250 = Subtract(x=w423, y=1) -> (x-y=w421:dbl)
                          n1251 = for {
                            N: w423 -> [_]
                            tunnel: w421 -> [w424]
                            i -> [w426]
                            # "What is this ^\n\nFor # of sequence\nframes, don't worry\nabout it"
                            # "How to make position x and y?\nIt's called a cluster, inser the new position to Position.x and Position.y"
                            n1252 = Equal?(x=w424, y=w426) -> (x = y?=w425:bool)
                            n1253 = case shown="True" w425 {
                              tunnel: [w449 w458] -> w428
                              tunnel: [w448 w457] -> w427
                              tunnel: w426 -> [w445 _]
                              frame False {
                                # "calculating new position"
                                n1254 = local read "Degree Rate"() -> (w447:dbl)
                                n1255 = Multiply(x=w447, y=w445) -> (x*y=w446:dbl)
                                n1256 = Cosine(x=w446) -> (cos(x)=w455:dbl)
                                n1257 = Sine(x=w446) -> (sin(x)=w456:dbl)
                                n1258 = local read "Radius X"() -> (w454:dbl)
                                n1259 = Multiply(x=w454, y=w456) -> (x*y=w453:dbl)
                                n1260 = Multiply(x=w455, y=w454) -> (x*y=w452:dbl)
                                n1261 = local read "Center X"() -> (w451:dbl)
                                n1262 = local read "Center Y"() -> (w450:dbl)
                                n1263 = Add(x=w451, y=w452) -> (x+y=w449:dbl)
                                n1264 = Add(x=w450, y=w453) -> (x+y=w448:dbl)
                              }
                              frame True {
                                n1265 = global read "red_tweezers_globals.vi" "Spots"() -> (w461:T3[])
                                n1266 = local read "Numeric"() -> (w460:dbl)
                                n1267 = Index Array(array=w461, index=w460) -> (element=w459:T3)
                                n1268 = Unbundle By Name(w459) -> ("Position.x"=w458:dbl, "Position.y"=w457:dbl)
                              }
                            }
                            n1269 = local read "Spot Storage 2"() -> (w444:T3[])
                            n1270 = local read "Numeric"() -> (w443:dbl)
                            n1271 = Index Array(array=w444, index=w443) -> (element=w430:T3)
                            n1272 = local read "Start at Which Frame?"() -> (w432:dbl)
                            n1273 = Bundle By Name(cluster=w430, "Position.x"=w428, "Position.y"=w427) -> (w429:T3)
                            n1274 = local read "How Many Frames?"() -> (w431:dbl)
                            n1275 = Subtract(x=w432, y=w426) -> (x-y=w441:dbl)
                            n1276 = local read "Sequence Storer"() -> (w442:T3[][])
                            n1277 = local read "Numeric"() -> (w437:dbl)
                            n1278 = Add(x=w441, y=w431) -> (x+y=w440:dbl)
                            n1279 = Subtract(x=w440, y=1) -> (x-y=w438:dbl)
                            n1280 = Replace Array Subset(array=w442, new element=w429, index (row)=w438, index (col)=w437) -> (w436:T3[][])
                            n1281 = Array Size(array=w436) -> (size(s)=w435:i32[])
                            n1282 = local write "Sequence Storer"(w436) -> ()
                            n1283 = Index Array(array=w435, index=0) -> (element=w433:i32)
                            n1284 = local write "Sequence Instances"(w433) -> ()
                          }
                        }
                        frame "Line" {
                          # "This is the automatic sequence generator which allows for the creation of the sequence. This calculates the LAST coordinates of each bubble first\nbefore going for the first few coordinates of the sequence."
                          n1285 = local read "How Many Frames?"() -> (w462:dbl)
                          n1286 = for {
                            N: w462 -> [_]
                            i -> [w470]
                            # "For why do we multiply?"
                            n1287 = local read "Spot Storage 2"() -> (w480:T3[])
                            n1288 = local read "Numeric"() -> (w467:dbl)
                            n1289 = local read "NewXYRates"() -> (w468:dbl[][])
                            n1290 = Index Array(array=w468, index (row)=w467, index (col)=1) -> (element=w463:dbl)
                            n1291 = Index Array(array=w468, index (row)=w467, index (col)=0) -> (element=w464:dbl)
                            n1292 = Index Array(array=w480, index=w467) -> (element=w478:T3)
                            n1293 = Unbundle By Name(w478) -> ("Position.x"=w485:dbl, "Position.y"=w483:dbl)
                            n1294 = Multiply(x=w464, y=w470) -> (x*y=w484:dbl)
                            n1295 = Multiply(x=w463, y=w470) -> (x*y=w479:dbl)
                            "probe" <- w479
                            n1296 = Subtract(x=w485, y=w484) -> (x-y=w482:dbl)
                            n1297 = Subtract(x=w483, y=w479) -> (x-y=w481:dbl)
                            n1298 = Bundle By Name(cluster=w478, "Position.x"=w482, "Position.y"=w481) -> (w473:T3)
                            n1299 = local read "Sequence Storer"() -> (w486:T3[][])
                            n1300 = local read "Numeric"() -> (w472:dbl)
                            n1301 = Add(x="Start at Which Frame?", y=w470) -> (x+y=w469:dbl)
                            n1302 = Replace Array Subset(array=w486, new element=w473, index (row)=w469, index (col)=w472) -> (w477:T3[][])
                            n1303 = Array Size(array=w477) -> (size(s)=w476:i32[])
                            n1304 = local write "Sequence Storer"(w477) -> ()
                            n1305 = Index Array(array=w476, index=0) -> (element=w474:i32)
                            n1306 = local write "Sequence Instances"(w474) -> ()
                          }
                        }
                      }
                    }
                    frame #1 {
                      w488 = FALSE
                      n1307 = Tick Count (ms)() -> (millisecond timer value=→"Stop":u32)
                      n1308 = local write "Play Pressed"(w488) -> ()
                      "Insert End" <- w488
                    }
                  }
                }
              }
              "Numeric" <- w415
            }
            frame #2 {
              n1309 = local write "Insert"(FALSE) -> ()
            }
          }
        }
      }
    }
    n1310 = And(x=w111, y=w115) -> (x .and. y?=w116:bool)
    n1311 = local read "Position"() -> (w54:cluster{"x":dbl, "y":dbl, "z":dbl})
    n1312 = case shown="True" w116 {
      frame False {
      }
      frame True {
        n1313 = local read "# of Spots"() -> (w723:dbl)
        n1314 = for {
          N: w723 -> [_]
          i -> [w725]
          stop <- w724 stop-if-true
          n1315 = local read "Selection/Group"() -> (w727:T12[])
          n1316 = Index Array(array=w727, index=w725) -> (element=w726:T12)
          n1317 = Unbundle By Name(w726) -> ("Selected"=w724:bool)
          n1318 = case shown="True" w724 {
            tunnel: w725 -> [_ w729]
            frame False {
            }
            frame True {
              n1319 = local write "Current Spot #"(w729) -> ()
              "Induce check" <- TRUE
            }
          }
        }
      }
    }
    n1320 = local read "spots selected"() -> (w126:i32)
    n1321 = local read "spots selected 2"() -> (w127:i32)
    n1322 = local read "Prev Current Spot"() -> (w135:dbl)
    n1323 = local read "1spot X"() -> (w50:dbl)
    n1324 = local read "2spot X"() -> (w43:dbl)
    n1325 = local read "2spot Y"() -> (w45:dbl)
    n1326 = local read "1spot Y"() -> (w48:dbl)
    n1327 = local read "ROI x2"() -> (w44:dbl)
    n1328 = local read "ROI y2"() -> (w46:dbl)
    n1329 = local read "ROI x1"() -> (w51:dbl)
    n1330 = local read "Number of Planned\nSequence Frames"() -> (w39:dbl)
    n1331 = local read "ROI y1"() -> (w49:dbl)
    n1332 = local read "Number of Planned\nSequence Frames"() -> (w40:dbl)
    n1333 = local read "Current Spot #"() -> (w136:dbl)
    n1334 = Unbundle(w54) -> ("x"=w53:dbl, "y"=w52:dbl)  [unwired: 1 out]
    n1335 = case shown="3" "Spots" {
      tunnel: w53 -> [_ w274 w276 w278]
      tunnel: w52 -> [_ w273 w275 w277]
      frame 0, Default {
      }
      frame 1 {
        "1spot X" <- w274
        "1spot Y" <- w273
      }
      frame 2 {
        "2spot X" <- w276
        "2spot Y" <- w275
      }
      frame 3 {
        "3spot X" <- w278
        "3spot Y" <- w277
      }
    }
    n1336 = Not Equal?(x=w136, y=w135) -> (x != y?=w134:bool)
    n1337 = Greater?(x=w127, y=w126) -> (0:w128:bool)
    n1338 = Subtract(x=w44, y=w43) -> (x-y=w42:dbl)
    n1339 = Subtract(x=w46, y=w45) -> (x-y=w41:dbl)
    n1340 = Subtract(x=w51, y=w50) -> (x-y=w38:dbl)
    n1341 = Subtract(x=w49, y=w48) -> (x-y=w47:dbl)
    n1342 = local read "Induce check"() -> (w117:bool)
    n1343 = Or(x=w134, y=w128) -> (x .or. y?=w119:bool)
    n1344 = Or(x=w119, y=w117) -> (x .or. y?=w118:bool)
    n1345 = Divide(x=w42, y=w40) -> (x/y=w36:dbl)
    "Step Calculation X2" <- w36
    n1346 = Divide(x=w41, y=w40) -> (x/y=w35:dbl)
    "Step Calculation Y2" <- w35
    n1347 = Divide(x=w38, y=w39) -> (x/y=w37:dbl)
    "Step Calculation X1" <- w37
    n1348 = Divide(x=w47, y=w39) -> (x/y=w34:dbl)
    "Step Calculation Y1" <- w34
    n1349 = case shown="True" w118 {
      frame False {
      }
      frame True {
        n1350 = stacked-sequence {
          frame #0 {
            # "A small 100 ms delay is given to provide enough time for the data to be processed properly."
            n1351 = local read "Null array"() -> (w735:dbl[])
            n1352 = local write "What to Check"(w735) -> ()
            n1353 = local write "ID"(w735) -> ()
            n1354 = local read "Current Spot #"() -> (w737:dbl)
            n1355 = local write "Potential Collisions"(0) -> ()
            n1356 = local read "Spot Checker"() -> (w736:T3[])
            n1357 = Index Array(array=w736, index=w737) -> (element=w738:T3)
            n1358 = Wait (ms)(milliseconds to wait=10) -> ()  [unwired: 1 out]
            n1359 = Unbundle By Name(w738) -> ("Position.x"=w732:dbl, "Position.y"=w733:dbl)
            n1360 = local write "Orig Y SC"(w733) -> ()
            n1361 = local write "Orig X SC"(w732) -> ()
            n1362 = local write "Induce check"(FALSE) -> ()
          }
          frame #1 {
            n1363 = local read "# of Spots"() -> (w739:dbl)
            n1364 = for {
              N: w739 -> [_]
              tunnel: w739 -> [w744]
              i -> [w740]
              n1365 = local read "Selection/Group"() -> (w743:T12[])
              n1366 = Index Array(array=w743, index=w740) -> (element=w742:T12)
              n1367 = Unbundle By Name(w742) -> ("Selected"=w741:bool)
              n1368 = case shown="True" w741 {
                tunnel: w744 -> [_ w746]
                tunnel: w740 -> [_ w745]
                frame False {
                }
                frame True {
                  n1369 = for {
                    N: w746 -> [_]
                    tunnel: w745 -> [w747]
                    i -> [w748]
                    # "If the bubble is not selected, find difference of bubble to bubble\nbeing checked"
                    n1370 = local read "Selection/Group"() -> (w752:T12[])
                    n1371 = Index Array(array=w752, index=w748) -> (element=w751:T12)
                    n1372 = Unbundle By Name(w751) -> ("Selected"=w749:bool)
                    n1373 = Not(x=w749) -> (.not. x?=w750:bool)
                    n1374 = case shown="True" w750 {
                      tunnel: w748 -> [_ w756]
                      tunnel: w747 -> [_ w755]
                      tunnel: w747 -> [_ w754]
                      frame False {
                      }
                      frame True {
                        n1375 = local read "Spot Checker"() -> (w773:T3[])
                        n1376 = Index Array(array=w773, index=w756) -> (element=w774:T3)
                        n1377 = Index Array(array=w773, index=w755) -> (element=w772:T3)
                        n1378 = Unbundle By Name(w772) -> ("Position.x"=w769:dbl, "Position.y"=w765:dbl)
                        n1379 = Unbundle By Name(w774) -> ("Position.x"=w766:dbl, "Position.y"=w762:dbl)
                        n1380 = local read "Area+ Buffer"() -> (w753:dbl)
                        n1381 = Subtract(x=w769, y=w753) -> (x-y=w770:dbl)
                        n1382 = Greater Or Equal?(x=w766, y=w770) -> (x >= y?=w771:bool)
                        n1383 = Add(x=w765, y=w753) -> (x+y=w764:dbl)
                        n1384 = Subtract(x=w765, y=w753) -> (x-y=w763:dbl)
                        n1385 = Add(x=w769, y=w753) -> (x+y=w767:dbl)
                        n1386 = Less Or Equal?(x=w762, y=w764) -> (x <= y?=w761:bool)
                        n1387 = Greater Or Equal?(x=w762, y=w763) -> (x >= y?=w760:bool)
                        n1388 = Less Or Equal?(x=w766, y=w767) -> (x <= y?=w768:bool)
                        n1389 = And(x=w771, y=w768) -> (x .and. y?=w758:bool)
                        n1390 = And(x=w761, y=w760) -> (x .and. y?=w759:bool)
                        n1391 = And(x=w758, y=w759) -> (x .and. y?=w757:bool)
                        n1392 = case shown="True" w757 {
                          tunnel: w756 -> [_ _]
                          tunnel: w756 -> [_ w776]
                          tunnel: w754 -> [_ w775]
                          frame False {
                          }
                          frame True {
                            n1393 = stacked-sequence {
                              tunnel: w776 -> [w777 _]
                              tunnel: w775 -> [w778 _]
                              frame #0 {
                                n1394 = local read "Potential Collisions"() -> (w781:dbl)
                                n1395 = local read "What to Check"() -> (w782:dbl[])
                                n1396 = Insert Into Array(array=w782, index=w781, new element=w777) -> (w783:dbl[])
                                n1397 = local read "ID"() -> (w780:dbl[])
                                n1398 = local write "What to Check"(w783) -> ()
                                n1399 = Insert Into Array(array=w780, index=w781, new element=w778) -> (w779:dbl[])
                                n1400 = local write "ID"(w779) -> ()
                              }
                              frame #1 {
                                n1401 = local read "Potential Collisions"() -> (w786:dbl)
                                n1402 = Add(x=w786, y=1) -> (x+y=w784:dbl)
                                n1403 = local write "Potential Collisions"(w784) -> ()
                              }
                            }
                          }
                        }
                      }
                    }
                  }
                }
              }
            }
          }
          frame #2 {
            n1404 = local read "Current Spot #"() -> (w787:dbl)
            n1405 = local write "Prev Current Spot"(w787) -> ()
          }
        }
      }
    }
    n1406 = while {
      tunnel: w47 -> [w248]
      tunnel: w38 -> [w240]
      tunnel: w37 -> [w218]
      tunnel: w34 -> [w238]
      tunnel: w35 -> [w221]
      tunnel: w36 -> [w222]
      tunnel: w42 -> [w225]
      tunnel: w41 -> [w224]
      tunnel: w40 -> [w223]
      i -> [w198]
      stop <- w207 continue-if-true
      # "Distance Formula"
      # "True if distance is less than the distance limit"
      n1407 = Multiply(x=w225, y=-1) -> (x*y=w228:dbl)
      n1408 = Multiply(x=w224, y=-1) -> (x*y=w233:dbl)
      n1409 = Multiply(x=w240, y=-1) -> (x*y=w239:dbl)
      n1410 = Multiply(x=w248, y=-1) -> (x*y=w245:dbl)
      n1411 = Less?(x=w198, y=w223) -> (x < y?=w197:bool)
      n1412 = Less?(x=w228, y=0) -> (x < y?=w231:bool)
      n1413 = Less?(x=w233, y=0) -> (x < y?=w232:bool)
      n1414 = Add(x=1, y=w198) -> (x+y=w220:i32)
      n1415 = Add(x=1, y=w198) -> (x+y=w217:i32)
      n1416 = Multiply(x=w221, y=w220) -> (x*y=w219:dbl)
      n1417 = Multiply(x=w217, y=w218) -> (x*y=w216:dbl)
      n1418 = Multiply(x=w238, y=w217) -> (x*y=w236:dbl)
      n1419 = Multiply(x=w222, y=w220) -> (x*y=w226:dbl)
      n1420 = Less?(x=w239, y=0) -> (x < y?=w243:bool)
      n1421 = Less?(x=w245, y=0) -> (x < y?=w244:bool)
      n1422 = case shown="False" w232 {
        tunnel: w226 -> [w257 w260]
        tunnel: [w255 w258] -> w199
        frame False {
          n1423 = local read "2spot Y"() -> (w256:dbl)
          n1424 = Subtract(x=w256, y=w257) -> (x-y=w255:dbl)
        }
        frame True {
          n1425 = local read "2spot Y"() -> (w259:dbl)
          n1426 = Add(x=w259, y=w260) -> (x+y=w258:dbl)
        }
      }
      n1427 = case shown="False" w231 {
        tunnel: w219 -> [w250 w253]
        tunnel: [w249 w252] -> w214
        frame False {
          n1428 = local read "2spot X"() -> (w251:dbl)
          n1429 = Subtract(x=w251, y=w250) -> (x-y=w249:dbl)
        }
        frame True {
          n1430 = local read "2spot X"() -> (w254:dbl)
          n1431 = Add(x=w253, y=w254) -> (x+y=w252:dbl)
        }
      }
      n1432 = case shown="False" w244 {
        tunnel: w216 -> [w269 w272]
        tunnel: [w267 w270] -> w215
        frame False {
          n1433 = local read "1spot Y"() -> (w268:dbl)
          n1434 = Subtract(x=w268, y=w269) -> (x-y=w267:dbl)
        }
        frame True {
          n1435 = local read "1spot Y"() -> (w271:dbl)
          n1436 = Add(x=w271, y=w272) -> (x+y=w270:dbl)
        }
      }
      n1437 = case shown="False" w243 {
        tunnel: w236 -> [w262 w265]
        tunnel: [w261 w264] -> w213
        frame False {
          n1438 = local read "1spot X"() -> (w263:dbl)
          n1439 = Subtract(x=w263, y=w262) -> (x-y=w261:dbl)
        }
        frame True {
          n1440 = local read "1spot X"() -> (w266:dbl)
          n1441 = Add(x=w265, y=w266) -> (x+y=w264:dbl)
        }
      }
      n1442 = Subtract(x=w199, y=w215) -> (x-y=w211:dbl)
      n1443 = Subtract(x=w214, y=w213) -> (x-y=w212:dbl)
      n1444 = Square(x=w211) -> (x^2=w210:dbl)
      n1445 = Square(x=w212) -> (x^2=w209:dbl)
      n1446 = local read "Bubble Size"() -> (w202:dbl)
      n1447 = local read "Buffer Zone"() -> (w205:dbl)
      n1448 = Add(x=w210, y=w209) -> (x+y=w208:dbl)
      n1449 = Square Root(x=w208) -> (sqrt(x)=w206:dbl)
      n1450 = Multiply(x=w205, y=2) -> (x*y=w203:dbl)
      n1451 = Add(x=w202, y=w203) -> (x+y=w201:dbl)
      n1452 = Greater?(x=w206, y=w201) -> (0:w200:bool)
      n1453 = Not(x=w200) -> (.not. x?=w196:bool)
      n1454 = And(x=w200, y=w197) -> (x .and. y?=w207:bool)
      n1455 = local write "Possible Collision"(w196) -> ()
    }
    n1456 = local read "Buffer Zone"() -> (w132:dbl)
    n1457 = Multiply(x=w132, y=2) -> (x*y=w133:dbl)
    n1458 = Add(x="Area to check", y=w133) -> (x+y=→"Area+ Buffer":dbl)
    n1459 = feedback #11() -> (w105:dbl)  [unwired: 1 in]
    n1460 = Equal?(x=w105, y=10000) -> (x = y?=w106:bool)
    n1461 = call "Elapsed Time"("Reset"=w106) -> ("Elapsed Time (s)"=w104:dbl, "Time has Elapsed"=w109:bool)  [unwired: 11 in, 6 out]
    "Elapsed Time" <- w104
    n1462 = feedback-in #11(w104) -> ()
    n1463 = And(x="On", y=w109) -> (x .and. y?=w110:bool)
    n1464 = case shown="True" w110 {
      frame False {
      }
      frame True {
        n1465 = local read "Position"() -> (w722:cluster{"x":dbl, "y":dbl, "z":dbl})
        n1466 = Unbundle By Name(w722) -> ("x"=→"X Pos every 10 sec":dbl)
      }
    }
    n1467 = case shown="True" "OK Button" {
      frame False {
      }
      frame True {
        n1468 = script code="clear all;\nclc;\n\ng = gigecam('169.254.154.83');\n\ng.PixelFormat= 'BayerGR8'\n\nimg = snapshot(g);\n\nimshow(img);"() -> ()  [unwired: 1 in, 1 out]
      }
    }
    n1469 = case shown="True" "O Button" {
      frame False {
      }
      frame True {
        n1470 = script code="%\n    rslt = Hough1_data(img);\n\n    % Frame translation\n    %- omit this as of now \n    \n    % Control method\n    increment = 10; %assuming the diamiter of the agent around 20 pic \n    \n    %- NewLoc = [x,y] whose unit is px\n    %- update new location based on current location obtained by the camera\n    NewLoc(1)= rslt(1);\n    NewLoc(2)= rslt(2);\n    \n    \n    % Update microrobot location with NewLoc\n    % the single robot would move to oblique downword\n    \n    % wait seconds"() -> ("NewLoc"=w718:dbl[])  [unwired: 1 in, 1 out]
        n1471 = Index Array(array=w718, index=1) -> (element=→"Y":dbl)
        n1472 = Index Array(array=w718, index=0) -> (element=→"X":dbl)
      }
    }
  }
  n1473 = flat-sequence {
    tunnel: w6 -> [w2253]
    tunnel: w5 -> [w2252]
    tunnel: [w2251] -> w3
    frame #0 {
      n1474 = disable-structure shown="\"White Image (stub)\"" {
        disable-tunnel: w2253 -> [_ _ _ _ _ _]
        disable-tunnel: w2252 -> [_ _ w2311 _ _ _]
        disable-tunnel: [_ _ w2310 _ _ _] -> w2251
        frame condition #0 {
          w2255 = u32 10 ("Number of buffers")
          (unwired) FALSE ("background subtraction")
          # "This subdiagram uses the IMAQ drivers, with a pre-allocated ringbuffer for images.  This is the code I use with my Mikrotron MC1362-CL"
          n1475 = call <vilib>:"IMAQ Init.vi"("Interface Name"="img0") -> ("IMAQ Session Out"=w2262:refnum<k11>)  [unwired: 9 in, 1 out]
          n1476 = call <vilib>:"IMAQ Configure List.vi"("Region of interest"="Global ROI (requires restart)", "Number of buffers"=w2255, "Continuous?"=enum16{"One-Shot", "Continuous"}."Continuous", "IMAQ Session In"=w2262) -> ("error out"=w2256:errorcluster, "IMAQ Session Out"=w2258:refnum<k11>)  [unwired: 6 in]
          n1477 = for {
            N: w2255 -> [_]
            tunnel: 0 ("Channel") -> [w2275]
            shift-right: [w2278] -> w2260
            shift-left: w2256 -> [w2274]
            shift-right: [w2277] -> w2259
            shift-left: w2258 -> [w2276]
            i -> [w2273]
            n1478 = Format Into String(format string="mikrotronbuffer%04d", w2273) -> (resulting string=w2271:string)  [unwired: 2 in, 1 out]
            n1479 = call "IMAQ Create"("Image Name"=w2271) -> ("New Image"=w2270:T8)  [unwired: 4 in, 1 out]
            n1480 = call <vilib>:"IMAQ Configure Buffer.vi"("Channel"=w2275, "error in (no error)"=w2274, "Buffer Number"=w2273, "Image In"=w2270, "IMAQ Session In"=w2276) -> ("error out"=w2278:errorcluster, "IMAQ Session Out"=w2277:refnum<k11>)  [unwired: 5 in]
          }
          n1481 = call <vilib>:"IMAQ Start.vi"("error in (no error)"=w2260, "IMAQ Session In"=w2259) -> ("error out"=w2266:errorcluster, "IMAQ Session Out"=w2267:refnum<k11>)  [unwired: 8 in]
          n1482 = call "IMAQ Create"("Image Name"="Red Tweezers live image") -> ("New Image"=w2268:T8)  [unwired: 3 in, 2 out]
          n1483 = while {
            tunnel: w2267 -> [w2286]
            tunnel: w2266 -> [w2285]
            tunnel: w2268 -> [_]
            tunnel: [w2287] -> w2264
            tunnel: [w2280] -> w2265
            i -> [w2282]
            stop <- w2288 stop-if-true
            n1484 = local read "stop"() -> (w2288:bool)
            n1485 = call <vilib>:"IMAQ Extract Buffer.vi"("error in (no error)"=w2285, "Buffer to extract"=w2282, "IMAQ Session In"=w2286) -> ("error out"=w2280:errorcluster, "Image Out"=w2279:T8, "IMAQ Session Out"=w2287:refnum<k11>)  [unwired: 3 in, 3 out]
            n1486 = call "imageQ_camera_hook.vi"("Image"=w2279) -> ()  [unwired: 11 in]
            n1487 = feedback #12() -> (w2283:T34)  [unwired: 1 in]
            n1488 = call "Smoothed Frame Rate.vi"("Feedback In"=w2283) -> ("Feedback Out"=w2284:T34, "Frame Rate"=w2281:dbl)  [unwired: 1 in, 4 out]
            n1489 = feedback-in #12(w2284) -> ()
            n1490 = global write "red_tweezers_globals_INTERNAL_VOLATILE.vi" "Video Frame Rate"(w2281) -> ()
          }
          n1491 = call <vilib>:"IMAQ Close.vi"("error in (no error)"=w2265, "IMAQ Session In"=w2264) -> ()  [unwired: 9 in, 1 out]
        }
        frame condition #1 {
          (unwired) FALSE ("background subtraction")
          # "This subdiagram acquires using the IMAQdx drivers.  This covers most FireWire and GigE cameras (at least the ones supporting the IIDC or GenICam standards)."
          n1492 = call <vilib>:"IMAQdx Open Camera.vi"("Session In"=T11 "dalsaGenie") -> ("error out"=w2291:errorcluster, "Session Out"=w2290:T11)  [unwired: 9 in]
          n1493 = call <vilib>:"IMAQdx Configure Grab.vi"("error in"=w2291, "Session In"=w2290) -> ("error out"=w2292:errorcluster, "Session Out"=w2293:T11)  [unwired: 8 in]
          n1494 = call "IMAQ Create"("Image Name"="Red Tweezers live image") -> ("New Image"=w2296:T8)  [unwired: 3 in, 2 out]
          n1495 = while {
            tunnel: w2293 -> [w2305]
            tunnel: w2292 -> [w2304]
            tunnel: w2296 -> [w2298]
            tunnel: [w2306] -> w2294
            tunnel: [w2300] -> w2295
            stop <- w2307 stop-if-true
            n1496 = local read "stop"() -> (w2307:bool)
            n1497 = call <vilib>:"IMAQdx Grab.vi"("error in"=w2304, "Image In"=w2298, "Session In"=w2305) -> ("error out"=w2300:errorcluster, "Image Out"=w2299:T8, "Session Out"=w2306:T11)  [unwired: 5 in, 1 out]
            n1498 = call "imageQ_camera_hook.vi"("Image"=w2299) -> ()  [unwired: 11 in]
            n1499 = feedback #13() -> (w2302:T34)  [unwired: 1 in]
            n1500 = call "Smoothed Frame Rate.vi"("Feedback In"=w2302) -> ("Feedback Out"=w2303:T34, "Frame Rate"=w2301:dbl)  [unwired: 1 in, 4 out]
            n1501 = feedback-in #13(w2303) -> ()
            n1502 = global write "red_tweezers_globals_INTERNAL_VOLATILE.vi" "Video Frame Rate"(w2301) -> ()
          }
          n1503 = call <vilib>:"IMAQdx Close Camera.vi"("error in"=w2295, "Session In"=w2294) -> ()  [unwired: 9 in, 1 out]
        }
        frame condition #2 {
          # "This subdiagram acquires using the IMAQdx drivers.  This covers most FireWire and GigE cameras (at least the ones supporting the IIDC or GenICam standards)."
          n1504 = call <vilib>:"IMAQdx Open Camera.vi"("Session In"="Camera") -> ("error out"=w2319:errorcluster, "Session Out"=w2318:T11)  [unwired: 9 in]
          n1505 = call <vilib>:"IMAQdx Configure Grab.vi"("error in"=w2319, "Session In"=w2318) -> ("error out"=w2315:errorcluster, "Session Out"=w2316:T11)  [unwired: 8 in]
          n1506 = call "IMAQ Create"("Image Name"="Red Tweezers live image") -> ("New Image"=w2313:T8)  [unwired: 3 in, 2 out]
          n1507 = call "IMAQdx_get_ROI.vi"("Session In"=w2316) -> ("ROI"=w2312:u32[], "Session Out"=w2314:T11)  [unwired: 8 in]
          n1508 = while {
            shift-right: [w2328] -> w2308
            shift-left: w2315 -> [w2329]
            shift-right: [w2325] -> w2309
            shift-left: w2314 -> [w2326]
            tunnel: w2313 -> [w2324]
            tunnel: w2312 -> [w2323]
            tunnel: w2311 -> [w2322]
            tunnel: [w2321] -> w2310
            stop <- w2335 stop-if-true
            n1509 = event shown="[0] Timeout" {
              selector: _ -> [_ _ _]
              dyn-events: _ -> [_ _ _]
              timeout: 0 -> [_ _ _]
              tunnel: w2329 -> [w2342 w2349 w2364]
              tunnel: [w2341 w2349 w2364] -> w2328
              tunnel: w2326 -> [w2340 w2350 w2365]
              tunnel: [w2339 w2350 w2365] -> w2325
              tunnel: w2324 -> [w2338 _ _]
              tunnel: w2323 -> [w2337 _ _]
              tunnel: w2322 -> [_ w2348 w2363]
              event Timeout {
                w2336 = 0  # timeout in ms
                # "Use a timeout of a few hundred ms if you want to acquire just fast enough to update the image- or a timeout of zero to run the camera at full speed."
                # "This VI sends the image to the loop above for display.\nIt's better to do this than to display here, because it separates the camera loop from the front panel a bit, and increases speed without sacrificing responsiveness of the UI.  Of course, using the event structure removes some of those benefits- but it is possible to write a high-performance camera loop with fast particle tracking, and still use this mechanism to display images without slowing down acquisition."
                # "If we're not dealing with other events, acquire from the camera."
                n1510 = event-data() -> ("Time"=w2347:u32)  [unwired: 1 in]
                n1511 = call <vilib>:"IMAQdx Grab.vi"("error in"=w2342, "Image In"=w2338, "Session In"=w2340) -> ("error out"=w2341:errorcluster, "Image Out"=w2344:T8, "Session Out"=w2339:T11)  [unwired: 5 in, 1 out]
                n1512 = call "IMAQ Clear Overlay"("Image"=w2344) -> ("Image Out"=w2343:T8)  [unwired: 9 in, 1 out]
                n1513 = Multiply(x=w2347, y=u32 1000) -> (x*y=w2345:u32)
                n1514 = call "imageQ_camera_hook.vi"("timeout in ms (0=don't wait if there are no requests)"=w2336, "Timestamp/us"=w2345, "ROI"=w2337, "Image"=w2343) -> ()  [unwired: 8 in]
              }
              event "Draw ROI", "Zoom": Value Change {
                # "This changes the current mouse mode on the image, allowing zooming/drawing of ROI (which can be useful if you want to window down a camera for particle tracking)."
                n1515 = event-data() -> ("CtlRef"=w2355:refnum<vi>)  [unwired: 1 in]
                n1516 = control-ref of="Draw ROI"() -> (w2356:refnum<vi>)
                n1517 = Equal?(x=w2356, y=w2355) -> (x = y?=w2354:bool)
                n1518 = case shown="True" w2354 {
                  tunnel: [w2359 w2362] -> w2353
                  tunnel: [TRUE ("stop") FALSE ("stop")] -> w2351
                  tunnel: [FALSE ("Update Indicators?") TRUE ("Update Indicators?")] -> w2352
                  frame False {
                    w2359 = u32 8 items=["Zoom Tool"=8, "Selection Tool"=0, "Pan Tool"=9, "Point Tool"=1, "Line Tool"=2, "Rectangle Tool"=3, "Rotated Rectangle Tool"=12, "Polyline Tool"=10, "Polygon Tool"=5, "Freehand Tool"=11, "Closed Freehand Tool"=6, "Ellipse Tool"=4, "Annulus Tool"=7] ("Current ROI Tool")
                  }
                  frame True {
                    w2362 = u32 3 items=["Zoom Tool"=8, "Selection Tool"=0, "Pan Tool"=9, "Point Tool"=1, "Line Tool"=2, "Rectangle Tool"=3, "Rotated Rectangle Tool"=12, "Polyline Tool"=10, "Polygon Tool"=5, "Freehand Tool"=11, "Closed Freehand Tool"=6, "Ellipse Tool"=4, "Annulus Tool"=7] ("Current ROI Tool")
                  }
                }
                n1519 = local write "Draw ROI"(w2352) -> ()
                n1520 = local write "Zoom"(w2351) -> ()
                n1521 = property on="Property Node" class="ImageControl"(reference=w2348, "Current ROI Tool"=w2353) -> ()  [unwired: 1 in, 2 out]
              }
              event "Zoom to Fit": Value Change {
                # "The various ROI tools are hidden, so the image control resizes nicely as the Red Tweezers window is resized.  The zoom to fit button/mouse mode buttons return some of this functionality."
                n1522 = event-data() -> ("NewVal"=w2366:bool)  [unwired: 1 in]
                n1523 = property on="Property Node" class="ImageControl"(reference=w2363, "Zoom to Fit Mode"=w2366) -> ()  [unwired: 1 in, 2 out]
              }
            }
            n1524 = feedback #14() -> (w2334:T34)  [unwired: 1 in]
            n1525 = call "Smoothed Frame Rate.vi"("Feedback In"=w2334, "Alpha"=0.05) -> ("Feedback Out"=w2333:T34, "Frame Rate"=w2330:dbl)  [unwired: 4 out]
            n1526 = feedback-in #14(w2333) -> ()
            n1527 = global write "red_tweezers_globals_INTERNAL_VOLATILE.vi" "Video Frame Rate"(w2330) -> ()
            n1528 = local read "stop"() -> (w2331:bool)
            n1529 = Unbundle By Name(w2328) -> ("status"=w2321:bool)
            n1530 = Or(x=w2321, y=w2331) -> (x .or. y?=w2335:bool)
          }
          n1531 = call <vilib>:"IMAQdx Close Camera.vi"("error in"=w2308, "Session In"=w2309) -> ()  [unwired: 9 in, 1 out]
        }
        frame condition #3 (active) {
          w2368 = 0 ("element")
          w2370 = 1920 ("dimension size")
          w2369 = 1080 ("dimension size")
          w2371 = T19 0 items=["Grayscale (U8)", "Grayscale (I16)", "Grayscale (SGL)", "Complex (CSG)", "RGB (U32)", "HSL (U32)", "RGB (U64)", "Grayscale (U16)"] ("Image Type")
          (unwired) FALSE ("background subtraction")
          # "This subdiagram generates a blank white image- useful if you don't have a camera"
          n1532 = Build Array(w2368, w2368, w2370, w2369) -> (w2367:i32[])
          n1533 = Initialize Array(u8 255 ("element"), w2369, w2370) -> (w2372:u8[][])
          n1534 = global write "red_tweezers_globals_INTERNAL.vi" "Global ROI"(w2367) -> ()
          n1535 = call "IMAQ Create"("Image Name"="red tweezers camera stub", "Image Type"=w2371) -> ("New Image"=w2373:T8)  [unwired: 2 in, 2 out]
          n1536 = call "IMAQ ArrayToImage"("Image Pixels (U8)"=w2372, "Image"=w2373) -> ("Image Out"=w2376:T8)  [unwired: 8 in, 1 out]
          n1537 = call "IMAQ Create"("Image Name"="Red Tweezers live image") -> ("New Image"=w2377:T8)  [unwired: 3 in, 2 out]
          n1538 = while {
            tunnel: w2376 -> [w2380]
            tunnel: w2377 -> [_]
            stop <- w2384 stop-if-true
            n1539 = local read "stop"() -> (w2384:bool)
            n1540 = Wait Until Next ms Multiple(millisecond multiple=u32 20) -> ()  [unwired: 1 out]
            n1541 = call "imageQ_camera_hook.vi"("Image"=w2380) -> ()  [unwired: 11 in]
            n1542 = feedback #15() -> (w2382:T34)  [unwired: 1 in]
            n1543 = call "Smoothed Frame Rate.vi"("Feedback In"=w2382) -> ("Feedback Out"=w2383:T34, "Frame Rate"=w2381:dbl)  [unwired: 1 in, 4 out]
            n1544 = feedback-in #15(w2383) -> ()
            n1545 = global write "red_tweezers_globals_INTERNAL_VOLATILE.vi" "Video Frame Rate"(w2381) -> ()
          }
        }
        frame condition #4 {
          # "Use this subdiagram if you have an external camera VI which writes to the image queue (using imageQ_camera_hook.vi)"
        }
        frame condition #5 {
          w2385 = path "C:/Users/Tweezer Cube/Desktop/red_tweezers_1_4_rc0/camera_for_rt136.llb/Particle Tracking.vi"  # Path to camera VI
          # "Use this subdiagram if you have an external camera VI which writes to the image queue (using imageQ_camera_hook.vi).  This is the slightly more sophisticated version, which checks that said external VI is running, and runs it if not."
          n1546 = Open VI Reference(vi path=w2385) -> (vi reference=w2386:refnum<vi>, error out=w2388:errorcluster)  [unwired: 5 in]
          n1547 = property class="VI"(reference=w2386) -> ("Path"=w2387:path)  [unwired: 1 in, 2 out]
          n1548 = global write "red_tweezers_globals_INTERNAL_VOLATILE.vi" "Current Camera VI"(w2387) -> ()
          n1549 = property class="VI"(reference=w2386, error in=w2388) -> (reference out=w2393:refnum<vi>, error out=w2392:errorcluster, "Exec.State"=w2390:T36)
          n1550 = Equal?(x=w2390, y=T36."Idle") -> (x = y?=w2394:bool)
          n1551 = case shown="True" w2394 {
            tunnel: w2393 -> [w2398 w2407]
            tunnel: w2392 -> [w2397 w2404]
            tunnel: [w2396 w2403] -> w2389
            tunnel: w2390 -> [w2400 _]
            frame False {
              n1552 = Close Reference(reference=w2398, error in (no error)=w2397) -> (error out=w2396:errorcluster)
              n1553 = Equal?(x=w2400, y=T36."Bad") -> (x = y?=w2399:bool)
              n1554 = case shown="False" w2399 {
                frame False {
                }
                frame True {
                  n1555 = One Button Dialog(message="The external camera VI is not running and cannot be started- it's probably broken or missing.  Check the static/dynamically loaded VI reference in the bottom loop on the block diagram.") -> ()  [unwired: 1 in, 1 out]
                }
              }
            }
            frame True {
              n1556 = invoke class="VI" method="Run VI"(reference=w2407, error in=w2404, "Wait until done"=FALSE ("Wait Until Done"), "Auto Dispose Ref"=TRUE ("Auto Dispose Reference")) -> (error out=w2403:errorcluster)  [unwired: 1 in, 4 out]
            }
          }
          n1557 = call <vilib>:"Simple Error Handler.vi"("error source (\" \")"="External camera VI (see the bottom loop in the block diagram)" ("error source (\" \")"), "error in (no error)"=w2389) -> ()  [unwired: 3 in, 5 out]
        }
      }
    }
  }
  n1558 = while {
    tunnel: w9 -> [w2425]
    shift-right: [w2424] -> w8
    shift-left: w10 -> [w2426]
    shift-right: [w2421] -> _
    shift-left: _ -> [w2414]
    shift-right: [w2420] -> _
    shift-left: _ -> [w2418]
    shift-right: [w2419] -> _
    shift-left: FALSE ("Saving") -> [w2415]
    stop <- w2423 stop-if-true
    w2412 = u32 50 ("millisecond multiple")
    # "Start/stop saving data, if necessary"
    n1559 = Divide(x=u32 1000, y=w2412) -> (x/y=w2410:dbl)
    n1560 = Wait Until Next ms Multiple(millisecond multiple=w2412) -> ()  [unwired: 1 out]
    n1561 = call "imageQ_dequeue.vi"("timeout in ms (-1)"=2000, "Return queue"=w2426, "Image Dst"=w2425) -> ("Timestamp/us"=w2416:u64, "Return queue out"=w2424:refnum<queue>, "Image Dst Out"=w2427:T8, "timed out?"=w2430:bool, "ROI"=w2409:u64[])  [unwired: 4 in]
    n1562 = Not(x=w2430) -> (.not. x?=w2428:bool)
    n1563 = case shown="True" w2428 {
      tunnel: w2427 -> [_ w2464]
      tunnel: w2418 -> [w2457 w2467]
      tunnel: w2415 -> [_ w2461]
      tunnel: [w2457 w2462] -> w2417
      tunnel: w2416 -> [_ w2465]
      tunnel: w2414 -> [w2458 w2466]
      tunnel: [w2458 w2463] -> w2413
      tunnel: w2409 -> [_ w2460]
      frame False {
      }
      frame True {
        n1564 = global read "red_tweezers_globals_INTERNAL.vi" "Image Overlay (extras from control loop)"() -> (w2475:T21[])
        n1565 = case shown="True" w2461 {
          tunnel: w2467 -> [w2476 w2478]
          tunnel: w2466 -> [w2477 w2484]
          tunnel: w2465 -> [_ w2483]
          tunnel: w2464 -> [_ w2482]
          tunnel: [w2477 w2481] -> w2463
          tunnel: [w2476 w2480] -> w2462
          frame False {
          }
          frame True {
            n1566 = call "save_data_save.vi"("Image"=w2482, "Timestamp"=w2483, "Avi Refnum"=w2478, "Data refnum"=w2484) -> ("error out"=w2479:errorcluster, "Avi Refnum (duplicate)"=w2480:T37, "Data refnum (duplicate)"=w2481:refnum<file>)  [unwired: 5 in]
            n1567 = case shown="Error" w2479 {
              selector: w2479 -> [_ w2486]
              frame No Error {
              }
              frame Error {
                n1568 = call <vilib>:"Clear Errors.vi"("error in (no error)"=w2486) -> ()  [unwired: 5 in, 2 out]
                n1569 = local write "Save Video"(FALSE ("Save")) -> ()
              }
            }
          }
        }
        n1570 = global write "red_tweezers_globals_INTERNAL.vi" "Global ROI"(w2460) -> ()
        n1571 = global read "red_tweezers_globals_INTERNAL_VOLATILE.vi" "Tracked Spot Positions (3D)"() -> (w2468:cluster{"x":dbl, "y":dbl, "Z":dbl}[])
        n1572 = global read "red_tweezers_globals.vi" "Selection/Group"() -> (w2474:T12[])
        n1573 = global read "red_tweezers_globals.vi" "Spots"() -> (w2473:T3[])
        n1574 = call "overlay_positions.vi"("Positions"=w2468, "Image"=w2464) -> ("Image 2"=w2470:T8)  [unwired: 9 in]
        n1575 = call "render_overlay_elements.vi"("Image Overlay (extras from control loop)"=w2475, "Image"=w2470) -> ("Image Out"=w2472:T8)  [unwired: 5 in]
        n1576 = call "grid_and_guides.vi"("Operation"=T16."Render on image", "Image"=w2472) -> ("Image Out"=w2459:T8)  [unwired: 9 in]
        n1577 = call "overlay_spots_on_image.vi"("Selection and Groups"=w2474, "Spots"=w2473, "image"=w2459) -> ("Image"=→"Image":T8)  [unwired: 3 in, 1 out]
      }
    }
    n1578 = global read "red_tweezers_globals_INTERNAL_VOLATILE.vi" "Video Frame Rate"() -> (→"Video Frame Rate":dbl)
    n1579 = case shown="False" "Save Video" {
      tunnel: [w2433 w2448] -> w2421
      tunnel: [w2432 w2442] -> w2420
      tunnel: [FALSE ("Saving") w2447] -> w2419
      tunnel: w2415 -> [w2436 w2446]
      tunnel: w2417 -> [w2434 w2445]
      tunnel: w2413 -> [w2435 w2444]
      tunnel: w2410 -> [_ w2443]
      frame False {
        n1580 = case shown="True" w2436 {
          tunnel: w2435 -> [w2438 w2441]
          tunnel: w2434 -> [w2437 w2440]
          tunnel: [w2438 _] -> w2433
          tunnel: [w2437 _] -> w2432
          frame False {
          }
          frame True {
            n1581 = local write "Save Video"(FALSE ("Save")) -> ()
            n1582 = call "save_data_stop.vi"("Avi Refnum"=w2440, "Data refnum"=w2441) -> ()  [unwired: 10 in]
          }
        }
      }
      frame True {
        n1583 = case shown="False" w2446 {
          selector: w2446 -> [_ w2456]
          tunnel: [w2453 w2454] -> w2448
          tunnel: [w2452 w2455] -> w2442
          tunnel: [w2449 w2456] -> w2447
          tunnel: w2445 -> [_ w2455]
          tunnel: w2444 -> [_ w2454]
          tunnel: w2443 -> [w2451 _]
          frame False {
            n1584 = call "save_data_start.vi"("Save Video"=TRUE, "Frames Per Second"=w2451) -> ("Saving"=w2449:bool, "Avi Refnum"=w2452:T37, "Data Refnum"=w2453:refnum<file>)  [unwired: 3 in]
            n1585 = local write "Save Video"(w2449) -> ()
          }
          frame True {
          }
        }
      }
    }
    n1586 = local read "stop"() -> (w2423:bool)
  }
  n1587 = Release Queue(queue=w8) -> ()  [unwired: 2 in, 3 out]
  n1588 = case shown="True" w3 {
    frame False {
    }
    frame True {
      n1589 = One Button Dialog(message="Warning: there was a camera error.  You may need to restart Red Tweezers.") -> ()  [unwired: 1 in, 1 out]
    }
  }
  n1590 = flat-sequence {
    tunnel: w18 -> [w2492]
    tunnel: w17 -> [_]
    frame #0 {
      # "This autosaves when we stop.  The sequence structures are necessary so that:\n1. loading settings doesn't stop the VI\n2. plugins are still open (and hence saved) when we save settings"
      n1591 = local read "Plugins"() -> (w2495:T5)
      n1592 = global read "red_tweezers_globals_INTERNAL_VOLATILE.vi" "Current Settings File"() -> (w2489:path)
      n1593 = global read "red_tweezers_globals_INTERNAL_VOLATILE.vi" "Save Settings On Exit"() -> (w2488:bool)
      n1594 = flat-sequence {
        tunnel: w2492 -> [w2498]
        tunnel: [w2498] -> w2491
        frame #0 {
          n1595 = local write "stop"(FALSE ("STOP")) -> ()
        }
      }
      n1596 = case shown="True" w2488 {
        tunnel: w2489 -> [_ w2503]
        tunnel: w2491 -> [w2500 w2501]
        tunnel: [w2500 w2501] -> w2490
        frame False {
        }
        frame True {
          n1597 = Path To String(path=w2503) -> (string=w2502:string)
          n1598 = call "settings_save_to_file.vi"("XML File Path"=w2503) -> ()  [unwired: 11 in]
          n1599 = call "settings_filename_to_registry.vi"("Last Used Settings File"=w2502) -> ()  [unwired: 11 in]
        }
      }
      n1600 = flat-sequence {
        tunnel: w2490 -> [w2496]
        tunnel: [w2496] -> _
        frame #0 {
          n1601 = local write "stop"(TRUE ("STOP")) -> ()
        }
      }
      n1602 = control-ref of="Plugin Pnl"() -> (w2493:refnum<vi>)
      n1603 = control-ref of="Plugin:"() -> (w2494:refnum<vi>)
      n1604 = call "plugins_unload.vi"("error in (no error)"=w2490, "Plugins"=w2495, "Sub Panel"=w2493, "Plugin Chooser"=w2494) -> ()  [unwired: 2 in, 2 out]
    }
  }
